vi "VR Controler 9.2.vi"() -> ()   [LabVIEW 2017]
uses:
  Sub VIs/Record enum.ctl
  Sub VIs/Socket enum.ctl
  Sub VIs/Main program enum2.ctl
  <vilib>/vision/Image Controls.llb/IMAQ Image.ctl
  e2139745-3a2d-4eca-8046-712b838de117.vi
  c1239b79-c935-4849-aa75-a73d195e7430.vi
  674a1914-568f-4f25-b0a8-01d8120e0c5f.vi
  5779e0b0-41b7-4506-a67f-138f79383ca8.vi
  75927e18-e53a-4ccd-922e-dca7ab16e00a.vi
  6c211394-beff-4d45-9cac-85fa7b8fa806.vi
  b426bb1a-86ec-4bb9-bfac-d02472307ceb.vi
  58126b9d-de85-4f5f-a9a7-01a9de38026e.vi
  6235507b-2202-4f21-86ca-b7b41428e472.vi
  835dcb76-40d0-41c5-8fe3-3989c1fd9891.vi
  7e58093c-c06d-4417-bc89-98900abbef57.vi
  280f3af5-b849-4305-b59e-3cd99654dfd1.vi
  378bb8a1-48c3-4ad7-89e2-98d14b258fa1.vi
  4796a129-a1f4-4c2b-9c8a-39875efc01cf.vi
  <vilib>/DAQmx/write.llb/DAQmx Write (Digital Bool 1Line 1Point).vi
  bf4008ee-ae26-4c0a-87de-22156137ce73.vi
  cfabecd4-7210-4e1d-87ea-acbfc879dca4.vi
  ec3ac053-eb45-4274-a63b-aef392164dd0.vi
  c7e8f878-57a8-404b-b967-73b810e59910.vi
  b14711bf-09ac-44ea-973e-d3b9cd6138c5.vi
  839eb35e-605d-4d61-b8d1-8b601b76a39a.vi
  1da1cb31-40b1-4a67-a7e6-56ad72bdf787.vi
  eb595f88-4225-414f-83f1-01d5d940fc66.vi
  fb6b5c9d-106e-453b-a883-cc93056fac18.vi
  4b664865-0372-4337-9de9-faa9f3913aab.vi
  63df5311-9246-4ffc-851f-b70ac2e65be5.vi
  <vilib>/DAQmx/read.llb/DAQmx Read (Analog 2D DBL NChan NSamp).vi
  <vilib>/DAQmx/read.llb/DAQmx Read (Digital 2D U8 NChan NSamp).vi
  <vilib>/DAQmx/read.llb/DAQmx Read (Counter 1D DBL 1Chan NSamp).vi
  <vilib>/DAQmx/create/channels.llb/DAQmx Create Channel (DO-Digital Output).vi
  <vilib>/Utility/file.llb/Read Delimited Spreadsheet (string).vi
  <vilib>/DAQmx/create/channels.llb/DAQmx Create Channel (AI-Voltage-Basic).vi
  <vilib>/DAQmx/create/channels.llb/DAQmx Create Channel (DI-Digital Input).vi
  <vilib>/DAQmx/configure/timing.llb/DAQmx Timing (Sample Clock).vi
  <vilib>/DAQmx/miscellaneous.llb/DAQmx Fill In Error Info.vi
  <vilib>/Utility/file.llb/Write Delimited Spreadsheet (string).vi
  <vilib>/DAQmx/create/channels.llb/DAQmx Create Channel (CO-Pulse Generation-Frequency).vi
  <vilib>/DAQmx/configure/timing.llb/DAQmx Timing (Implicit).vi
  6f1d6b9c-7e66-4bfa-a54a-0bf9111e914d.vi
  <resource>/objmgr/daqmx.rc
  f0a6b648-ccd6-4e98-b62c-d3930b5e7adb.vi
  <vilib>/vision/driver/NI_Vision_Acquisition_Software.lvlib
  fa866b4b-dc6c-4481-bc67-f1512cbbaaf9.vi
  <vilib>/DAQmx/configure/task.llb/DAQmx Configure Logging (TDMS).vi
panel:
  out "Write loop stopped":bool
  out "Read loop stopped":bool
  in  "VR Controller":T1(tab)
  in  "Timed reward (s)":u32
  in  "Various GUI elements":T2(tab)
  out "Saved 2P signals":string[][](table)
  in  "Record 2P":bool
  out "Frame signal 1 rec.":bool
  out "Frame signal 2 rec.":bool
  in  "Start trigger":bool
  in  "Stop triggers":bool
  out "Boolean 2":bool
  out "Boolean 3":bool
  out "Opt stim command":dbl[](graph)
  out "stim loop rate":dbl
  in  "start with ramp":bool
  out "Next trial stim. protocol":string
  out "Current stim. protocol":string
  in  "Stimulus cut off (s)":u32=15
  out "Laser ON":bool
  in  "Enable stim.":bool
  out "Saved optogen. signals":string[][](table)
  out "Pupille image saved":bool
  in  "Record Button 2":bool
  in  "Black Level":dbl(slide)=0.9896907216494839 min=-32.0 max=31.75 step=1.0 scale=-32.0..32.0
  in  "Gain":dbl(slide)=8.879999999999999 min=0.0 max=24.0 step=1.0 scale=0.0..24.0
  in  "Exposure Time (ms)":dbl(slide)=15144.329896907217 min=1.0 max=15.0 scale=0.0..15.0
  in  "Target frame rate":dbl=60.0 min=1.0 max=144.0 step=1.0
  out "Pupille image":T3(plugin-control)
  out "Frame rate":dbl
  in  "Image Format Control::Offset X":i64(slide) min=0 max=450 step=2 scale=0.0..450.0
  in  "Image Format Control::Offset Y":i64(slide) min=0 max=350 step=2 scale=0.0..350.0
  out "Lost Image Count":u32
  out "Total Images Transferred":u32
  out "Saved pupil imaging signals":string[][](table)
  out "EyeCam frame signal rec.":bool
  out "Security cam image":T3(plugin-control)
  in  "Cam ON /OFF":bool
  out "Random start pos":bool=TRUE
  in  "VR start pos":T4(ring)
  out "Behavior and VR signals saved":string[][](table)
  out "Stim. count":i32
  in  "Random reward":bool
  in  "Hybrid licking":bool
  in  "Boolean":bool
  in  "Comment":string
  out "Photodiode":bool
  out "Trial type ettings":enum32{"Page 1", "Page 2"}(tab)
  in  "Auto stop recording":bool
  in  "Shuffle stim trials":bool
  out "Session length":u16 max=100
  in  "Block num. 5":u16
  in  "Block 5":u16(ring) items=["Context J", "Context K (rew same as J)", "Context L", "Context M", "Context N (rew same as J)", "Context O"]
  in  "Block num. 4":u16
  in  "Block 4":u16(ring) items=["Context J", "Context K (rew same as J)", "Context L", "Context M", "Context N (rew same as J)", "Context O"]
  in  "Block num. 3":u16
  in  "Block 3":u16(ring) items=["Context J", "Context K (rew same as J)", "Context L", "Context M", "Context N (rew same as J)", "Context O"]
  in  "Block num. 2":u16
  in  "Block 2":u16(ring) items=["Context J", "Context K (rew same as J)", "Context L", "Context M", "Context N (rew same as J)", "Context O"]
  in  "Block num. 1":u16=1 min=1
  in  "Block 1":u16(ring) items=["Context J", "Context K (rew same as J)", "Context L", "Context M", "Context N (rew same as J)", "Context O"]
  in  "stim. num. 5":u16
  in  "Stim. prot 5":u16(ring) items=["none", "none", "continuous from 0 to 150 int. 100 % duty cycle 0 %", "20 Hz sinus from 0 to 150 int. 100 % duty cycle 0 %", "20 Hz sinus from 10 to 20 int. 100 % duty cycle 0 %", "20 Hz sinus from 10 to 70 int. 100 % duty cycle 0 %", "20 Hz sinus from 10 to 0 int. 100 % duty cycle 0 %", "20 Hz sinus from 0 to 70 int. 100 % duty cycle 0 %", "20 Hz sinus from 0 to 70 int. 50 % duty cycle 0 %", "continuous from 10 to 70 int. 100 % duty cycle 0 %"]
  in  "stim. num. 4":u16
  in  "Stim. prot 4":u16(ring) items=["none", "none", "continuous from 0 to 150 int. 100 % duty cycle 0 %", "20 Hz sinus from 0 to 150 int. 100 % duty cycle 0 %", "20 Hz sinus from 10 to 20 int. 100 % duty cycle 0 %", "20 Hz sinus from 10 to 70 int. 100 % duty cycle 0 %", "20 Hz sinus from 10 to 0 int. 100 % duty cycle 0 %", "20 Hz sinus from 0 to 70 int. 100 % duty cycle 0 %", "20 Hz sinus from 0 to 70 int. 50 % duty cycle 0 %", "continuous from 10 to 70 int. 100 % duty cycle 0 %"]
  in  "stim. num. 3":u16
  in  "Stim. prot 3":u16(ring) items=["none", "none", "continuous from 0 to 150 int. 100 % duty cycle 0 %", "20 Hz sinus from 0 to 150 int. 100 % duty cycle 0 %", "20 Hz sinus from 10 to 20 int. 100 % duty cycle 0 %", "20 Hz sinus from 10 to 70 int. 100 % duty cycle 0 %", "20 Hz sinus from 10 to 0 int. 100 % duty cycle 0 %", "20 Hz sinus from 0 to 70 int. 100 % duty cycle 0 %", "20 Hz sinus from 0 to 70 int. 50 % duty cycle 0 %", "continuous from 10 to 70 int. 100 % duty cycle 0 %"]
  in  "stim. num. 2":u16
  in  "Stim. prot 2":u16(ring) items=["none", "none", "continuous from 0 to 150 int. 100 % duty cycle 0 %", "20 Hz sinus from 0 to 150 int. 100 % duty cycle 0 %", "20 Hz sinus from 10 to 20 int. 100 % duty cycle 0 %", "20 Hz sinus from 10 to 70 int. 100 % duty cycle 0 %", "20 Hz sinus from 10 to 0 int. 100 % duty cycle 0 %", "20 Hz sinus from 0 to 70 int. 100 % duty cycle 0 %", "20 Hz sinus from 0 to 70 int. 50 % duty cycle 0 %", "continuous from 10 to 70 int. 100 % duty cycle 0 %"]
  in  "stim. num. 1":u16 min=1
  in  "Stim. prot 1":u16(ring) items=["none", "none", "continuous from 0 to 150 int. 100 % duty cycle 0 %", "20 Hz sinus from 0 to 150 int. 100 % duty cycle 0 %", "20 Hz sinus from 10 to 20 int. 100 % duty cycle 0 %", "20 Hz sinus from 10 to 70 int. 100 % duty cycle 0 %", "20 Hz sinus from 10 to 0 int. 100 % duty cycle 0 %", "20 Hz sinus from 0 to 70 int. 100 % duty cycle 0 %", "20 Hz sinus from 0 to 70 int. 50 % duty cycle 0 %", "continuous from 10 to 70 int. 100 % duty cycle 0 %"]
  out "Stim array length":u16 max=500
  in  "Masking light":T5(ring)
  out "GUI version":enum32{"Page 1", "Page 2"}(tab)
  in  "plot selector 1":u16(ring) items=["Context J", "Context K (rew same as J)", "Context L", "Context M", "Context N (rew same as J)", "Context O"]
  out "?":dbl(slide) scale=0.0..250.0
  in  "Reset top plot":bool=TRUE caption="Reset"
  in  "Reset bottom plot":bool=TRUE caption="Reset"
  out "P stim. Hit":dbl(slide) scale=0.0..1.0
  out "P ctrl. Hit":dbl(slide) scale=0.0..1.0
  out "Control hit trials %":dbl
  out "Stim. hit trials %":dbl
  out "Top Graph":cluster{"Y":dbl[], "Y":dbl[]}[](graph) caption="XY Graph"
  out "Bottom Graph":cluster{"Y":dbl[], "Y":dbl[]}[](graph) caption="XY Graph"
  in  "plot selector bool 1":bool
  in  "plot selector 2":u16(ring) items=["Context J", "Context K (rew same as J)", "Context L", "Context M", "Context N (rew same as J)", "Context O"]
  in  "plot selector bool 2":bool
  out "Hit trials %":dbl format="%#.1g"
  out "Hit trials":i32
  out "Wheel position graph":cluster{"Y":dbl[], "Y":dbl[]}[](graph) caption="XY Graph"
  in  "Reset wheel pos. graph":bool=TRUE caption="Reset"
  out "P hit trials":dbl(slide) scale=0.0..1.0
  out "%":dbl format="%#_3g"
  in  "Weight":dbl
  in  "Lab book notes":string
  in  "Open valve":bool
  in  "Reward freq. (cm)":u32
  in  "Reward zone":bool
  out "Distance (m)":dbl format="%#.2g"
  in  "Record Button":bool
  in  "Reset water count":bool
  out "Water received (ul)":dbl
  out "All trials":i32
  out "Ctrl. count":i32
  out "Unique ID":i8 format="%2d"
  in  "Stop recording":bool
  in  "Start recording":bool
  out "Laps":i32
  in  "Exit program":bool
  in  "counter reset (F)":bool caption="stop (F)"
  out "Position on the wheel":dbl(knob) scale=0.0..157.0
  in  "Give reward":bool
  in  "Repetition":i32
  out "Date":string
  out "Run experiment":bool
  out "Velocity chart":dbl(graph)
  out "Lick and reward chart":cluster{dbl, i16}(graph)
  out "Record":bool
  out "Time (min)":dbl format="%#.2g"
  in  "Active licking":bool
  in  "Mouse name":u16(ring) items=["-", "m8134-MN7", "m8135-NL1", "m8136-NL3", "m8137-MN8", "m8138-NL7", "m8139-X2", "m8140-MN6", "m8141-NL8", "m8142-NL6", "m8143-X", "m8144-NL4", "-", "-", "-", "-", "-", "test-xx", "train-NLX", "-"]
  out "Tab Control hidden Variables":enum32{"Test charts", "Variables"}(tab)
  in  "Ring 4":u16(ring) items=["Encoder signal", "Photo-diode", "Distance (cm)", "Position in Unity", "Valve open", "Lick signal", "Analog lick signal", "VR context", "VR gain", "Frame signal", "Frame signal 2", "EyeCam frame signal", "Analog input 3", "Photo stimulus signal", "Masking light signal", "Stimulus protocol", "Analog input 5"]
  out "Waveform Chart 4":dbl[](graph)
  in  "Ring 3":u16(ring) items=["Encoder signal", "Photo-diode", "Distance (cm)", "Position in Unity", "Valve open", "Lick signal", "Analog lick signal", "VR context", "VR gain", "Frame signal", "Frame signal 2", "EyeCam frame signal", "Analog input 3", "Photo stimulus signal", "Masking light signal", "Stimulus protocol", "Analog input 5"]
  out "Waveform Chart 3":dbl[](graph)
  in  "Ring 2":u16(ring) items=["Encoder signal", "Photo-diode", "Distance (cm)", "Position in Unity", "Valve open", "Lick signal", "Analog lick signal", "VR context", "VR gain", "Frame signal", "Frame signal 2", "EyeCam frame signal", "Analog input 3", "Photo stimulus signal", "Masking light signal", "Stimulus protocol", "Analog input 5"]
  out "Waveform Chart 2":dbl[](graph)
  in  "Ring":u16(ring) items=["Encoder signal", "Photo-diode", "Distance (cm)", "Position in Unity", "Valve open", "Lick signal", "Analog lick signal", "VR context", "VR gain", "Frame signal", "Frame signal 2", "EyeCam frame signal", "Analog input 3", "Photo stimulus signal", "Masking light signal", "Stimulus protocol", "Analog input 5"]
  out "Waveform Chart":dbl[](graph)
  in  "VR Gain":dbl
  out "Frame signal 2":i8[](array[numeric])
  out "corridor lengths":i32[](array[numeric])
  out "zeward zones":i16[][](array[numeric])
  out "teleports":i16[](array[numeric])
  out "Stim prot command":u16
  out "Context command":u16
  out "ML signal":sgl[](array[numeric])
  out "Pupil Exp day folder":path
  out "settings folder":path
  out "Eyecam states":T6(ring)
  in  "Eable security cam":bool
  out "Eye cam frame signal":i8[](array[numeric])
  out "prev. max stim. V":dbl
  out "prev. stim. type":string
  out "protocol array":string[][](array[string])
  out "analog lick":sgl[](array[numeric])
  out "Encoder signal":sgl[](array[numeric])
  out "Photo stimulus signal":sgl[](array[numeric])
  out "SciScan start":refnum<k21>
  out "Valve signal":i8[](array[numeric])
  out "Trials in session array":u16[][](array[numeric])
  out "Photodiode signal":sgl[](array[numeric])
  out "Frame signal":i8[](array[numeric])
  out "Filename":string
  out "Lab book file":path
  out "Lick indicator":dbl
  out "Encoder count":dbl
  out "Last saved reward size":dbl
  out "Stim types":u16[](array[numeric])
  out "shuffled array":i16[](array[numeric])
  out "Record loop state":T7
  in  "Record enum":T7
  out "Wheel circumference":dbl
  in  "Recording folder":path
  in  "command line":string
  in  "working directory":path=path ""
  out "Start time":u32
  out "Experiment time (ms)":u32
  out "delta time (s)":dbl format="%#.8g"
  out "reward zone end":dbl
  out "Sample rate":dbl
  out "Loop rate":dbl
  out "No. of smpl. per ch.":i32
  out "Original weight":dbl
  out "Laser stimulus calibration":string
  out "Stimulus protocol":string
  out "prev. diode position":dbl
  out "encoder ticks per rev":dbl
  out "Prev. rew. pos.":dbl
  out "Distance (cm)":dbl
  out "miss trial":bool
  out "Session start:":string
  out "hit trial":bool
  out "2P imaging":string
  out "Security camera":string
  out "velocity (cm/s)":dbl
  out "Masking light prot":string
  out "offset tag":string
  out "random rew":dbl
  out "Track position":sgl
  out "start of stim":bool
  in  "Eable eye cam":bool
  out "stim started":bool
  out "Context types":u16[](array[numeric])
  out "Reward given":u32
  out "current VR context":u16
  out "RZ available":bool
  out "User profile":string
  out "Stop Unity":bool
  out "Exit":bool
  out "Stim trial":bool
  out "Trial counted":bool
  in  "select trial":bool
  in  "VR Mode":bool
  out "delta distance cm":dbl[](array[numeric])
  in  "index":i32
  out "lick signal":i8[](array[numeric])
  out "msg tag":string
  out "Header":string
  out "Unity connected":bool
  out "Masking light":bool
  out "Lick":bool
  out "Valve open":bool
  in  "sound cue presented":bool
  out "read":bool
  out "Write":bool
  out "My tdms file":refnum<k34>
  out "Water cnt. reset":i32
  out "Store prev encoder count":dbl
  out "Start mask stim":bool
  out "Start light stim":bool
  out "Stop light stim":bool
  out "Light ON":bool
  out "Stop mask stim":bool
  out "Hit trials stim.":i32
  out "Hit trials ctrl.":i32
  in  "Software version":string
  out "total distance cm":sgl[](array[numeric])
  out "Experiment time (s)":dbl
  out "Analog 3":sgl[](array[numeric])
  out "Analog 5":sgl[](array[numeric])
  out "Signals to delete":i32[](array[numeric])
  out "channel names":string[](array[string])
  in  "working directory 2":path=path ""
  out "Mouse name 2":string
  out "Task config":string
  out "Saved signals":string
  out "Default vars text":string
  in  "Duty cycle (%)":u8=50 max=100 step=1
  out "Last calibration":string
  in  "Edit mouse list":bool
  out "Socket read loop rate (ms)":u32(graph)
  out "Recording loop rate  (ms)":u32(graph)
  in  "Sound duration (ms)":u32=25
  in  "Valve open dur. (ms)":u32=25
  in  "Reward size (ul)":dbl min=0.0 step=inf format="%#.2g"
  out "Reward read loop rate (ms)":u32(graph)
  in  "Current mice":string[][](array[string])
  out "Water count":i32
  in  "Stim protocols":u16(ring) items=["none", "none", "continuous from 0 to 150 int. 100 % duty cycle 0 %", "20 Hz sinus from 0 to 150 int. 100 % duty cycle 0 %", "20 Hz sinus from 10 to 20 int. 100 % duty cycle 0 %", "20 Hz sinus from 10 to 70 int. 100 % duty cycle 0 %", "20 Hz sinus from 10 to 0 int. 100 % duty cycle 0 %", "20 Hz sinus from 0 to 70 int. 100 % duty cycle 0 %", "20 Hz sinus from 0 to 70 int. 50 % duty cycle 0 %", "continuous from 10 to 70 int. 100 % duty cycle 0 %"]
  in  "Stim type":u16(ring) items=["none", "10 Hz sinus", "20 Hz sinus", "40 Hz sinus", "continuous", "10 Hz square", "20 Hz square", "40 Hz square"]
  in  "Intensity (%)":u8=100 max=100 step=1
  in  "stop (cm)":i32
  in  "start (cm)":i32
  in  "Select user profile":string(combo)
  in  "Default var. edit":string[][](array[string])
  in  "Path 2":path
  in  "Path":path
  out "Default variables":string[](array[string])
  out "Imaging ralated signals":string[](array[string])=["Encoder signal", "Photo-diode", "Distance (cm)", "Photo stimulus signal", "Position in Unity", "Valve open", "Lick signal", "Frame signal", "Stimulus protocol", "VR context", "Analog lick signal", "EyeCam frame signal", "Masking light signal", "Frame signal 2"]
  out "Behavior and task related signals":string[](array[string])=["Encoder signal", "Photo-diode", "Distance (cm)", "Photo stimulus signal", "Position in Unity", "Valve open", "Lick signal", "Frame signal", "Stimulus protocol", "VR context", "Analog lick signal", "EyeCam frame signal", "Masking light signal", "Frame signal 2"]
  out "Optogenetics related signals":string[](array[string])=["Encoder signal", "Photo-diode", "Distance (cm)", "Photo stimulus signal", "Position in Unity", "Valve open", "Lick signal", "Frame signal", "Stimulus protocol", "VR context", "Analog lick signal", "EyeCam frame signal", "Masking light signal", "Frame signal 2"]
  in  "Save":bool[](array[boolean])
  in  "Save 2":bool[](array[boolean])
  in  "Save 3":bool[](array[boolean])
  in  "Task configuration":string[][](array[string])
  in  "Save and exit":bool
  # "All"
  # "This session"
  # "Reward conditions"
  # "recording"
  # "recording"
  # "(Default)"
  # "To use 2P recording at least 1 frame \nsignal have to be saved. To edit signals \nto be saved please use the signal \nconfigurations VI."
  # "recording"
  # "ScanImage stops more reliably with extra stop triggers"
  # "Requirements to use optogenetics:  \n1) The stimulus signal have to be saved. \nTo edit  signals to be saved please use the signal configurations VI.\n\n2) \"Laser stimulus calibration.txt\" file in the user profile folder. Please use the Calibrate photo-stimulation VI to calibrate command voltage."
  # "To record pupil image the frame signal have to be \nsaved. To edit  signals to \nbe saved please use the \nsignal configurations VI."
  # "To edit signals to be saved please \nuse the signal configurations VI."
  # "Trial type settings"
  # "Hit trials:"
  # "%"
  # "Hit trials:"
  # "%"
  # "%"
  # "Edit stimulus protocols for photo stimulation. Chose a protocol from the list and define parameters."
  # "Mouse name               Headbar           Original weight"
  # "Reward settings"
  # "Test charts are not available in recording mode."
  # "Note: \nThese variables are used during the startup of the program. To save and activate any changes the program needs to be restarted. Press the Save and Exit button!"
  # "P0.5"
  # "Dev1/ctr0"
  # "P0.3"
  # "AI 4"
  # "AI 1"
  # "Calculated in LV"
  # "AI 3"
  # "Feedback from Unity"
  # "P0.6"
  # "P0.4"
  # "AI 0"
  # "AI 6"
  # "AI 2"
  # "LV command"
  # "LV command"
  # "LV command"
  # "AI 5"
  # "Context name"
  # "Corridor length"
  # "Teleport point"
  # "Rew. zone 1 start"
  # "Rew. zone 1 end"
  # "Rew. zone 2 start"
  # "Rew. zone 2 end"
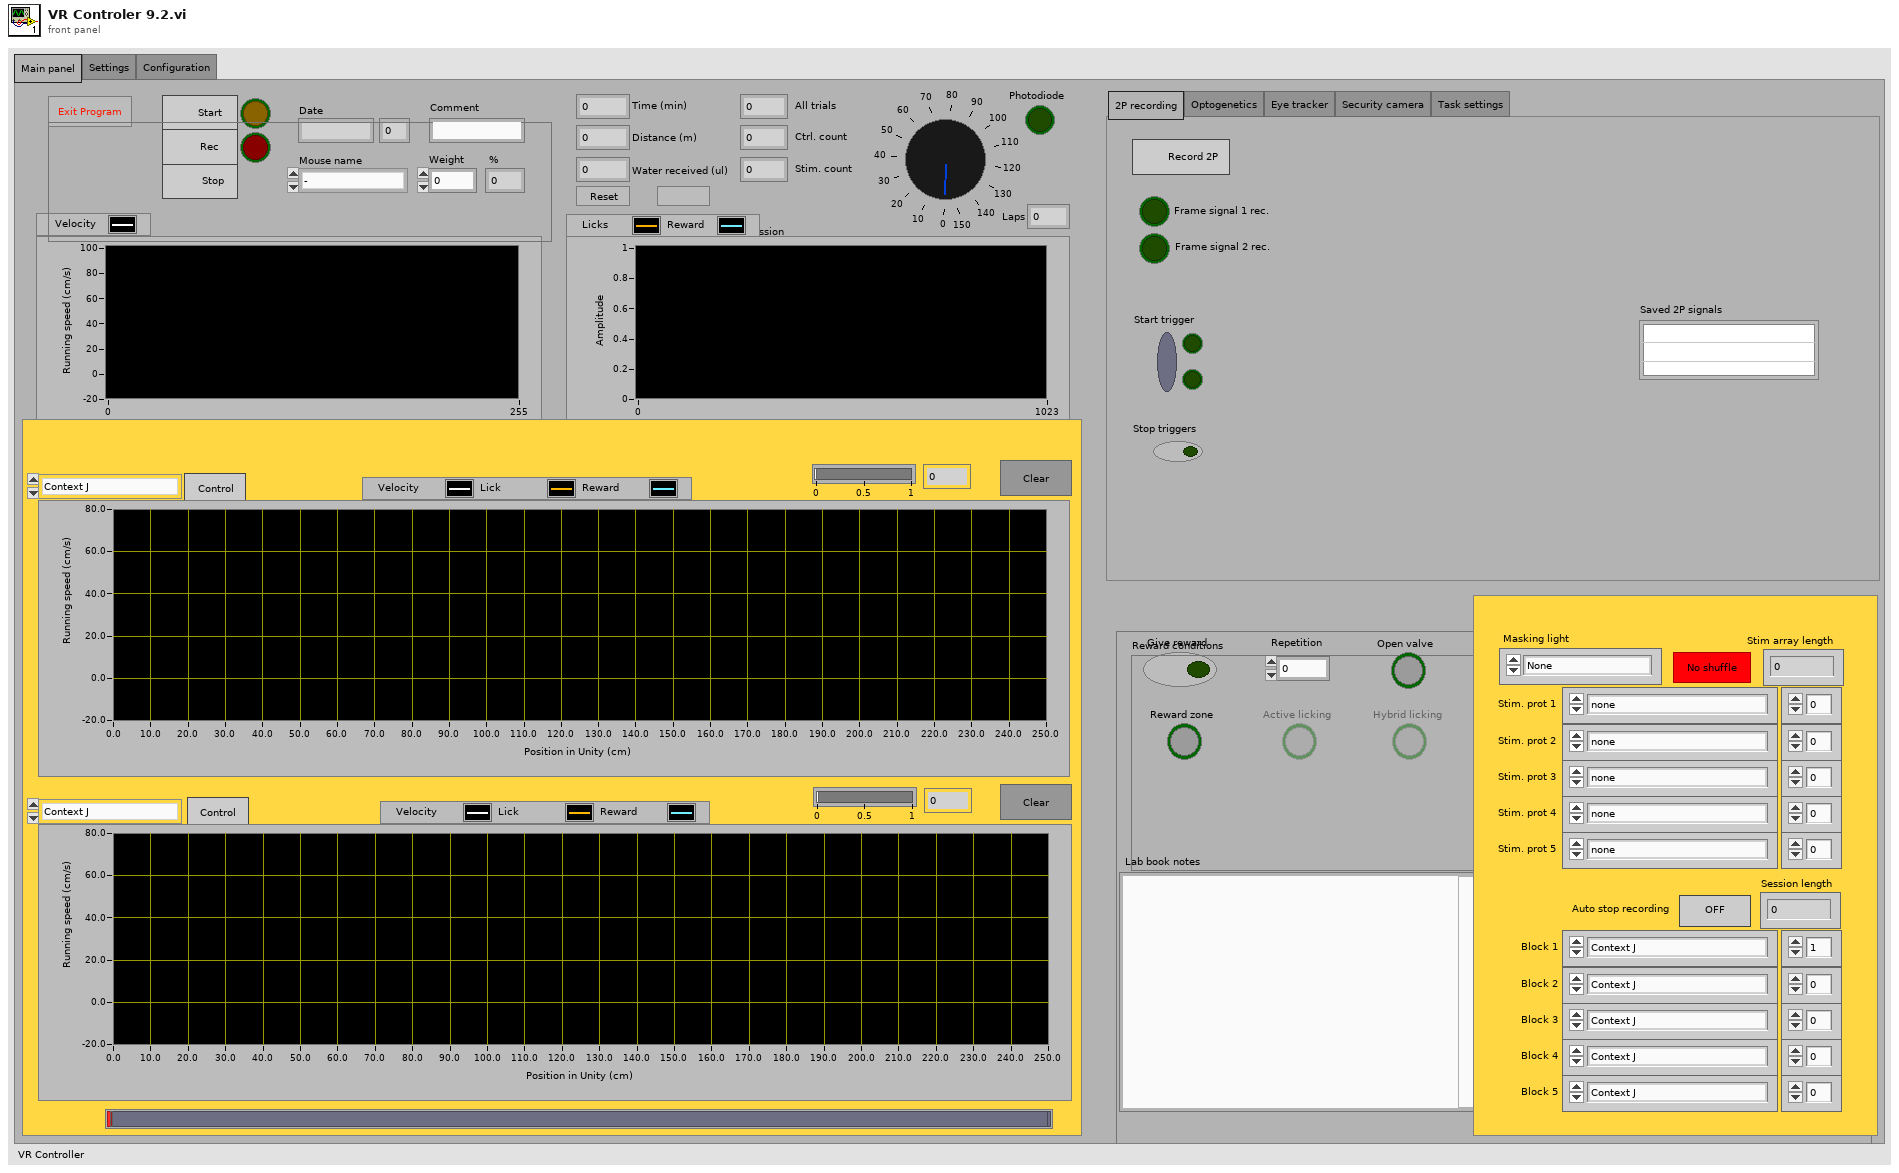
[diagram p1: front panel]
types:
  T1 = enum32{"Main panel", "Settings", "Configuration"}
  T2 = enum32{"2P recording", "Optogenetics", "Eye tracker", "Security camera", "Task settings"}
  T3 = typedef "IMAQ Image.ctl" = refnum<image>
  T4 = enum16{"Random of 4", "Random of 2", "Non-random"}
  T5 = enum16{"None", "20 Hz until reward ", "Continuous specified light off trials", "Continuous specified all trials", "20 Hz specified light off trials", "20 Hz specified all trials", "20 Hz full trial", "Continuous full trial"}
  T6 = enum16{"Idle", "Set params", "Start recording", "Record pupille", "Stop recording"}
  T7 = typedef "Record enum.ctl" = enum16{"Idle", "Init recording", "Init data acquisition", "Record VR", "Record", "Stop data acquision"}
  T8 = enum8{"Enabled", "Disabled", "Disabled and Grayed Out"}
  T9 = enum16{"open", "replace", "create", "open or create", "replace or create", "replace or create with confirmation"}
  T10 = typedef "Main program enum2.ctl" = enum16{"Init program", "Idle", "Init recording ", "Record", "Record VR", "Stop Recording", "Exit program"}
  T11 = typedef "Socket enum.ctl" = enum16{"Socket not connected", "Init socket", "Socket connected", "Close socket"}
  T12 = cluster{"Type":u32, "Version":u32, "Flags":u32, "SerialNumberHigh":u32, "SerialNumberLow":u32, "BusType":u32, "InterfaceName":string, "VendorName":string, "ModelName":string, "CameraFileName":string, "CameraAttributeURL":string}[]
  T13 = enum16{"Init program", "Idle", "Init recording ", "Record", "Record VR", "Stop Recording", "Exit program"}
  T14 = enum16{"None", "20 Hz until reward ", "Continuous specified light off trials", "Continuous specified all trials", "20 Hz specified light off trials", "20 Hz specified all trials"}
  T15 = enum16{"None", "Full trial 40 Hz sinus ", "Full trial 20 Hz sinus", "Continuous light ON", "Until reward 40 Hz sinus"}
  T16 = typedef "LVStringsAndValuesArrayTypeDef_U16.ctl" = cluster{"String":string, "Value":u16}[]
  T17 = enum16{"open", "open or create", "create or replace", "create", "open (read-only)"}
  T18 = enum16{"Standard", "Buffered", "CRLF", "Immediate"}
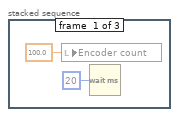
[diagram p2: hidden frame]
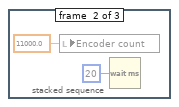
[diagram p3: hidden frame]
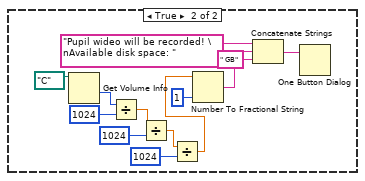
[diagram p7: hidden frame]
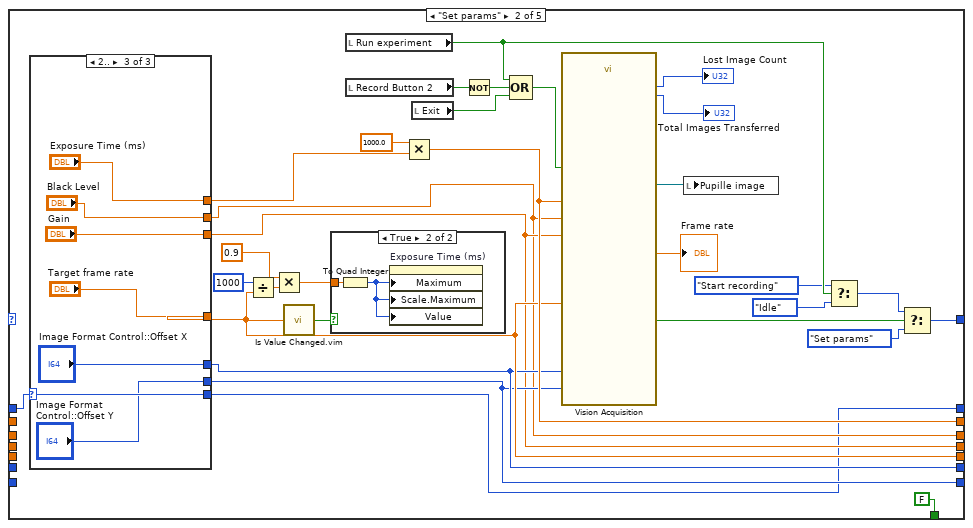
[diagram p8: hidden frame]
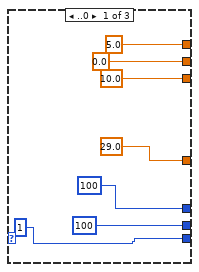
[diagram p9: hidden frame]
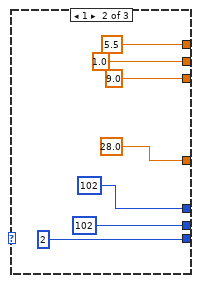
[diagram p10: hidden frame]
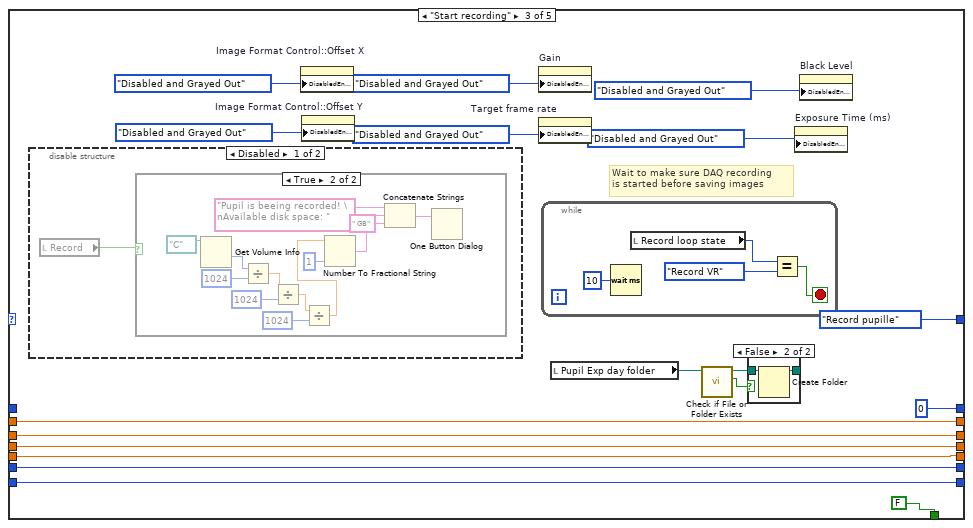
[diagram p12: hidden frame]
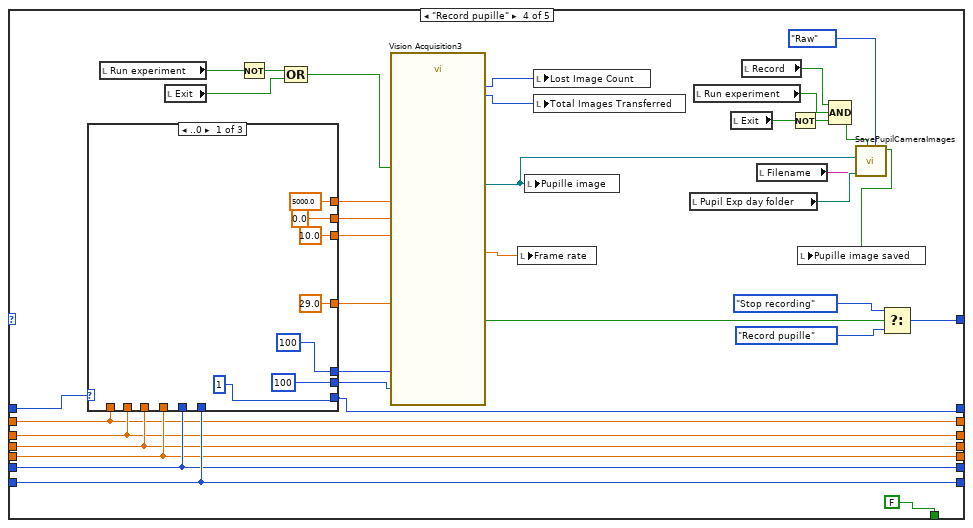
[diagram p16: hidden frame]
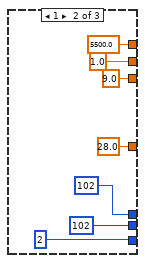
[diagram p17: hidden frame]
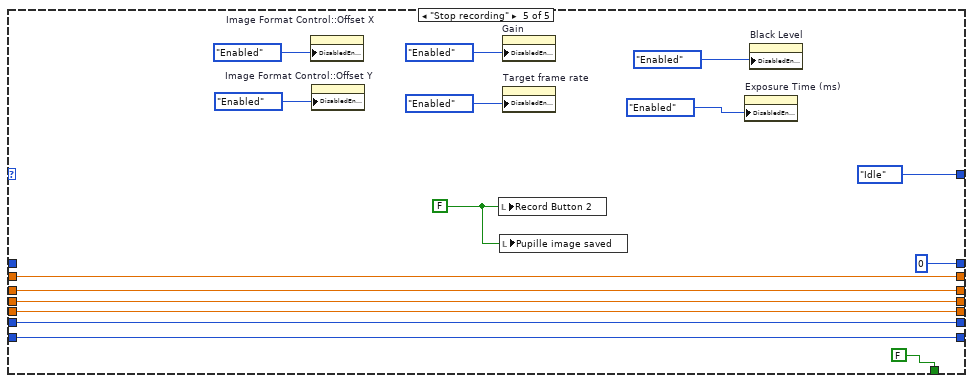
[diagram p19: hidden frame]
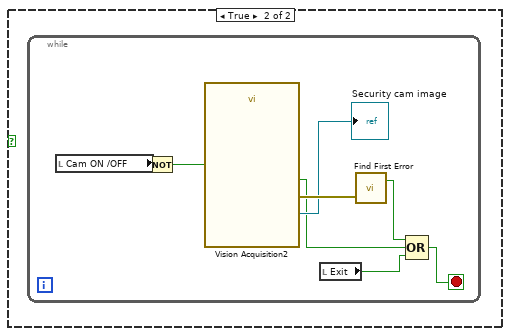
[diagram p20: hidden frame]
diagram:
  (unwired) string[] ["Photodiode signal", "Track position", "Valve signal", "Lick signal (digital)", "Lick signal (analog)", "VR gain", "Frame signal ", "Frame signal 2", "Pupilcam frame signal", "Analog input 3", "Photo stimulus signal", "ML signal", "Analog input 5"] ("Strings []")
  w7 = 0
  w10 = 0
  w19 = T8."Enabled" ("Disabled")
  w29 = FALSE ("Eable eye cam")
  w30 = FALSE ("Record Button 2")
  w31 = 60 ("y")
  (unwired) string[] ["Photo-diode", "Time (s)", "Delta Time (ms)", "Distance (cm)", "Valve open", "Frame signal", "Lick signal", "Photo stimulus signal", "Laser ON", "Position in Unity", "Corridor indicator"] ("channel name(s) in (Untitled)")
  w44 = FALSE ("Reset")
  # "Defaults"
  # "Keep order of default variables:\nUser:\tMate\nLoop rate:\t100\nSampling rate:\t3000\nEncoder tisks:\t4000\nRecording folder:\tC:\\Users\\vrsetup\\Desktop\nEnable VR more(Y/N):\tY\n..."
  # "File versions:\n-8.5 User profile selector\n\n-8.3 Camera control added> Pupil imaging and security camera\nTimed reward\n\n-8.2 with 8.4 unity version: \nNew task without cue\nImportant bugfixes in photo-stimulation, start stimulus with ramp option is added\nSafety switch shuts off stimulus after 10s \n\n-8.0 - 8.2\nNew task wersionm new optogenetic prorocol solutions\n\n-7.5 - 2019.07.10\nRandom reward option\n\n-7.5\nNew Unity version: coupling error is corrected! (interpolation factor discarded), randomizeable starting point.\nTiki-taka task for Nora\nNew masking light functions : 20Hz specified in light off or all trials\n\n\n-7.3\nMasking light options are added\nMasking light protocol is saved now in labbook\n\n-7.2\nmade GitHub compatible: folder path and some default variables are red from txt file and txt data files are now in separate folder\ndate is formated with different method\n\n-7.1\nsaves Encoder signal and imaging/security camera YES NO indication is added to lab book\nsaves Analog lick signal\n\n-7.0 \nMasking light\n\n-6.9\nData typed are changed back to DBL\n\n-6.8\nDifferent data saving settings to reduce file size by specifying data types\nCorrect trial % corrected after 2018.12.05\nHybrid licking\nPhoto stimulus trials and counting of \"Hit trials \"for Nora\n\n-6.7 \nfor Mate Loop rate from 200 -> 100 Hz  (should not affect VR that is 60 Hz) \nrecorded sampling rate increased 200 -> 3000 Hz\nswitch to show water consumption in current session is added\n\n\n\n..."
  n1 = flat-sequence {
    tunnel: [w86] -> w25
    tunnel: w25 -> [w144]
    tunnel: [w144] -> w1
    tunnel: [Socket_enum."Socket not connected" ("Enum")] -> w76
    tunnel: [Main_program_enum2."Init program" ("main program")] -> w75
    tunnel: [Record_enum."Idle" ("Record enum")] -> w72
    tunnel: [TRUE ("VR Mode")] -> _
    frame #0 {
      # "Select user profile"
      n2 = call <vilib>:"Recursive File List.vi"("Folder Path"=path "C:/VR Controller/data" ("path")) -> ("All Folders"=w100:path[])  [unwired: 6 in, 4 out]
      n3 = Array Size(array=w100) -> (size(s)=w104:i32)
      n4 = for {
        N: w104 -> [_]
        tunnel: w100 -> [w143] mode=indexing
        shift-right: [w140] -> w101
        shift-left: string[] [] -> [w139]
        i -> [w141]
        n5 = Strip Path(path=w143) -> (name=w142:string)  [unwired: 1 out]
        n6 = Insert Into Array(array=w139, index=w141, new element=w142) -> (w140:string[])
      }
      n7 = Array Size(array=w101) -> (size(s)=w95:i32)
      n8 = Greater?(x=w95, y=1) -> (0:w93:bool)
      n9 = Array Subset(array=w101, index=1, length=w95) -> (w81:string[])
      n10 = case shown="True" w93 {
        tunnel: w81 -> [_ w138]
        tunnel: w100 -> [_ w137]
        tunnel: [path "" ("path") w134] -> w80
        frame False {
        }
        frame True {
          n11 = call "Get User Input.vi"("Strings []"=w138) -> ("user"=w136:u16)  [unwired: 1 in, 9 out]
          n12 = Increment(x=w136) -> (x+1=w135:u16)
          n13 = Index Array(array=w137, index=w135) -> (element=w134:path)
        }
      }
      n14 = property on="Select user profile" class="CmbBox"("Strings[]"=w81) -> ()  [unwired: 2 in, 2 out]
      n15 = Strip Path(path=w80) -> (name=w79:string)  [unwired: 1 out]
      n16 = property on="Select user profile" class="CmbBox"("Value"=w79) -> ()  [unwired: 2 in, 2 out]
      n17 = Equal?(x=w80, y=path "" ("path")) -> (x = y?=w98:bool)
      n18 = Select(t=path "C:/VR Controller/data", s=w98, f=w80) -> (s? t:f=w86:path)
      "settings folder" <- w86
      n19 = Build Path(base path=w86, name or relative path="Data saving config.txt") -> (appended path=w88:path)
      n20 = call <vilib>:"Check if File or Folder Exists.vi"("path"=w88) -> ("file or folder exists?"=w87:bool)  [unwired: 8 in, 2 out]
      n21 = case shown="True" w87 {
        tunnel: [w119 w129] -> w83
        tunnel: w88 -> [_ w124]
        frame False {
          n22 = for {
            N: 17 -> [_]
            shift-right: [w121] -> w119
            shift-left: i32[] [] -> [w122]
            n23 = Build Array (concatenate)(w122, 1 ("index")) -> (w121:i32[])
          }
          n24 = local write "Saved signals"("Signal saving has not been concigured. All available signals are saved." ("Saved signals")) -> ()
          n25 = One Button Dialog(message="Data signal saving have not yet been configured for this user profile (Optional). Please find the options on the \"Configuration\" tab to avoid saving unused data channels!") -> ()  [unwired: 1 in, 1 out]
        }
        frame True {
          n26 = call-poly <vilib>:"Read Delimited Spreadsheet.vi"("file path (dialog if empty)"=w124) -> ("all rows"=w132:string[][])  [unwired: 9 in, 5 out]
          n27 = Open/Create/Replace File(file path (use dialog)=w124, operation (0:open)=T9."open", access (0:read/write)=enum16{"read/write", "read-only", "write-only"}."read-only") -> (refnum out=w128:refnum<file>)  [unwired: 3 in, 2 out]
          n28 = Read from Text File(file (use dialog)=w128) -> (refnum out=w127:refnum<file>, text=→"Saved signals":string)  [unwired: 3 in, 2 out]
          n29 = Index Array(array=w132, index (col)=1 ("disabled index (col)")) -> (element=w130:string[])  [unwired: 1 in]
          n30 = Close File(refnum=w127) -> ()  [unwired: 1 in, 2 out]
          n31 = Decimal String To Number(string=w130) -> (number=w129:i32[])  [unwired: 2 in, 1 out]
        }
      }
      n32 = for {
        tunnel: w83 -> [w110] mode=indexing
        shift-right: [w106] -> w85
        shift-left: i32[] [] -> [w105]
        i -> [w107]
        n33 = Equal?(x=w110, y=0) -> (x = y?=w108:bool)
        n34 = case shown="True" w108 {
          tunnel: w107 -> [_ w114]
          tunnel: [w111 w113] -> w106
          tunnel: w105 -> [w111 w112]
          frame False {
          }
          frame True {
            n35 = Build Array (concatenate)(w112, w114) -> (w113:i32[])
          }
        }
      }
      n36 = Path To String(path=w86) -> (string=w92:string)
      n37 = Reverse 1D Array(array=w85) -> (reversed array=→"Signals to delete":i32[])
      n38 = Match Pattern(string=w92, regular expression="data\\") -> (after substring=→"User profile":string)  [unwired: 1 in, 3 out]
    }
    frame #1 {
      w164 = 1 ("length")
      w169 = 1 ("length")
      w182 = 1 ("length")
      w185 = 1 ("length")
      w188 = 1 ("length")
      w191 = 1 ("length")
      # "VI version"
      # "Enable VR mode"
      n39 = Build Path(base path=w144, name or relative path="Default variables.txt") -> (appended path=w146:path)
      n40 = call-poly <vilib>:"Read Delimited Spreadsheet.vi"("file path (dialog if empty)"=w146) -> ("all rows"=w160:string[][])  [unwired: 9 in, 5 out]
      n41 = Array Subset(array=w160, index (row)=0 ("index"), length (row)=w191, index (col)=w191, length (col)=w191) -> (w190:string[][])
      n42 = Array Subset(array=w160, index (row)=1 ("index"), length (row)=w188, index (col)=w188, length (col)=w188) -> (w189:string[][])
      n43 = Array Subset(array=w160, index (row)=2 ("index"), length (row)=w169, index (col)=w169, length (col)=w169) -> (w166:string[][])
      n44 = Array Subset(array=w160, index (row)=3 ("index"), length (row)=w185, index (col)=w185, length (col)=w185) -> (w184:string[][])
      n45 = Array Subset(array=w160, index (row)=4 ("index"), length (row)=w182, index (col)=w182, length (col)=w182) -> (w183:string[][])
      n46 = Array Subset(array=w160, index (row)=5 ("index"), length (row)=w164, index (col)=w164, length (col)=w164) -> (w163:string[][])
      n47 = Concatenate Strings(w190) -> (w176:string)
      n48 = Concatenate Strings(w189) -> (w178:string)
      n49 = Concatenate Strings(w166) -> (w170:string)
      n50 = Concatenate Strings(w184) -> (w179:string)
      n51 = Concatenate Strings(w183) -> (w180:string)
      n52 = Concatenate Strings(w163) -> (w162:string)
      n53 = String To Path(string=w180) -> (path=w155:path)
      n54 = Fract/Exp String To Number(string=w170) -> (number=w167:dbl)  [unwired: 3 in, 1 out]
      n55 = Fract/Exp String To Number(string=w179) -> (number=w174:dbl)  [unwired: 3 in, 1 out]
      n56 = Fract/Exp String To Number(string=w178) -> (number=w175:dbl)  [unwired: 3 in, 1 out]
      n57 = Equal?(x=w176, y=" ") -> (x = y?=w153:bool)
      n58 = Equal?(x=w162, y="Y") -> (x = y?=w152:bool)
      n59 = case shown="True" w152 {
        tunnel: w160 -> [_ w200]
        tunnel: [path "" w203] -> w154
        frame False {
          (unwired) FALSE ("T button?")
        }
        frame True {
          w201 = 1 ("length")
          w207 = 1 ("length")
          # "Default context"
          n60 = Array Subset(array=w200, index (row)=6 ("index"), length (row)=w207, index (col)=w207, length (col)=w207) -> (w205:string[][])
          n61 = Array Subset(array=w200, index (row)=7 ("index"), length (row)=w201, index (col)=w201, length (col)=w201) -> (w199:string[][])
          n62 = Concatenate Strings(w205) -> (w204:string)
          n63 = Concatenate Strings(w199) -> (w198:string)
          n64 = local write "command line"(w204) -> ()
          n65 = String To Path(string=w204) -> (path=w203:path)
          n66 = Decimal String To Number(string=w198) -> (number=w197:i32)  [unwired: 2 in, 1 out]
          n67 = local write "Block 1"(w197) -> ()
          n68 = local write "plot selector 1"(w197) -> ()
        }
      }
      n69 = local write "Loop rate"(w175) -> ()
      n70 = local write "Sample rate"(w167) -> ()
      n71 = local write "encoder ticks per rev"(w174) -> ()
      n72 = local write "Recording folder"(w155) -> ()
      n73 = case shown="True" w153 {
        frame False {
          n74 = local write "Sound duration (ms)"(u32 0 ("Sound duration (ms)")) -> ()
        }
        frame True {
          n75 = local write "Sound duration (ms)"(u32 0 ("Sound duration (ms)")) -> ()
        }
      }
      n76 = Open/Create/Replace File(file path (use dialog)=w146, operation (0:open)=T9."open", access (0:read/write)=enum16{"read/write", "read-only", "write-only"}."read-only") -> (refnum out=w147:refnum<file>)  [unwired: 3 in, 2 out]
      n77 = Read from Text File(file (use dialog)=w147) -> (refnum out=w148:refnum<file>, text=→"Default vars text":string)  [unwired: 3 in, 2 out]
      n78 = Close File(refnum=w148) -> ()  [unwired: 1 in, 2 out]
      n79 = local write "VR Mode"(w152) -> ()
      n80 = Current VI's Path() -> (path=w158:path)
      n81 = case shown="True" TRUE {
        tunnel: [enum32{"Page 1", "Page 2"}."Page 2" ("GUI version") w230] -> w194
        tunnel: [enum32{"Page 1", "Page 2"}."Page 1" ("GUI version") w230] -> w193
        frame False {
          n82 = property on="Lick and reward chart" class="WFChart (strict)"("Visible"=FALSE, "DisabledEnum"=T8."Disabled" ("Disabled")) -> ()  [unwired: 2 in, 2 out]
          n83 = property on="Velocity chart" class="WFChart (strict)"("Visible"=FALSE, "DisabledEnum"=T8."Disabled" ("Disabled")) -> ()  [unwired: 2 in, 2 out]
          n84 = property on="Top Graph" class="XYGraph (strict)"("DisabledEnum"=T8."Disabled" ("Disabled")) -> ()  [unwired: 2 in, 2 out]
          n85 = property on="Bottom Graph" class="XYGraph (strict)"("DisabledEnum"=T8."Disabled" ("Disabled")) -> ()  [unwired: 2 in, 2 out]
          n86 = property on="Wheel position graph" class="XYGraph (strict)"("DisabledEnum"=T8."Enabled" ("Disabled")) -> ()  [unwired: 2 in, 2 out]
          n87 = property on="Reset top plot" class="Bool (strict)"("DisabledEnum"=T8."Disabled" ("Disabled")) -> ()  [unwired: 2 in, 2 out]
          n88 = property on="Reset wheel pos. graph" class="Bool (strict)"("DisabledEnum"=T8."Enabled" ("Disabled")) -> ()  [unwired: 2 in, 2 out]
          n89 = property on="Reset bottom plot" class="Bool (strict)"("DisabledEnum"=T8."Disabled" ("Disabled")) -> ()  [unwired: 2 in, 2 out]
        }
        frame True {
          w230 = enum32{"Page 1", "Page 2"}."Page 1" ("GUI version")
          n90 = property on="Top Graph" class="XYGraph (strict)"("DisabledEnum"=T8."Enabled" ("Disabled")) -> ()  [unwired: 2 in, 2 out]
          n91 = property on="Bottom Graph" class="XYGraph (strict)"("DisabledEnum"=T8."Enabled" ("Disabled")) -> ()  [unwired: 2 in, 2 out]
          n92 = property on="Lick and reward chart" class="WFChart (strict)"("Visible"=TRUE, "DisabledEnum"=T8."Enabled" ("Disabled")) -> ()  [unwired: 2 in, 2 out]
          n93 = property on="Wheel position graph" class="XYGraph (strict)"("DisabledEnum"=T8."Disabled" ("Disabled")) -> ()  [unwired: 2 in, 2 out]
          n94 = property on="Velocity chart" class="WFChart (strict)"("Visible"=TRUE, "DisabledEnum"=T8."Enabled" ("Disabled")) -> ()  [unwired: 2 in, 2 out]
          n95 = property on="Reset top plot" class="Bool (strict)"("DisabledEnum"=T8."Enabled" ("Disabled")) -> ()  [unwired: 2 in, 2 out]
          n96 = property on="Reset wheel pos. graph" class="Bool (strict)"("DisabledEnum"=T8."Disabled" ("Disabled")) -> ()  [unwired: 2 in, 2 out]
          n97 = property on="Reset bottom plot" class="Bool (strict)"("DisabledEnum"=T8."Enabled" ("Disabled")) -> ()  [unwired: 2 in, 2 out]
        }
      }
      "GUI version" <- w194
      "Trial type ettings" <- w193
      n98 = Strip Path(path=w154) -> (name=w156:string)  [unwired: 1 out]
      n99 = Strip Path(path=w158) -> (name=w157:string)  [unwired: 1 out]
      n100 = disable-structure shown="Disabled" {
        frame Disabled {
          n101 = local write "command line"("C:\\VR Controller\\corridor1\\LVcontrol_6.exe" ("command line")) -> ()
        }
        frame Enabled {
        }
      }
      n102 = case shown="True" w152 {
        tunnel: ["" ("string") w210] -> w172
        tunnel: w156 -> [_ w209]
        frame False {
        }
        frame True {
          n103 = Concatenate Strings(";    Unity VR version: " ("string"), w209) -> (w210:string)
        }
      }
      n104 = Concatenate Strings(w157, w172, "" ("string")) -> (w173:string)
      n105 = local write "Software version"(w173) -> ()
    }
    frame #2 {
      # "Has to be integer!"
      n106 = call <vilib>:"IMAQdx Enumerate Cameras.vi"() -> ("Camera Information Array"=w240:T12)  [unwired: 10 in, 1 out]
      n107 = local read "Sample rate"() -> (w239:dbl)
      n108 = for {
        tunnel: w240 -> [w252] mode=indexing
        # "Eye camera available"
        # "Security camera available"
        n109 = Unbundle By Name(w252) -> ("VendorName"=w249:string)
        n110 = Equal?(x="Microsoft® LifeCam Studio(TM)", y=w249) -> (x = y?=w247:bool)
        n111 = Equal?(x=w249, y="Basler") -> (x = y?=w248:bool)
        n112 = case shown="True" w247 {
          selector: w247 -> [_ w253]
          frame False {
          }
          frame True {
            n113 = local write "Eable security cam"(w253) -> ()
            n114 = property on="Cam ON /OFF" class="Bool (strict)"("DisabledEnum"=T8."Enabled" ("Disabled")) -> ()  [unwired: 2 in, 2 out]
          }
        }
        n115 = case shown="True" w248 {
          selector: w248 -> [_ w255]
          frame False {
          }
          frame True {
            n116 = local write "Eable eye cam"(w255) -> ()
            n117 = property on="Record Button 2" class="Bool (strict)"("DisabledEnum"=T8."Enabled" ("Disabled")) -> ()  [unwired: 2 in, 2 out]
          }
        }
      }
      n118 = local read "Loop rate"() -> (w243:dbl)
      n119 = Divide(x=w239, y=w243) -> (x/y=w244:dbl)
      n120 = Divide(x=1.0, y=w239) -> (x/y=w237:dbl)
      n121 = local write "No. of smpl. per ch."(w244) -> ()
      n122 = property on="Opt stim command" class="WFChart (strict)"("XScale.Multiplier"=w237) -> ()  [unwired: 2 in, 2 out]
    }
  }
  n123 = property on="Software version" class="Str"("Visible"=TRUE) -> ()  [unwired: 2 in, 2 out]
  n124 = disable-structure shown="Disabled" {
    frame Disabled {
      n125 = call-poly <vilib>:"DAQmx Configure Logging.vi"() -> ()  [unwired: 14 in, 2 out]
    }
    frame Enabled {
    }
  }
  n126 = disable-structure shown="Disabled" {
    frame Disabled {
      n127 = local read "Unity connected"() -> (w257:bool)
      n128 = case shown="False" w257 {
        frame False {
          n129 = case shown="True" {
            selector: _ -> [_ _]
            frame False {
            }
            frame True {
              n130 = call <vilib>:"System Exec.vi"("wait until completion? (T)"=FALSE, "working directory"="working directory", "command line"="command line") -> ()  [unwired: 5 in, 4 out]
              n131 = Wait (ms)(milliseconds to wait=u32 1000) -> ()  [unwired: 1 out]
            }
          }
        }
        frame True {
        }
      }
    }
    frame Enabled {
    }
  }
  n132 = local write "Eable security cam"(w29) -> ()
  n133 = local write "Eable eye cam"(w29) -> ()
  n134 = property on="Cam ON /OFF" class="Bool (strict)"("DisabledEnum"=T8."Disabled and Grayed Out" ("Disabled")) -> ()  [unwired: 2 in, 2 out]
  n135 = property on="Record Button 2" class="Bool (strict)"("DisabledEnum"=T8."Disabled and Grayed Out" ("Disabled")) -> ()  [unwired: 2 in, 2 out]
  n136 = local write "msg tag"("str," ("msg tag")) -> ()
  n137 = local write "Stop recording"(FALSE ("Stop recording")) -> ()
  n138 = local write "Security camera"("Security camera: NO" ("Security camera")) -> ()
  n139 = Multiply(x=50.0, y=3.141592653589793) -> (x*y=→"Wheel circumference":dbl)
  n140 = Divide(x=1000, y=w31) -> (x/y=w33:dbl)
  n141 = property on="Header" class="Str"("Visible"=TRUE) -> ()  [unwired: 2 in, 2 out]
  n142 = disable-structure shown="Disabled" {
    frame Disabled {
      n143 = Add Array Elements() -> (numeric array=w264:dbl[], sum=w263:dbl)
      n144 = Array Size(array=w264) -> (size(s)=w262:i32)
      n145 = Divide(x=w263, y=w262) -> ()  [unwired: 1 out]
    }
    frame Enabled {
    }
  }
  n146 = local write "Target frame rate"(w31) -> ()
  n147 = local write "Write loop stopped"(TRUE ("Read loop stopped")) -> ()
  n148 = local write "Read loop stopped"(TRUE ("Read loop stopped")) -> ()
  n149 = property on="Read loop stopped" class="Bool (strict)"("Visible"=FALSE) -> ()  [unwired: 2 in, 2 out]
  n150 = property on="Write loop stopped" class="Bool (strict)"("Visible"=FALSE) -> ()  [unwired: 2 in, 2 out]
  n151 = local write "Encoder count"(0.0 ("Encoder count")) -> ()
  n152 = Multiply(x=0.9, y=w33) -> (x*y=w35:dbl)
  n153 = local write "Recording folder"("Recording folder") -> ()
  n154 = To Quad Integer(1:w35) -> (0:w36:i64)
  n155 = Get Date/Time String(date format (0)=enum16{"short", "long", "abbreviated"}."short") -> ()  [unwired: 2 in, 2 out]
  n156 = property on="Lab book file" class="Path"("Visible"=TRUE) -> ()  [unwired: 2 in, 2 out]
  n157 = local write "Record Button 2"(w30) -> ()
  n158 = local write "Pupille image saved"(w30) -> ()
  n159 = property on="index" class="DigNum (strict)"("Visible"=TRUE) -> ()  [unwired: 2 in, 2 out]
  n160 = property on="Exposure Time (ms)" class="Slide (strict)"("Maximum"=w36, "Scale.Maximum"=w36, "Value"=w36) -> ()  [unwired: 2 in, 2 out]
  n161 = property on="lick signal" class="Arr (strict)"("Visible"=TRUE) -> ()  [unwired: 2 in, 2 out]
  n162 = property on="delta distance cm" class="DigNum (strict)"("Visible"=TRUE) -> ()  [unwired: 2 in, 2 out]
  n163 = while {
    shift-right: [w265] -> _
    shift-left: w75 -> [w267]
    stop <- w268 stop-if-true
    n164 = case shown="\"Record VR\"" w267 {
      tunnel: [T13."Idle" ("main program") w625 w1008 T13."Idle" ("main program") T13."Idle" ("main program") w1123 w1231] -> w265
      frame "Init program", Default {
        w320 = 11 ("index")
        w338 = 9 ("index")
        w339 = 0 ("index")
        w343 = 13 ("length")
        w293 = string[] ["Encoder signal", "Photo-diode", "Distance (cm)", "Position in Unity", "Valve open", "Lick signal", "Analog lick signal", "VR context", "VR gain", "Frame signal", "Frame signal 2", "EyeCam frame signal", "Analog input 3", "Photo stimulus signal", "Masking light signal", "Stimulus protocol", "Analog input 5"] ("channel name(s) in (Untitled)")
        w350 = 1 ("y")
        (unwired) path "C:/Users/Mate Neubrandt/Desktop/test/Task config" ("path")
        w285 = "Last calibration.txt" ("name or relative path")
        w276 = "List of mice.txt" ("name or relative path")
        w388 = u16 0 items=["none"] ("Stim. prot 1")
        w389 = u16 0 ("stim. num. 2")
        # "9"
        # "13"
        # "16"
        n165 = local read "settings folder"() -> (w277:path)
        n166 = local read "settings folder"() -> (w287:path)
        n167 = local write "Stim array length"(u16 10 ("Denominator")) -> ()
        n168 = local write "stim. num. 2"(w389) -> ()
        n169 = local write "stim. num. 3"(w389) -> ()
        n170 = local write "stim. num. 4"(w389) -> ()
        n171 = local write "stim. num. 5"(w389) -> ()
        n172 = local write "Record 2P"(FALSE ("SciScan")) -> ()
        n173 = local write "Block num. 2"(w389) -> ()
        n174 = local write "Block num. 3"(w389) -> ()
        n175 = local write "Block num. 4"(w389) -> ()
        n176 = local write "Block num. 5"(w389) -> ()
        n177 = local write "Unique ID"(i8 0 ("Unique ID")) -> ()
        n178 = local write "Stim. prot 2"(w388) -> ()
        n179 = local write "Stim. prot 3"(w388) -> ()
        n180 = local write "Stim. prot 4"(w388) -> ()
        n181 = local write "Stim. prot 5"(w388) -> ()
        n182 = local write "Run experiment"(FALSE ("Record")) -> ()
        n183 = local write "Edit mouse list"(FALSE ("Edit mouse list")) -> ()
        n184 = local write "Block 2"(w388) -> ()
        n185 = local write "Block 3"(w388) -> ()
        n186 = local write "Block 4"(w388) -> ()
        n187 = local write "Block 5"(w388) -> ()
        n188 = Build Path(base path=w287, name or relative path=w285) -> (appended path=w286:path)
        n189 = Strip Path(path=w277) -> (stripped path=w282:path)  [unwired: 1 out]
        n190 = Build Path(base path=w277, name or relative path=w276) -> (appended path=w281:path)
        n191 = Strip Path(path=w287) -> (stripped path=w290:path)  [unwired: 1 out]
        n192 = call-poly <vilib>:"DAQmx Create Virtual Channel.vi"("lines"=tag "Dev1/port0/line0") -> ("task out"=→"SciScan start":refnum<k21>)  [unwired: 13 in, 1 out]
        n193 = Build Path(base path=w290, name or relative path=w285) -> (appended path=w284:path)
        n194 = call <vilib>:"Check if File or Folder Exists.vi"("path"=w286) -> ("file or folder exists?"=w289:bool, "dup path"=w288:path)  [unwired: 8 in, 1 out]
        n195 = Build Path(base path=w282, name or relative path=w276) -> (appended path=w275:path)
        n196 = call <vilib>:"Check if File or Folder Exists.vi"("path"=w281) -> ("file or folder exists?"=w278:bool, "dup path"=w279:path)  [unwired: 8 in, 1 out]
        n197 = Select(t=w279, s=w278, f=w275) -> (s? t:f=w280:path)
        n198 = Select(t=w288, s=w289, f=w284) -> (s? t:f=w283:path)
        n199 = property on="Stop recording" class="Bool (strict)"("DisabledEnum"=T8."Disabled" ("Disabled")) -> ()  [unwired: 2 in, 2 out]
        n200 = call-poly <vilib>:"Read Delimited Spreadsheet.vi"("file path (dialog if empty)"=w280) -> ("all rows"=w291:string[][])  [unwired: 9 in, 5 out]
        n201 = Open/Create/Replace File(file path (use dialog)=w283, operation (0:open)=T9."open", access (0:read/write)=enum16{"read/write", "read-only", "write-only"}."read-only") -> (refnum out=w399:refnum<file>)  [unwired: 3 in, 2 out]
        n202 = local write "Current mice"(w291) -> ()
        n203 = for {
          tunnel: w291 -> [w414] mode=indexing
          tunnel: [w410] -> w292 mode=indexing
          n204 = Index Array(array=w414, index=0) -> (element=w413:string)
          n205 = Index Array(array=w414, index=1 ("length")) -> (element=w411:string)
          n206 = Concatenate Strings(w413, "-" ("string"), w411) -> (w410:string)
        }
        n207 = Read from Text File(file (use dialog)=w399) -> (refnum out=w400:refnum<file>, text=w401:string)  [unwired: 3 in, 2 out]
        n208 = flat-sequence {
          frame #0 {
            n209 = property on="Stim protocols" class="Ring (strict)"("Strings []"=string[] []) -> ()  [unwired: 2 in, 2 out]
          }
          frame #1 {
            n210 = local read "settings folder"() -> (w492:path)
            n211 = Build Path(base path=w492, name or relative path="Stimprotocols.txt") -> (appended path=w490:path)
            n212 = call-poly <vilib>:"Read Delimited Spreadsheet.vi"("file path (dialog if empty)"=w490) -> ("all rows"=w495:string[][])  [unwired: 9 in, 5 out]
            "protocol array" <- w495
            n213 = Array Size(array=w495) -> (size(s)=w498:i32[])
            n214 = Index Array(array=w498, index=0) -> (element=w496:i32)
            n215 = for {
              N: w496 -> [_]
              tunnel: w495 -> [w509] mode=indexing
              shift-right: [w507] -> w493
              shift-left: string[] [] -> [w506]
              i -> [w508]
              n216 = Concatenate Strings(w509) -> (w503:string)
              n217 = Match Pattern(string=w503, regular expression="none") -> (before substring=w501:string, match substring=w500:string)  [unwired: 1 in, 2 out]
              n218 = Not Equal?(x=w500, y="none") -> (x != y?=w502:bool)
              n219 = Select(t=w501, s=w502, f=w500) -> (s? t:f=w499:string)
              n220 = Insert Into Array(array=w506, index=w508, new element=w499) -> (w507:string[])
            }
            n221 = property on="Stim protocols" class="Ring (strict)"("Strings []"=w493) -> ()  [unwired: 2 in, 2 out]
          }
        }
        n222 = local write "Last calibration"(w401) -> ()
        n223 = Close File(refnum=w400) -> ()  [unwired: 1 in, 2 out]
        n224 = Match Pattern(string=w401, regular expression=" ul") -> (before substring=w403:string)  [unwired: 1 in, 3 out]
        n225 = Match Pattern(string=w401, regular expression="ul / ") -> (after substring=w402:string)  [unwired: 1 in, 3 out]
        n226 = local read "Signals to delete"() -> (w315:i32[])
        n227 = property on="Ring" class="Ring (strict)"("Strings []"=w293) -> ()  [unwired: 2 in, 2 out]
        n228 = property on="Ring 2" class="Ring (strict)"("Strings []"=w293) -> ()  [unwired: 2 in, 2 out]
        n229 = property on="Ring 3" class="Ring (strict)"("Strings []"=w293) -> ()  [unwired: 2 in, 2 out]
        n230 = property on="Ring 4" class="Ring (strict)"("Strings []"=w293) -> ()  [unwired: 2 in, 2 out]
        n231 = Fract/Exp String To Number(string=w403) -> (number=w404:dbl)  [unwired: 3 in, 1 out]
        "Last saved reward size" <- w404
        n232 = Match Pattern(string=w402, regular expression=" ms ") -> (before substring=w405:string)  [unwired: 1 in, 3 out]
        n233 = property on="Mouse name" class="Ring (strict)"("Strings []"=w292) -> ()  [unwired: 2 in, 2 out]
        n234 = local write "Reward size (ul)"(w404) -> ()
        n235 = Decimal String To Number(string=w405) -> (number=w406:i32)  [unwired: 2 in, 1 out]
        n236 = local write "Valve open dur. (ms)"(w406) -> ()
        n237 = for {
          tunnel: w315 -> [w488] mode=indexing
          shift-right: [w485] -> w344
          shift-left: w293 -> [w487]
          n238 = Delete From Array(array=w487, length=1, index=w488) -> (array with subset deleted=w485:string[])  [unwired: 1 out]
        }
        "channel names" <- w344
        n239 = Delete From Array(array=w293, length=4, index=13) -> (array with subset deleted=w340:string[])  [unwired: 1 out]
        n240 = Index Array(array=w293, index=w320) -> (element=w319:string)
        n241 = Search 1D Array(1D array=w315, element=9 ("index")) -> (index of element=w329:i32)  [unwired: 1 in]
        n242 = Search 1D Array(1D array=w315, element=10 ("index")) -> (index of element=w327:i32)  [unwired: 1 in]
        n243 = Delete From Array(array=w293, length=w343, index=w339) -> (array with subset deleted=w301:string[])  [unwired: 1 out]
        n244 = Delete From Array(array=w340, length=9, index=0) -> (array with subset deleted=w321:string[])  [unwired: 1 out]
        n245 = local read "settings folder"() -> (w300:path)
        n246 = local read "settings folder"() -> (w355:path)
        n247 = Build Array(w301) -> (w303:string[][])
        n248 = Build Array(w319) -> (w305:string[])
        n249 = Greater Or Equal?(x=w329, y=0) -> (x >= y?=w326:bool)
        n250 = Greater Or Equal?(x=w327, y=0) -> (x >= y?=w325:bool)
        n251 = Delete From Array(array=w321, length=1, index=2) -> (array with subset deleted=w308:string[])  [unwired: 1 out]
        n252 = Search 1D Array(1D array=w315, element=11 ("index")) -> (index of element=w318:i32)  [unwired: 1 in]
        n253 = Transpose 2D Array(2D array=w303) -> (transposed array=→"Saved optogen. signals":string[][])
        n254 = And(x=w326, y=w325) -> (x .and. y?=w324:bool)
        n255 = Build Array(w305) -> (w306:string[][])
        n256 = Build Array(w308) -> (w309:string[][])
        n257 = Greater Or Equal?(x=w318, y=0) -> (x >= y?=w314:bool)
        n258 = Build Path(base path=w300, name or relative path="Laser stimulus calibration.txt") -> (appended path=w299:path)
        n259 = Transpose 2D Array(2D array=w306) -> (transposed array=→"Saved pupil imaging signals":string[][])
        n260 = Transpose 2D Array(2D array=w309) -> (transposed array=→"Saved 2P signals":string[][])
        n261 = Build Path(base path=w355, name or relative path="Task configuration.txt") -> (appended path=w273:path)
        n262 = Open/Create/Replace File(file path (use dialog)=w273, operation (0:open)=T9."open", access (0:read/write)=enum16{"read/write", "read-only", "write-only"}."read-only") -> (refnum out=w274:refnum<file>)  [unwired: 3 in, 2 out]
        n263 = call <vilib>:"Check if File or Folder Exists.vi"("path"=w299) -> ("file or folder exists?"=w294:bool)  [unwired: 8 in, 2 out]
        n264 = Delete From Array(array=w293, length=8, index=w338) -> (array with subset deleted=w310:string[])  [unwired: 1 out]
        n265 = Search 1D Array(1D array=w315, element=13 ("index")) -> (index of element=w346:i32)  [unwired: 1 in]
        n266 = Read from Text File(file (use dialog)=w274) -> (refnum out=w270:refnum<file>, text=→"Task config":string)  [unwired: 3 in, 2 out]
        n267 = call-poly <vilib>:"Read Delimited Spreadsheet.vi"("file path (dialog if empty)"=w273) -> ("all rows"=w386:string[][])  [unwired: 9 in, 5 out]
        n268 = Greater Or Equal?(x=w346, y=0) -> (x >= y?=w296:bool)
        n269 = for {
          shift-right: [w457] -> _
          shift-left: w308 -> [w450]
          tunnel: w315 -> [w449] mode=indexing
          n270 = Equal?(x=w449, y=9) -> (x = y?=w455:bool)
          n271 = Equal?(x=w449, y=10) -> (x = y?=w454:bool)
          n272 = Equal?(x=w449, y=12) -> (x = y?=w447:bool)
          n273 = Subtract(x=w449, y=9) -> (x-y=w444:i32)
          n274 = Compound Arithmetic op=OR(w455, w454, w447) -> (w456:bool)
          n275 = Decrement(x=w444) -> (x-1=w445:i32)
          n276 = Select(t=w445, s=w447, f=w444) -> (s? t:f=w446:i32)
          n277 = case shown="True" w456 {
            tunnel: w450 -> [w458 w464]
            tunnel: [w458 w463] -> w457
            tunnel: w446 -> [_ w461]
            frame False {
            }
            frame True {
              n278 = Delete From Array(array=w464, length=1, index=w461) -> (array with subset deleted=w463:string[])  [unwired: 1 out]
              n279 = Bundle(w461, 0) -> (w462:cluster{i32, i32})  [unwired: 1 in]
              n280 = property on="Saved 2P signals" class="Tbl (strict)"("Active Cell"=w462, "Cell BG Color"=u32 13816530) -> ()  [unwired: 2 in, 2 out]
            }
          }
        }
        n281 = for {
          tunnel: w315 -> [w421] mode=indexing
          tunnel: w320 -> [w420]
          shift-right: [w417] -> _
          shift-left: w305 -> [w418]
          n282 = Equal?(x=w421, y=w420) -> (x = y?=w419:bool)
          n283 = case shown="True" w419 {
            tunnel: w418 -> [w422 _]
            tunnel: [w422 string[] []] -> w417
            frame False {
            }
            frame True {
              w425 = 0
              n284 = Bundle(w425, w425) -> (w424:cluster{i32, i32})  [unwired: 1 in]
              n285 = property on="Saved pupil imaging signals" class="Tbl (strict)"("Active Cell"=w424, "Cell BG Color"=u32 13816530) -> ()  [unwired: 2 in, 2 out]
            }
          }
        }
        n286 = for {
          tunnel: w343 -> [w472]
          tunnel: w315 -> [w471] mode=indexing
          shift-right: [w468] -> _
          shift-left: w301 -> [w469]
          tunnel: w339 -> [w466]
          n287 = Subtract(x=w471, y=w472) -> (x-y=w467:i32)
          n288 = Greater Or Equal?(x=w467, y=w466) -> (x >= y?=w470:bool)
          n289 = case shown="True" w470 {
            tunnel: w469 -> [w473 w479]
            tunnel: [w473 w478] -> w468
            tunnel: w467 -> [_ w474]
            frame False {
            }
            frame True {
              n290 = Delete From Array(array=w479, length=1, index=w474) -> (array with subset deleted=w478:string[])  [unwired: 1 out]
              n291 = Bundle(w474, 0) -> (w476:cluster{i32, i32})  [unwired: 1 in]
              n292 = property on="Saved optogen. signals" class="Tbl (strict)"("Active Cell"=w476, "Cell BG Color"=u32 13816530) -> ()  [unwired: 2 in, 2 out]
            }
          }
        }
        n293 = Close File(refnum=w270) -> ()  [unwired: 1 in, 2 out]
        n294 = Not(x=w296) -> (.not. x?=w295:bool)
        n295 = for {
          tunnel: w315 -> [w432] mode=indexing
          shift-right: [w433] -> _
          shift-left: w310 -> [w434]
          tunnel: w338 -> [w431]
          n296 = Less?(x=w432, y=w431) -> (x < y?=w435:bool)
          n297 = case shown="True" w435 {
            tunnel: w434 -> [w436 w442]
            tunnel: [w436 w441] -> w433
            tunnel: w432 -> [_ w440]
            frame False {
            }
            frame True {
              n298 = Delete From Array(array=w442, length=1, index=w440) -> (array with subset deleted=w441:string[])  [unwired: 1 out]
              n299 = Bundle("String"=w440, 0) -> (w438:cluster{"String":i32, i32})  [unwired: 1 in]
              n300 = property on="Behavior and VR signals saved" class="Tbl (strict)"("Active Cell"=w438, "Cell BG Color"=u32 13816530) -> ()  [unwired: 2 in, 2 out]
            }
          }
        }
        n301 = Build Array(w310) -> (w312:string[][])
        n302 = Delete From Array(array=w386, length=1, index (col)=0 ("disabled index (col)")) -> (deleted portion=w383:string[][], array with subset deleted=w372:string[][])  [unwired: 1 in]
        n303 = And(x=w295, y=w294) -> (x .and. y?=w297:bool)
        n304 = Transpose 2D Array(2D array=w312) -> (transposed array=→"Behavior and VR signals saved":string[][])
        n305 = case shown="False" w297 {
          frame False {
            n306 = local write "Enable stim."(FALSE ("Enable stim.")) -> ()
            n307 = property on="Enable stim." class="Bool (strict)"("DisabledEnum"=T8."Disabled and Grayed Out" ("Disabled")) -> ()  [unwired: 2 in, 2 out]
          }
          frame True {
            n308 = local write "Enable stim."(TRUE ("Enable stim.")) -> ()
            n309 = property on="Enable stim." class="Bool (strict)"("DisabledEnum"=T8."Enabled" ("Disabled")) -> ()  [unwired: 2 in, 2 out]
          }
        }
        n310 = Array Size(array=w383) -> (size(s)=w382:i32[])
        n311 = Index Array(array=w382, index=0) -> (element=w380:i32)
        n312 = Reshape Array(w383, w380) -> (w354:string[])
        n313 = Decimal String To Number(string=w372) -> (number=w369:i32[][])  [unwired: 2 in, 1 out]
        n314 = property on="Block 1" class="Ring (strict)"("Strings []"=w354) -> ()  [unwired: 2 in, 2 out]
        n315 = property on="Block 2" class="Ring (strict)"("Strings []"=w354) -> ()  [unwired: 2 in, 2 out]
        n316 = property on="Block 3" class="Ring (strict)"("Strings []"=w354) -> ()  [unwired: 2 in, 2 out]
        n317 = property on="Block 4" class="Ring (strict)"("Strings []"=w354) -> ()  [unwired: 2 in, 2 out]
        n318 = property on="Block 5" class="Ring (strict)"("Strings []"=w354) -> ()  [unwired: 2 in, 2 out]
        n319 = Delete From Array(array=w369, length=1, index (col)=0 ("disabled index (col)")) -> (deleted portion=w364:i32[][], array with subset deleted=w368:i32[][])  [unwired: 1 in]
        n320 = property on="plot selector 1" class="Ring (strict)"("Strings []"=w354) -> ()  [unwired: 2 in, 2 out]
        n321 = property on="plot selector 2" class="Ring (strict)"("Strings []"=w354) -> ()  [unwired: 2 in, 2 out]
        n322 = Delete From Array(array=w368, length=1, index (col)=0 ("disabled index (col)")) -> (deleted portion=w358:i32[][], array with subset deleted=→"zeward zones":i32[][])  [unwired: 1 in]
        n323 = local read "Eable eye cam"() -> (w334:bool)
        n324 = Not(x=w314) -> (.not. x?=w313:bool)
        n325 = local read "command line"() -> (w379:string)
        n326 = And(x=w313, y=w334) -> (x .and. y?=w333:bool)
        n327 = case shown="True" w324 {
          frame False {
            n328 = property on="Record 2P" class="Bool (strict)"("DisabledEnum"=T8."Enabled" ("Disabled")) -> ()  [unwired: 2 in, 2 out]
          }
          frame True {
            n329 = property on="Record 2P" class="Bool (strict)"("DisabledEnum"=T8."Disabled and Grayed Out" ("Disabled")) -> ()  [unwired: 2 in, 2 out]
          }
        }
        n330 = Array Size(array=w364) -> (size(s)=w365:i32[])
        n331 = Array Size(array=w358) -> (size(s)=w360:i32[])
        n332 = Array Size(array=w354) -> (size(s)=w353:i32)
        n333 = case shown="False" w333 {
          selector: w333 -> [_ w429]
          frame True {
          }
          frame False {
            n334 = local write "Eable eye cam"(w429) -> ()
            n335 = property on="Record Button 2" class="Bool (strict)"("DisabledEnum"=T8."Disabled and Grayed Out" ("Disabled")) -> ()  [unwired: 2 in, 2 out]
          }
        }
        n336 = Index Array(array=w365, index=0) -> (element=w363:i32)
        n337 = Index Array(array=w360, index=0) -> (element=w361:i32)
        n338 = Greater?(x=w353, y=w350) -> (0:w351:bool)
        n339 = Reshape Array(w364, w363) -> (→"corridor lengths":i32[])
        n340 = Reshape Array(w358, w361) -> (→"teleports":i32[])
        n341 = Match Pattern(string=w379, regular expression=".exe") -> (before substring=w377:string)  [unwired: 1 in, 3 out]
        n342 = Select(t=w350, s=w351, f=2) -> (s? t:f=w352:i32)
        n343 = property on="plot selector 2" class="Ring (strict)"("Value"=w352) -> ()  [unwired: 2 in, 2 out]
        n344 = Concatenate Strings(w377, "_config" ("string")) -> (w375:string)
        n345 = Build Path(name or relative path=w375) -> ()  [unwired: 1 in, 1 out]
      }
      frame "Idle" {
        w554 = string[] []
        w577 = u16[] []
        w578 = u16[] []
        w614 = 1 ("length")
        # "Save reward calibration data"
        # "Select mouse from the current list of mice"
        n346 = local read "stim. num. 1"() -> (w511:u16)
        n347 = local read "stim. num. 2"() -> (w582:u16)
        n348 = local read "stim. num. 3"() -> (w581:u16)
        n349 = local read "stim. num. 4"() -> (w580:u16)
        n350 = local read "stim. num. 5"() -> (w579:u16)
        n351 = stacked-sequence {
          seq-local: ["Stim protocols" _] -> [_ w751]
          seq-local: [w698 _] -> [_ w773]
          tunnel: [_ w749] -> w592
          frame #0 {
            n352 = call "Is Value Changed.vim"("value"="Stim protocols") -> ("changed or first call?"=w700:bool)
            n353 = local read "protocol array"() -> (w698:string[][])
            n354 = case shown="True" w700 {
              tunnel: w698 -> [_ w706]
              tunnel: "Stim protocols" -> [_ w704]
              frame False {
              }
              frame True {
                n355 = Index Array(array=w706, index (row)=w704, index (col)=2 ("disabled index (col)")) -> (element=w712:string)
                n356 = Index Array(array=w706, index (row)=w704, index (col)=0 ("disabled index (col)")) -> (element=w717:string)
                n357 = property on="Stim type" class="Ring (strict)"() -> ("StringsAndValues[]"=w715:T16)  [unwired: 2 in, 2 out]
                n358 = Index Array(array=w706, index (row)=w704, index (col)=1 ("disabled index (col)")) -> (element=w714:string)
                n359 = Index Array(array=w706, index (row)=w704, index (col)=4 ("disabled index (col)")) -> (element=w705:string)
                n360 = Index Array(array=w706, index (row)=w704, index (col)=3 ("disabled index (col)")) -> (element=w721:string)
                n361 = Match Pattern(string=w712, regular expression="to ") -> (after substring=w713:string)  [unwired: 1 in, 3 out]
                n362 = Match Pattern(string=w714, regular expression="from ") -> (after substring=w726:string)  [unwired: 1 in, 3 out]
                n363 = Not Equal?(x=w713, y="rew") -> ()  [unwired: 1 out]
                n364 = Match Pattern(string=w721, regular expression=" int. ") -> (after substring=w720:string)  [unwired: 1 in, 3 out]
                n365 = Not Equal?(x=w726, y="rew") -> ()  [unwired: 1 out]
                n366 = Match Pattern(string=w705, regular expression=" duty cycle. ") -> (after substring=w710:string)  [unwired: 1 in, 3 out]
                n367 = Match Pattern(string=w720, regular expression=" %  ") -> (before substring=w719:string)  [unwired: 1 in, 3 out]
                n368 = Match Pattern(string=w710, regular expression=" %  ") -> (before substring=w711:string)  [unwired: 1 in, 3 out]
                n369 = Decimal String To Number(string=w726) -> (number=w702:i32)  [unwired: 2 in, 1 out]
                n370 = Decimal String To Number(string=w713) -> (number=w701:i32)  [unwired: 2 in, 1 out]
                n371 = Array Size(array=w715) -> (size(s)=w718:i32)
                n372 = for {
                  N: w718 -> [_]
                  tunnel: w717 -> [w735]
                  tunnel: w715 -> [w734] mode=indexing
                  n373 = Unbundle(w734) -> ("String"=w733:string, "Value"=w737:u16)
                  n374 = Equal?(x=w735, y=w733) -> (x = y?=w736:bool)
                  n375 = case shown="True" w736 {
                    tunnel: w737 -> [_ w738]
                    frame False {
                    }
                    frame True {
                      n376 = local write "Stim type"(w738) -> ()
                    }
                  }
                }
                n377 = Decimal String To Number(string=w711) -> (number=w703:i32)  [unwired: 2 in, 1 out]
                n378 = Decimal String To Number(string=w719) -> (number=w716:i32)  [unwired: 2 in, 1 out]
                n379 = local write "Intensity (%)"(w716) -> ()
                n380 = local write "Duty cycle (%)"(w703) -> ()
                n381 = local write "start (cm)"(w702) -> ()
                n382 = local write "stop (cm)"(w701) -> ()
              }
            }
          }
          frame #1 {
            w746 = "" ("new element/subarray")
            w748 = 0 ("index (row)")
            n383 = Number To Decimal String(number="stop (cm)") -> (decimal integer string=w744:string)  [unwired: 1 in]
            n384 = Number To Decimal String(number="Duty cycle (%)") -> (decimal integer string=w757:string)  [unwired: 1 in]
            n385 = Number To Decimal String(number="Intensity (%)") -> (decimal integer string=w778:string)  [unwired: 1 in]
            n386 = Concatenate Strings(" to " ("string"), w744) -> (w787:string)
            n387 = property on="Stim type" class="Ring (strict)"() -> ("RingText.Text"=w760:string)  [unwired: 2 in, 2 out]
            n388 = Number To Decimal String(number="start (cm)") -> (decimal integer string=w740:string)  [unwired: 1 in]
            n389 = property on="stop (cm)" class="DigNum (strict)"("DisabledEnum"=T8."Enabled" ("Disabled")) -> ()  [unwired: 2 in, 2 out]
            n390 = property on="start (cm)" class="DigNum (strict)"("DisabledEnum"=T8."Enabled" ("Disabled")) -> ()  [unwired: 2 in, 2 out]
            n391 = Concatenate Strings(" from " ("string"), w740) -> (w786:string)
            n392 = Concatenate Strings(" int. " ("string"), w778, " %" ("string")) -> (w788:string)
            n393 = Concatenate Strings(" duty cycle " ("string"), w757, " %" ("string")) -> (w753:string)
            n394 = Not Equal?(x=w760, y="none") -> (x != y?=w761:bool)
            n395 = case shown="True" w761 {
              tunnel: w788 -> [w794 _]
              tunnel: w787 -> [w793 _]
              tunnel: w786 -> [w792 _]
              tunnel: [w791 w797] -> w782
              tunnel: w760 -> [w790 w796]
              tunnel: w753 -> [w789 _]
              frame True {
                n396 = Build Array(w790, w792, w793, w794, w789) -> (w791:string[])
              }
              frame False {
                w795 = "" ("element")
                n397 = Build Array(w796, w795, w795, w795, w795) -> (w797:string[])
              }
            }
            n398 = Replace Array Subset(array=w773, new element=w760, index (row)=w751, index (col)=0 ("disabled index (col)")) -> (w783:string[][])
            n399 = Replace Array Subset(array=w783, new element=w786, index (row)=w751, index (col)=1 ("disabled index (col)")) -> (w784:string[][])
            n400 = Replace Array Subset(array=w784, new element=w787, index (row)=w751, index (col)=2 ("disabled index (col)")) -> (w785:string[][])
            n401 = Replace Array Subset(array=w785, new element=w788, index (row)=w751, index (col)=3 ("disabled index (col)")) -> (w752:string[][])
            n402 = Replace Array Subset(array=w752, new element=w753, index (row)=w751, index (col)=4 ("disabled index (col)")) -> (w754:string[][])
            n403 = Replace Array Subset(array=w754, new element="none" ("new element/subarray"), index (row)=w748, index (col)=0 ("disabled index (col)")) -> (w767:string[][])
            n404 = Replace Array Subset(array=w767, new element=w746, index (row)=w748, index (col)=1 ("disabled index (col)")) -> (w766:string[][])
            n405 = Replace Array Subset(array=w766, new element=w746, index (row)=w748, index (col)=2 ("disabled index (col)")) -> (w765:string[][])
            n406 = Replace Array Subset(array=w765, new element=w746, index (row)=w748, index (col)=3 ("disabled index (col)")) -> (w750:string[][])
            n407 = Replace Array Subset(array=w750, new element=w746, index (row)=w748, index (col)=4 ("disabled index (col)")) -> (w749:string[][])
            n408 = local write "protocol array"(w749) -> ()
            n409 = Concatenate Strings(w782) -> (w781:string)
            n410 = property on="Stim protocols" class="Ring (strict)"("RingText.Text"=w781) -> ()  [unwired: 2 in, 2 out]
          }
        }
        n411 = Compound Arithmetic op=ADD(w511, w582, w581, w580, w579) -> (w510:u16)
        "Stim array length" <- w510
        n412 = Build Array("Stim. prot 1", "Stim. prot 2", "Stim. prot 3", "Stim. prot 4", "Stim. prot 5") -> (w555:u16[])
        n413 = for {
          N: "stim. num. 2" -> [_]
          tunnel: "Stim. prot 2" -> [w883]
          shift-right: [w882] -> w590
          shift-left: w578 -> [w881]
          i -> [w884]
          n414 = Insert Into Array(array=w881, index=w884, new element=w883) -> (w882:u16[])
        }
        n415 = for {
          N: "stim. num. 3" -> [_]
          tunnel: "Stim. prot 3" -> [w879]
          shift-right: [w878] -> w591
          shift-left: w578 -> [w877]
          i -> [w880]
          n416 = Insert Into Array(array=w877, index=w880, new element=w879) -> (w878:u16[])
        }
        n417 = for {
          N: "stim. num. 4" -> [_]
          tunnel: "Stim. prot 4" -> [w875]
          shift-right: [w874] -> w588
          shift-left: w578 -> [w873]
          i -> [w876]
          n418 = Insert Into Array(array=w873, index=w876, new element=w875) -> (w874:u16[])
        }
        n419 = for {
          N: "stim. num. 1" -> [_]
          tunnel: "Stim. prot 1" -> [w887]
          shift-right: [w886] -> w589
          shift-left: w578 -> [w885]
          i -> [w888]
          n420 = Insert Into Array(array=w885, index=w888, new element=w887) -> (w886:u16[])
        }
        n421 = for {
          N: "stim. num. 5" -> [_]
          tunnel: "Stim. prot 5" -> [w871]
          shift-right: [w870] -> w587
          shift-left: w578 -> [w869]
          i -> [w872]
          n422 = Insert Into Array(array=w869, index=w872, new element=w871) -> (w870:u16[])
        }
        n423 = for {
          N: w510 -> [_]
          shift-right: [w894] -> w594
          shift-left: i32[] [] -> [w893]
          i -> [w895]
          n424 = Insert Into Array(array=w893, index=w895, new element=w895) -> (w894:i32[])
        }
        n425 = Build Array (concatenate)(w589, w590, w591, w588, w587) -> (→"Stim types":u16[])
        n426 = local write "shuffled array"(w594) -> ()
        n427 = Build Array("Block 1", "Block 2", "Block 3", "Block 4", "Block 5") -> (w542:u16[])
        n428 = local read "Block num. 1"() -> (w527:u16)
        n429 = local read "Block num. 2"() -> (w528:u16)
        n430 = local read "Block num. 3"() -> (w529:u16)
        n431 = local read "Block num. 4"() -> (w530:u16)
        n432 = local read "Block num. 5"() -> (w526:u16)
        n433 = for {
          N: "Block num. 1" -> [_]
          tunnel: "Block 1" -> [w867]
          shift-right: [w866] -> w572
          shift-left: w577 -> [w865]
          i -> [w868]
          n434 = Insert Into Array(array=w865, index=w868, new element=w867) -> (w866:u16[])
        }
        n435 = for {
          N: "Block num. 2" -> [_]
          tunnel: "Block 2" -> [w863]
          shift-right: [w862] -> w571
          shift-left: w577 -> [w861]
          i -> [w864]
          n436 = Insert Into Array(array=w861, index=w864, new element=w863) -> (w862:u16[])
        }
        n437 = for {
          N: "Block num. 3" -> [_]
          tunnel: "Block 3" -> [w859]
          shift-right: [w858] -> w570
          shift-left: w577 -> [w857]
          i -> [w860]
          n438 = Insert Into Array(array=w857, index=w860, new element=w859) -> (w858:u16[])
        }
        n439 = for {
          N: "Block num. 4" -> [_]
          tunnel: "Block 4" -> [w855]
          shift-right: [w854] -> w569
          shift-left: w577 -> [w853]
          i -> [w856]
          n440 = Insert Into Array(array=w853, index=w856, new element=w855) -> (w854:u16[])
        }
        n441 = for {
          N: "Block num. 5" -> [_]
          tunnel: "Block 5" -> [w851]
          shift-right: [w850] -> w568
          shift-left: w577 -> [w849]
          i -> [w852]
          n442 = Insert Into Array(array=w849, index=w852, new element=w851) -> (w850:u16[])
        }
        n443 = call "Is Value Changed.vim"("value"=w592) -> ("changed or first call?"=w593:bool)
        n444 = property on="Stim protocols" class="Ring (strict)"() -> ("Strings []"=w567:string[])  [unwired: 2 in, 2 out]
        n445 = local read "VR Controller"() -> (w515:T1)
        n446 = property on="Stim. prot 1" class="Ring (strict)"("Strings []"=w567) -> ()  [unwired: 2 in, 2 out]
        n447 = property on="Stim. prot 2" class="Ring (strict)"("Strings []"=w567) -> ()  [unwired: 2 in, 2 out]
        n448 = property on="Stim. prot 3" class="Ring (strict)"("Strings []"=w567) -> ()  [unwired: 2 in, 2 out]
        n449 = property on="Stim. prot 4" class="Ring (strict)"("Strings []"=w567) -> ()  [unwired: 2 in, 2 out]
        n450 = property on="Stim. prot 5" class="Ring (strict)"("Strings []"=w567) -> ()  [unwired: 2 in, 2 out]
        n451 = case shown="True" w593 {
          tunnel: w592 -> [_ w892]
          frame False {
          }
          frame True {
            n452 = local read "settings folder"() -> (w891:path)
            n453 = Build Path(base path=w891, name or relative path="Stimprotocols.txt") -> (appended path=w889:path)
            n454 = call-poly <vilib>:"Write Delimited Spreadsheet.vi"("file path (dialog if empty)"=w889, "2D data"=w892) -> ()  [unwired: 12 in, 2 out]
          }
        }
        n455 = Equal?(x=w515, y=T1."Configuration") -> (x = y?=w516:bool)
        n456 = Compound Arithmetic op=ADD(w527, w528, w529, w530, w526) -> (→"Session length":u16)
        n457 = Build Array (concatenate)(w572, w571, w570, w569, w568) -> (→"Context types":u16[])
        n458 = case shown="True" w516 {
          frame False {
          }
          frame True {
            n459 = Path To String(path="Path") -> (string=w632:string)
            n460 = Path To String(path="Path 2") -> (string=w631:string)
            n461 = Boolean To (0,1)(Boolean="Save") -> (0, 1=w670:i16[])
            n462 = Boolean To (0,1)(Boolean="Save 2") -> (0, 1=w669:i16[])
            n463 = Boolean To (0,1)(Boolean="Save 3") -> (0, 1=w667:i16[])
            n464 = Replace Array Subset(array="Default var. edit", new element=w632, index (row)=4, index (col)=1 ("disabled index (col)")) -> (w639:string[][])
            n465 = Replace Array Subset(array="Default var. edit", new element=w631, index (row)=6, index (col)=1 ("disabled index (col)")) -> (w636:string[][])
            n466 = Number To Decimal String(number=w670) -> (decimal integer string=w663:string[])  [unwired: 1 in]
            n467 = Number To Decimal String(number=w669) -> (decimal integer string=w665:string[])  [unwired: 1 in]
            n468 = Number To Decimal String(number=w667) -> (decimal integer string=w664:string[])  [unwired: 1 in]
            n469 = call "Is Value Changed.vim"("value"=w632) -> ("changed or first call?"=w640:bool)
            n470 = call "Is Value Changed.vim"("value"=w631) -> ("changed or first call?"=w637:bool)
            n471 = Select(t=w639, s=w640, f="Default var. edit") -> (s? t:f=w638:string[][])
            n472 = Build Array (concatenate)(w663, w665, w664) -> (w662:string[])
            n473 = Select(t=w636, s=w637, f="Default var. edit") -> (s? t:f=w635:string[][])
            n474 = local read "Exit program"() -> (w647:bool)
            n475 = local write "Default var. edit"(w635) -> ()
            n476 = local write "Default var. edit"(w638) -> ()
            n477 = local read "Default var. edit"() -> (w654:string[][])
            n478 = local read "settings folder"() -> (w649:path)
            n479 = Or(x="Save and exit", y=w647) -> (x .or. y?=w645:bool)
            n480 = Build Path(base path=w649, name or relative path="Default variables.txt") -> (appended path=w648:path)
            n481 = Build Path(base path=w649, name or relative path="Task configuration.txt") -> (appended path=w655:path)
            n482 = Build Path(base path=w649, name or relative path="Data saving config.txt") -> (appended path=w652:path)
            n483 = Build Path(base path=path "C:/VR Controller/data" ("t"), name or relative path="Select user profile") -> (appended path=w658:path)
            n484 = call "Is Value Changed.vim"("value"=w658) -> ("changed or first call?"=w660:bool)
            n485 = case shown="True" w660 {
              tunnel: w658 -> [_ w694]
              tunnel: [w681 w693] -> w659
              tunnel: w658 -> [_ w689]
              tunnel: w658 -> [_ w686]
              frame False {
                n486 = local read "Behavior and task related signals"() -> (w684:string[])
                n487 = local read "Imaging ralated signals"() -> (w683:string[])
                n488 = local read "Optogenetics related signals"() -> (w682:string[])
                n489 = Build Array (concatenate)(w684, w683, w682) -> (w681:string[])
              }
              frame True {
                n490 = call "Read signal settings.vi"("base path"=w694) -> ("channel name(s) in (Untitled)"=w692:string[], "Save"=w697:bool[], "channel name(s) in (Untitled) 2"=w691:string[], "Save 2"=w696:bool[], "channel name(s) in (Untitled) 3"=w690:string[], "Save 3"=w695:bool[])  [unwired: 13 in]
                "Imaging ralated signals" <- w691
                "Behavior and task related signals" <- w692
                "Optogenetics related signals" <- w690
                n491 = call "Read def. var..vi"("settings folder"=w689) -> ("Name column"=→"Default variables":string[], "Default var."=w687:string[][])  [unwired: 9 in]
                n492 = call "Read task config..vi"("settings folder"=w686) -> ("table"=w685:string[][])  [unwired: 10 in]
                n493 = local write "Task configuration"(w685) -> ()
                n494 = local write "Default var. edit"(w687) -> ()
                n495 = local write "Save"(w697) -> ()
                n496 = local write "Save 3"(w695) -> ()
                n497 = local write "Save 2"(w696) -> ()
                n498 = Build Array (concatenate)(w692, w691, w690) -> (w693:string[])
              }
            }
            n499 = Build Array(w659, w662) -> (w661:string[][])
            n500 = Transpose 2D Array(2D array=w661) -> (transposed array=w651:string[][])
            n501 = case shown="True" w645 {
              selector: w645 -> [_ w674]
              tunnel: "Task configuration" -> [_ w680]
              tunnel: w655 -> [_ w679]
              tunnel: w654 -> [_ w678]
              tunnel: w652 -> [_ w677]
              tunnel: w651 -> [_ w676]
              tunnel: w648 -> [_ w675]
              frame False {
              }
              frame True {
                n502 = local write "Exit program"(w674) -> ()
                n503 = call-poly <vilib>:"Write Delimited Spreadsheet.vi"("file path (dialog if empty)"=w675, "2D data"=w678) -> ()  [unwired: 12 in, 2 out]
                n504 = call-poly <vilib>:"Write Delimited Spreadsheet.vi"("file path (dialog if empty)"=w677, "2D data"=w676) -> ()  [unwired: 12 in, 2 out]
                n505 = call-poly <vilib>:"Write Delimited Spreadsheet.vi"("file path (dialog if empty)"=w679, "2D data"=w680) -> ()  [unwired: 12 in, 2 out]
              }
            }
            n506 = local write "settings folder"(w658) -> ()
          }
        }
        n507 = local read "stim. num. 1"() -> (w564:u16)
        n508 = local read "stim. num. 2"() -> (w563:u16)
        n509 = local read "stim. num. 3"() -> (w562:u16)
        n510 = local read "stim. num. 4"() -> (w561:u16)
        n511 = local read "stim. num. 5"() -> (w560:u16)
        n512 = local read "Block num. 1"() -> (w552:u16)
        n513 = local read "Block num. 2"() -> (w551:u16)
        n514 = local read "Block num. 3"() -> (w550:u16)
        n515 = local read "Block num. 4"() -> (w549:u16)
        n516 = local read "Block num. 5"() -> (w548:u16)
        n517 = local read "Last saved reward size"() -> (w603:dbl)
        n518 = Build Array(w564, w563, w562, w561, w560) -> (w553:u16[])
        n519 = Build Array(w552, w551, w550, w549, w548) -> (w547:u16[])
        n520 = Array Size(array=w553) -> (size(s)=w566:i32)
        n521 = for {
          N: w566 -> [_]
          tunnel: w542 -> [w812] mode=indexing
          shift-right: [w808] -> w539
          shift-left: w554 -> [w807]
          tunnel: w547 -> [w806] mode=indexing
          tunnel: w555 -> [w800] mode=indexing
          shift-right: [w804] -> w541
          shift-left: w554 -> [w799]
          tunnel: w553 -> [w805] mode=indexing
          i -> [w798]
          n522 = Greater?(x=w806, y=u16 0) -> (0:w811:bool)
          n523 = Greater?(x=w805, y=u16 0) -> (0:w801:bool)
          n524 = case shown="True" w811 {
            tunnel: w812 -> [_ w848]
            tunnel: w806 -> [_ w847]
            tunnel: ["" w836] -> w809
            frame False {
            }
            frame True {
              n525 = property on="Block 1" class="Ring (strict)"() -> ("StringsAndValues[]"=w831:T16)  [unwired: 2 in, 2 out]
              n526 = local read "Session length"() -> (w832:u16)
              n527 = Number To Decimal String(number=w847) -> (decimal integer string=w842:string)  [unwired: 1 in]
              n528 = Index Array(array=w831, index=w848) -> (element=w846:cluster{"String":string, "Value":u16})
              n529 = Number To Decimal String(number=w832) -> (decimal integer string=w840:string)  [unwired: 1 in]
              n530 = Concatenate Strings(w842, "/" ("string"), w840) -> (w839:string)
              n531 = Unbundle(w846) -> ("String"=w835:string, "Value"=w845:u16)
              n532 = Number To Decimal String(number=w845) -> (decimal integer string=w844:string)  [unwired: 1 in]
              n533 = Match Pattern(string=w835, regular expression="int. ") -> (before substring=w833:string)  [unwired: 1 in, 3 out]
              n534 = Concatenate Strings(w844, ": " ("string"), w839, " " ("string"), w833, "\n" ("string")) -> (w836:string)
            }
          }
          n535 = case shown="True" w801 {
            tunnel: w800 -> [_ w828]
            tunnel: w805 -> [_ w827]
            tunnel: ["" w814] -> w803
            frame False {
            }
            frame True {
              n536 = property on="Stim protocols" class="Ring (strict)"() -> ("StringsAndValues[]"=w829:T16)  [unwired: 2 in, 2 out]
              n537 = local read "Stim array length"() -> (w820:u16)
              n538 = Number To Decimal String(number=w827) -> (decimal integer string=w822:string)  [unwired: 1 in]
              n539 = Index Array(array=w829, index=w828) -> (element=w826:cluster{"String":string, "Value":u16})
              n540 = Number To Decimal String(number=w820) -> (decimal integer string=w819:string)  [unwired: 1 in]
              n541 = Unbundle(w826) -> ("String"=w816:string, "Value"=w825:u16)
              n542 = Concatenate Strings(w822, "/" ("string"), w819) -> (w818:string)
              n543 = Number To Decimal String(number=w825) -> (decimal integer string=w824:string)  [unwired: 1 in]
              n544 = Concatenate Strings(w824, ": " ("string"), w818, " " ("string"), w816, "\n" ("string")) -> (w814:string)
            }
          }
          n545 = Insert Into Array(array=w807, index=w798, new element=w809) -> (w808:string[])
          n546 = Insert Into Array(array=w799, index=w798, new element=w803) -> (w804:string[])
        }
        n547 = Not Equal?(x="Reward size (ul)", y=w603) -> (x != y?=w617:bool)
        n548 = case shown="True" w617 {
          tunnel: "Reward size (ul)" -> [_ w908]
          frame False {
          }
          frame True {
            w905 = "Last calibration.txt" ("name or relative path")
            n549 = local write "Last saved reward size"(w908) -> ()
            n550 = local read "settings folder"() -> (w907:path)
            n551 = local read "Valve open dur. (ms)"() -> (w916:u32)
            n552 = local read "Date"() -> (w911:string)
            n553 = Strip Path(path=w907) -> (stripped path=w906:path)  [unwired: 1 out]
            n554 = Build Path(base path=w907, name or relative path=w905) -> (appended path=w903:path)
            n555 = Number To Decimal String(number=w916) -> (decimal integer string=w917:string)  [unwired: 1 in]
            n556 = call <vilib>:"Check if File or Folder Exists.vi"("path"=w903) -> ("file or folder exists?"=w901:bool, "dup path"=w902:path)  [unwired: 8 in, 1 out]
            n557 = Build Path(base path=w906, name or relative path=w905) -> (appended path=w900:path)
            n558 = Number To Fractional String(number=w908, precision (6)=i16 2) -> (F-format string=w919:string)  [unwired: 2 in]
            n559 = Select(t=w902, s=w901, f=w900) -> (s? t:f=w904:path)
            n560 = Concatenate Strings(w919, " ul / " ("string"), w917, " ms " ("string"), " (" ("string"), w911, ")" ("string")) -> (w913:string)
            "Last calibration" <- w913
            n561 = Open/Create/Replace File(file path (use dialog)=w904, operation (0:open)=T9."open") -> (refnum out=w920:refnum<file>)  [unwired: 4 in, 2 out]
            n562 = Write to Text File(file (use dialog)=w920, text=w913) -> (refnum out=w921:refnum<file>)  [unwired: 2 in, 2 out]
            n563 = Close File(refnum=w921) -> ()  [unwired: 1 in, 2 out]
          }
        }
        n564 = local read "Current mice"() -> (w517:string[][])
        n565 = case shown="True" "Edit mouse list" {
          frame False {
            n566 = property on="Current mice" class="Arr (strict)"("DisabledEnum"=T8."Disabled and Grayed Out" ("Disabled")) -> ()  [unwired: 2 in, 2 out]
          }
          frame True {
            w927 = "List of mice.txt" ("name or relative path")
            n567 = local read "settings folder"() -> (w931:path)
            n568 = property on="Current mice" class="Arr (strict)"("DisabledEnum"=T8."Enabled" ("Disabled")) -> ()  [unwired: 2 in, 2 out]
            n569 = Strip Path(path=w931) -> (stripped path=w928:path)  [unwired: 1 out]
            n570 = Build Path(base path=w931, name or relative path=w927) -> (appended path=w932:path)
            n571 = for {
              tunnel: "Current mice" -> [w938] mode=indexing
              tunnel: [w934] -> w924 mode=indexing
              n572 = Index Array(array=w938, index=0) -> (element=w937:string)
              n573 = Index Array(array=w938, index=1 ("length")) -> (element=w935:string)
              n574 = Concatenate Strings(w937, "-" ("string"), w935) -> (w934:string)
            }
            n575 = call <vilib>:"Check if File or Folder Exists.vi"("path"=w932) -> ("file or folder exists?"=w930:bool, "dup path"=w929:path)  [unwired: 8 in, 1 out]
            n576 = Build Path(base path=w928, name or relative path=w927) -> (appended path=w926:path)
            n577 = Select(t=w929, s=w930, f=w926) -> (s? t:f=w925:path)
            n578 = property on="Mouse name" class="Ring (strict)"("Strings []"=w924) -> ()  [unwired: 2 in, 2 out]
            n579 = call-poly <vilib>:"Write Delimited Spreadsheet.vi"("file path (dialog if empty)"=w925, "2D data"="Current mice") -> ()  [unwired: 12 in, 2 out]
          }
        }
        n580 = local write "Valve open dur. (ms)"("Valve open dur. (ms)") -> ()
        n581 = Format Date/Time String(time format string (%c)="%Y.%m.%d") -> (date/time string=→"Date":string)  [unwired: 2 in]
        n582 = local read "Exit program"() -> (w628:bool)
        n583 = property on="Masking light" class="Enum (strict)"() -> ("RingText.Text"=w535:string)  [unwired: 2 in, 2 out]
        n584 = Concatenate Strings("\nOptical stimulation protocol:\n", w541, "\nVR context:\n", w539) -> (→"Stimulus protocol":string)
        n585 = Array Subset(array=w517, index (row)="Mouse name", length (row)=w614, index (col)=0 ("index 2"), length (col)=w614) -> (w622:string[][])
        n586 = Array Subset(array=w517, index (row)="Mouse name", length (row)=w614, index (col)=1 ("index 2"), length (col)=w614) -> (w619:string[][])
        n587 = Array Subset(array=w517, index (row)="Mouse name", length (row)=w614, index (col)=2 ("index"), length (col)=w614) -> (w613:string[][])
        n588 = Concatenate Strings(w613) -> (w611:string)
        n589 = local write "Run experiment"(FALSE ("Record")) -> ()
        n590 = case shown="True" w628 {
          frame False {
            n591 = flat-sequence {
              frame #0 {
                n592 = Wait (ms)(milliseconds to wait=u32 50) -> ()  [unwired: 1 out]
              }
              frame #1 {
                n593 = local write "Write"(TRUE ("Write")) -> ()
              }
            }
            n594 = local write "read"(FALSE ("read")) -> ()
            n595 = local write "msg tag"("str," ("msg tag")) -> ()
          }
          frame True {
            n596 = while {
              tunnel: [FALSE ("read")] -> w947
              tunnel: [TRUE ("Exit")] -> w946
              stop <- w956 stop-if-true
              n597 = local read "Read loop stopped"() -> (w956:bool)
              n598 = local read "Encoder count"() -> (w954:dbl)
              n599 = Add(x=w954, y=100.0) -> (x+y=w955:dbl)
              n600 = local write "Encoder count"(w955) -> ()
              n601 = Wait (ms)(milliseconds to wait=u32 20) -> ()  [unwired: 1 out]
            }
            n602 = local read "Write loop stopped"() -> (w948:bool)
            n603 = local write "msg tag"("c1" ("msg tag")) -> ()
            n604 = local write "Masking light"(T14."None" ("Masking light")) -> ()
            n605 = case shown="True" w948 {
              frame False {
              }
              frame True {
                n606 = local write "Exit program"(FALSE ("Exit program")) -> ()
                n607 = local write "Exit"(TRUE ("Exit")) -> ()
              }
            }
            n608 = local write "Stop Unity"(w946) -> ()
            n609 = local write "read"(w947) -> ()
          }
        }
        n610 = local read "Stim types"() -> (w524:u16[])
        n611 = Fract/Exp String To Number(string=w611) -> (number=w610:dbl)  [unwired: 3 in, 1 out]
        "Original weight" <- w610
        n612 = local write "Masking light"("Masking light") -> ()
        n613 = local write "Record"("Record Button") -> ()
        n614 = case shown="False" "Record Button" {
          frame False {
          }
          frame True {
            n615 = local read "Unique ID"() -> (w896:i8)
            n616 = Increment(x=w896) -> (x+1=w897:i8)
            n617 = local write "Unique ID"(w897) -> ()
          }
        }
        n618 = Or(x="Start recording", y="Record Button") -> (x .or. y?=w626:bool)
        n619 = Concatenate Strings("Primary masking light: ", w535) -> (→"Masking light prot":string)
        n620 = Concatenate Strings(w622, string[][] [["-"]] ("string"), w619) -> (w601:string)
        "Mouse name 2" <- w601
        n621 = Add Array Elements(numeric array=w524) -> (sum=w523:u16)
        n622 = Divide(x="Weight", y=w610) -> (x/y=w608:dbl)
        n623 = Multiply(x=100.0, y=w608) -> (x*y=→"%":dbl)
        n624 = local write "2P imaging"("2P imaging: NO" ("2P imaging")) -> ()
        n625 = Greater?(x=w523, y=u16 0) -> (0:w521:bool)
        n626 = local write "Comment"("Comment") -> ()
        n627 = call "Is Value Changed.vim"("value"=w601) -> ("changed or first call?"=w600:bool)
        n628 = case shown="True" w600 {
          frame False {
          }
          frame True {
            n629 = local write "Reset water count"(TRUE ("Reset water count")) -> ()
            n630 = local write "Unique ID"(i8 0 ("Unique ID")) -> ()
          }
        }
        n631 = Not(x="Start trigger") -> (.not. x?=→"Boolean 3":bool)
        n632 = property on="plot selector bool 2" class="Bool (strict)"("Value"=w521) -> ()  [unwired: 2 in, 2 out]
        n633 = Select(t=T13."Init recording " ("main program"), s=w626, f=T13."Idle" ("main program")) -> (s? t:f=w625:T13)
        "Boolean 2" <- "Start trigger"
      }
      frame "Init recording " {
        w991 = T8."Disabled" ("Disabled")
        w993 = 0 ("All trials")
        # "Reward zone available?"
        n634 = local read "teleports"() -> (w988:i16[])
        n635 = Index Array(array=w988, index=0) -> (element=w986:i16)
        n636 = local write "Edit mouse list"(FALSE ("Edit mouse list")) -> ()
        n637 = Decrement(x=w986) -> (x-1=w985:i16)
        n638 = local write "Write"(TRUE ("Write")) -> ()
        n639 = local write "read"(TRUE ("read")) -> ()
        n640 = local write "select trial"(FALSE ("Randomize")) -> ()
        n641 = local write "Run experiment"(TRUE ("record")) -> ()
        n642 = local write "Random reward"(FALSE ("Random reward")) -> ()
        n643 = local read "current VR context"() -> (w968:u16)
        n644 = local read "zeward zones"() -> (w969:i16[][])
        n645 = local write "Track position"(w985) -> ()
        n646 = Delete From Array(array=w969, index (row)=w968) -> (deleted portion=w970:i16[])  [unwired: 2 in, 1 out]
        n647 = Decimate 1D Array(w970) -> (w967:i16[], w966:i16[])
        n648 = disable-structure shown="Enabled" {
          disable-tunnel: [w1017 -1 ("All trials")] -> w989
          frame Disabled {
            n649 = local read "VR Mode"() -> (w1018:bool)
            n650 = Select(t=-1 ("All trials"), s=w1018, f=0 ("All trials")) -> (s? t:f=w1017:i32)
          }
          frame Enabled {
          }
        }
        n651 = Add Array Elements(numeric array=w967) -> (sum=w965:i16)
        n652 = Add Array Elements(numeric array=w966) -> (sum=w964:i16)
        n653 = Less?(x=w965, y=w964) -> (x < y?=w960:bool)
        n654 = local read "Context types"() -> (w983:u16[])
        n655 = Select(t=TRUE ("Hybrid licking"), s=w960, f=FALSE ("Active licking")) -> (s? t:f=w961:bool)
        n656 = local write "Stim prot command"(u16 0 ("Mask prot command")) -> ()
        n657 = local write "Trials in session array"(u16[][] [] ("Trials in session array")) -> ()
        n658 = local write "Prev. rew. pos."(0.0 ("Prev. rew. pos.")) -> ()
        n659 = local write "miss trial"(FALSE ("miss trial")) -> ()
        n660 = local write "Water count"(0 ("Water count")) -> ()
        n661 = local write "Active licking"(w961) -> ()
        n662 = local write "Start light stim"(FALSE ("Start light stim")) -> ()
        n663 = local write "Reward given"(u32 10 ("Reward given")) -> ()
        n664 = local write "Hybrid licking"(w961) -> ()
        n665 = local write "Reward zone"(TRUE ("Reward zone")) -> ()
        n666 = local write "Hit trials ctrl."(w993) -> ()
        n667 = local write "Hit trials"(w993) -> ()
        n668 = local write "Hit trials stim."(w993) -> ()
        n669 = local write "Ctrl. count"(w993) -> ()
        n670 = local write "Stim. count"(w993) -> ()
        n671 = Index Array(array=w983, index=0) -> (element=w977:u16)
        n672 = local write "All trials"(w989) -> ()
        n673 = local write "Context command"(w977) -> ()
        n674 = Increment(x=w977) -> (x+1=w982:u16)
        n675 = local read "corridor lengths"() -> (w975:i32[])
        n676 = Number To Decimal String(number=w982) -> (decimal integer string=w980:string)  [unwired: 1 in]
        n677 = local read "teleports"() -> (w976:i16[])
        n678 = Concatenate Strings("c" ("string"), w980) -> (w981:string)
        n679 = local write "Trial counted"(FALSE ("Trial counted")) -> ()
        n680 = local write "msg tag"(w981) -> ()
        n681 = disable-structure shown="Disabled" {
          frame Disabled {
            n682 = local read "Stim types"() -> (w1028:u16[])
            n683 = local read item#-1() -> ()  [unwired: 1 out]
            n684 = Index Array(array=w1028, index=1 ("index (row)")) -> (element=w1030:u16)
            n685 = Add Array Elements(numeric array=w1030) -> (sum=w1029:dbl)
            n686 = Greater?(x=w1029, y=i16 0) -> (0:w1022:bool)
            n687 = Equal?(y=T15."None" ("Stimulus protocol")) -> (x = y?=w1023:bool)  [unwired: 1 in]
            n688 = And(x=w1022, y=w1023) -> (x .and. y?=w1024:bool)
            n689 = case shown="True" w1024 {
              frame False {
              }
              frame True {
                n690 = One Button Dialog(message="No stimulus protocol has been selected!") -> ()  [unwired: 1 in, 1 out]
              }
            }
          }
          frame Enabled {
          }
        }
        n691 = Index Array(array=w976, index=w977) -> (element=w974:i16)
        n692 = Index Array(array=w975, index=w977) -> (element=w973:i32)
        n693 = Subtract(x=w974, y=w973) -> (x-y=w972:i32)
        n694 = local read "SciScan start"() -> (w1002:refnum<k21>)
        n695 = property on="Top Graph" class="XYGraph (strict)"("XScale.Maximum"=w974, "XScale.Minimum"=w972) -> ()  [unwired: 2 in, 2 out]
        n696 = property on="Bottom Graph" class="XYGraph (strict)"("XScale.Maximum"=w974, "XScale.Minimum"=w972) -> ()  [unwired: 2 in, 2 out]
        n697 = property on="Position bar" class="Slide (strict)"("Scale.Maximum"=w974, "Scale.Minimum"=w972) -> ()  [unwired: 2 in, 2 out]
        n698 = call <vilib>:"DAQmx Start Task.vi"("task/channels in"=w1002) -> ("task out"=w1003:refnum<k21>, "error out"=w1000:errorcluster)  [unwired: 13 in]
        n699 = local write "offset tag"("0," ("offset tag")) -> ()
        n700 = call-poly <vilib>:"DAQmx Write.vi"("task/channels in"=w1003, "data"=FALSE, "error in"=w1000) -> ("task out"=w999:refnum<k21>)  [unwired: 10 in, 2 out]
        n701 = disable-structure shown="Disabled" {
          frame Disabled {
            n702 = call <vilib>:"DAQmx Stop Task.vi"() -> ()  [unwired: 14 in, 2 out]
          }
          frame Enabled {
          }
        }
        n703 = property on="Record Button" class="Bool (strict)"("DisabledEnum"=w991) -> ()  [unwired: 2 in, 2 out]
        n704 = property on="Stop recording" class="Bool (strict)"("DisabledEnum"=T8."Enabled" ("Disabled")) -> ()  [unwired: 2 in, 2 out]
        n705 = local write "SciScan start"(w999) -> ()
        n706 = property on="Start recording" class="Bool (strict)"("DisabledEnum"=w991) -> ()  [unwired: 2 in, 2 out]
        n707 = disable-structure shown="Enabled" {
          disable-tunnel: [w1020 TRUE ("VR Mode")] -> w1006
          frame Disabled {
            n708 = local read "VR Mode"() -> (w1020:bool)
          }
          frame Enabled {
          }
        }
        n709 = Select(t=T13."Record VR" ("main program"), s=w1006, f=T13."Record" ("main program")) -> (s? t:f=w1008:T13)
      }
      frame "Stop Recording" {
        w1041 = T8."Enabled" ("Disabled")
        n710 = local read "VR Mode"() -> (w1046:bool)
        n711 = local write "read"(FALSE ("read")) -> ()
        n712 = local write "Run experiment"(FALSE ("Record")) -> ()
        n713 = local write "Start light stim"(FALSE ("Start light stim")) -> ()
        n714 = local write "Timed reward (s)"(u32 0 ("Timed reward (s)")) -> ()
        n715 = local write "Start recording"(FALSE ("Start recording")) -> ()
        n716 = local write "Record Button"(FALSE ("Record Button")) -> ()
        n717 = local write "Repetition"(1 ("Repetition")) -> ()
        n718 = case shown="True" w1046 {
          frame False {
          }
          frame True {
            # "Wait for writing stimulus protocol, etc. to in lab book file"
            n719 = flat-sequence {
              frame #0 {
                n720 = Wait (ms)(milliseconds to wait=u32 100) -> ()  [unwired: 1 out]
              }
              frame #1 {
                n721 = disable-structure shown="Disabled" {
                  frame Disabled {
                    n722 = local write "Masking light"(T14."None" ("Masking light")) -> ()
                  }
                  frame Enabled {
                  }
                }
              }
            }
          }
        }
        n723 = local read "Stop triggers"() -> (w1035:bool)
        n724 = local read "SciScan start"() -> (w1037:refnum<k21>)
        n725 = case shown="True" w1035 {
          tunnel: w1037 -> [w1053 w1060]
          tunnel: [w1052 w1055] -> w1038
          frame False {
            n726 = call-poly <vilib>:"DAQmx Write.vi"("task/channels in"=w1053, "data"=FALSE) -> ("task out"=w1052:refnum<k21>)  [unwired: 11 in, 2 out]
          }
          frame True {
            n727 = flat-sequence {
              tunnel: w1060 -> [w1062]
              tunnel: [w1061] -> w1059
              tunnel: w1059 -> [w1066]
              tunnel: [w1065] -> w1058
              tunnel: w1058 -> [w1070]
              tunnel: [w1069] -> w1057
              tunnel: w1057 -> [w1074]
              tunnel: [w1073] -> w1056
              tunnel: w1056 -> [w1079]
              tunnel: [w1078] -> w1055
              frame #0 {
                n728 = call-poly <vilib>:"DAQmx Write.vi"("task/channels in"=w1062, "data"=FALSE) -> ("task out"=w1061:refnum<k21>)  [unwired: 11 in, 2 out]
                n729 = Wait (ms)(milliseconds to wait=u32 20) -> ()  [unwired: 1 out]
              }
              frame #1 {
                n730 = call-poly <vilib>:"DAQmx Write.vi"("task/channels in"=w1066, "data"=TRUE) -> ("task out"=w1065:refnum<k21>)  [unwired: 11 in, 2 out]
                n731 = Wait (ms)(milliseconds to wait=u32 20) -> ()  [unwired: 1 out]
              }
              frame #2 {
                n732 = call-poly <vilib>:"DAQmx Write.vi"("task/channels in"=w1070, "data"=FALSE) -> ("task out"=w1069:refnum<k21>)  [unwired: 11 in, 2 out]
                n733 = Wait (ms)(milliseconds to wait=u32 50) -> ()  [unwired: 1 out]
              }
              frame #3 {
                n734 = call-poly <vilib>:"DAQmx Write.vi"("task/channels in"=w1074, "data"=TRUE) -> ("task out"=w1073:refnum<k21>)  [unwired: 11 in, 2 out]
                n735 = Wait (ms)(milliseconds to wait=u32 50) -> ()  [unwired: 1 out]
              }
              frame #4 {
                n736 = call-poly <vilib>:"DAQmx Write.vi"("task/channels in"=w1079, "data"=FALSE) -> ("task out"=w1078:refnum<k21>)  [unwired: 11 in, 2 out]
                n737 = Wait (ms)(milliseconds to wait=u32 10) -> ()  [unwired: 1 out]
              }
            }
          }
        }
        n738 = local write "Frame signal 1 rec."(FALSE ("Frame signal")) -> ()
        n739 = local write "Frame signal 2 rec."(FALSE ("Frame signal")) -> ()
        n740 = local write "EyeCam frame signal rec."(FALSE ("Frame signal")) -> ()
        n741 = local write "Record 2P"(FALSE ("SciScan")) -> ()
        n742 = Wait (ms)(milliseconds to wait=u32 100) -> ()  [unwired: 1 out]
        n743 = call <vilib>:"DAQmx Stop Task.vi"("task/channels in"=w1038) -> ("task out"=w1036:refnum<k21>)  [unwired: 13 in, 1 out]
        n744 = local write "SciScan start"(w1036) -> ()
        n745 = property on="Stop recording" class="Bool (strict)"("DisabledEnum"=T8."Disabled" ("Disabled")) -> ()  [unwired: 2 in, 2 out]
        n746 = property on="Record Button" class="Bool (strict)"("DisabledEnum"=w1041) -> ()  [unwired: 2 in, 2 out]
        n747 = property on="Start recording" class="Bool (strict)"("DisabledEnum"=w1041) -> ()  [unwired: 2 in, 2 out]
      }
      frame "Exit program" {
      }
      frame "Record" {
        # "only true if prev. diode pos. <15 cm and reward given changes"
        # "These events happen only once in a trial at the beginning: 10 cm after the diode signal \nand  min ~ 5cm after revard given"
        # "Calculate \"Hit trials\""
        # "These events happen only once in a trial at the second half: 100 cm after diode signal"
        n748 = local read "Reward given"() -> (w1085:u32)
        n749 = local read "VR Mode"() -> (w1098:bool)
        n750 = local read "prev. diode position"() -> (w1090:dbl)
        n751 = case shown="False" w1098 {
          tunnel: [w1128 w1129] -> w1097
          frame True {
            n752 = local read "Prev. rew. pos."() -> (w1128:dbl)
          }
          frame False {
            n753 = local read "prev. diode position"() -> (w1129:dbl)
          }
        }
        n754 = local read "prev. diode position"() -> (w1105:dbl)
        n755 = Not Equal?(x=w1085, y=u32 0) -> (x != y?=w1084:bool)
        n756 = local read "total distance cm"() -> (w1108:sgl[])
        n757 = local read "Trial counted"() -> (w1096:bool)
        n758 = First Call?() -> (First Call?: T/F=w1091:bool)
        n759 = local read "hit trial"() -> (w1095:bool)
        n760 = Not(x=w1091) -> (.not. x?=w1088:bool)
        n761 = Greater?(x=w1090, y=0.0) -> (0:w1087:bool)
        n762 = Not(x=w1096) -> (.not. x?=w1093:bool)
        n763 = Array Max & Min(array=w1108) -> (max value=w1109:sgl)  [unwired: 3 out]
        n764 = call "Is Value Changed.vim"("value"=w1097) -> ("changed or first call?"=w1092:bool)
        n765 = call "Is Value Changed.vim"("value"=w1084) -> ("changed or first call?"=w1103:bool)
        n766 = Subtract(x=w1109, y=w1105) -> (x-y=w1106:dbl)
        n767 = Compound Arithmetic op=AND(w1092, w1093, w1088, w1087) -> (w1094:bool)
        n768 = Less?(x=w1106, y=15.0) -> (x < y?=w1104:bool)
        n769 = case shown="True" w1094 {
          frame False {
          }
          frame True {
            n770 = stacked-sequence {
              frame #0 {
                n771 = local read "Reward given"() -> (w1132:u32)
                n772 = Not Equal?(x=w1132, y=u32 0) -> (x != y?=w1130:bool)
                n773 = local read "Stim trial"() -> (w1133:bool)
                n774 = local read "Stim trial"() -> (w1135:bool)
                n775 = local read "Stim trial"() -> (w1138:bool)
                n776 = local read "hit trial"() -> (w1140:bool)
                n777 = local read "hit trial"() -> (w1136:bool)
                n778 = case shown="True" w1133 {
                  frame False {
                    n779 = local read "Ctrl. count"() -> (w1143:i32)
                    n780 = Increment(x=w1143) -> (x+1=w1144:i32)
                    n781 = local write "Ctrl. count"(w1144) -> ()
                  }
                  frame True {
                    n782 = local read "Stim. count"() -> (w1146:i32)
                    n783 = Increment(x=w1146) -> (x+1=w1145:i32)
                    n784 = local write "Stim. count"(w1145) -> ()
                  }
                }
                n785 = local read "All trials"() -> (w1142:i32)
                n786 = Not(x=w1135) -> (.not. x?=w1134:bool)
                n787 = Compound Arithmetic op=AND(w1130, w1140, w1134) -> (w1139:bool)
                n788 = Compound Arithmetic op=AND(w1130, w1136, w1138) -> (w1137:bool)
                n789 = Increment(x=w1142) -> (x+1=w1141:i32)
                n790 = case shown="True" w1139 {
                  frame False {
                  }
                  frame True {
                    n791 = local read "Hit trials ctrl."() -> (w1149:i32)
                    n792 = Increment(x=w1149) -> (x+1=w1150:i32)
                    n793 = local write "Hit trials ctrl."(w1150) -> ()
                  }
                }
                n794 = case shown="True" w1137 {
                  frame False {
                  }
                  frame True {
                    n795 = local read "Hit trials stim."() -> (w1147:i32)
                    n796 = Increment(x=w1147) -> (x+1=w1148:i32)
                    n797 = local write "Hit trials stim."(w1148) -> ()
                  }
                }
                n798 = local write "All trials"(w1141) -> ()
              }
              frame #1 {
                w1181 = TRUE ("Trial counted")
                # "Build trial type array counting trials \nat the beginning"
                n799 = local read "Stim array length"() -> (w1151:u16)
                n800 = local read "Stim array length"() -> (w1163:u16)
                n801 = local read "All trials"() -> (w1155:i32)
                n802 = local read "shuffled array"() -> (w1158:i16[])
                n803 = local read "Stim types"() -> (w1171:u16[])
                n804 = local read "All trials"() -> (w1152:i32)
                n805 = local write "Trial counted"(w1181) -> ()
                n806 = local write "select trial"(w1181) -> ()
                n807 = Quotient & Remainder(x=w1155, y=w1163) -> (x-y*floor(x/y)=w1160:i32)  [unwired: 1 out]
                n808 = Decrement(x=w1163) -> (x-1=w1159:u16)
                n809 = Increment(x=w1152) -> (x+1=w1156:i32)
                n810 = Quotient & Remainder(x=w1152, y=w1151) -> (x-y*floor(x/y)=w1154:i32)  [unwired: 1 out]
                n811 = Quotient & Remainder(x=w1156, y=w1151) -> (x-y*floor(x/y)=w1153:i32)  [unwired: 1 out]
                n812 = Equal?(x=w1160, y=w1159) -> (x = y?=w1161:bool)
                n813 = Index Array(array=w1158, index=w1154) -> (element=w1166:i16)
                n814 = call "Shuffle 1D Array.vim"("array"=w1158) -> ("shuffled array"=w1162:i16[])  [unwired: 4 in]
                n815 = Select(t=w1162, s=w1161, f=w1158) -> (s? t:f=w1157:i16[])
                n816 = Index Array(array=w1157, index=w1153) -> (element=w1165:i16)
                n817 = Index Array(array=w1171, index=w1166) -> (element=w1164:u16)
                n818 = Index Array(array=w1171, index=w1165) -> (element=w1170:u16)
                n819 = local write "shuffled array"(w1157) -> ()
                n820 = local write "Stim prot command"(w1164) -> ()
                n821 = Build Array(w1164, w1164) -> (w1178:u16[])
                n822 = property on="Stim protocols" class="Ring (strict)"() -> ("Strings []"=w1177:string[])  [unwired: 2 in, 2 out]
                n823 = local read "Trials in session array"() -> (w1179:u16[][])
                n824 = Greater?(x=w1164, y=i8 0) -> (0:w1174:bool)
                n825 = Select(t=TRUE, s=w1174, f=FALSE) -> (s? t:f=w1173:bool)
                n826 = local read "All trials"() -> (w1172:i32)
                n827 = Index Array(array=w1177, index=w1164) -> (element=w1176:string)
                n828 = Index Array(array=w1177, index=w1170) -> (element=w1175:string)
                n829 = local write "Stim trial"(w1173) -> ()
                n830 = local write "Current stim. protocol"(w1176) -> ()
                n831 = local write "Next trial stim. protocol"(w1175) -> ()
                n832 = Insert Into Array(array=w1179, index (row)=w1172, new element=w1178) -> (w1180:u16[][])  [unwired: 1 in]
                n833 = local write "Trials in session array"(w1180) -> ()
              }
            }
          }
        }
        n834 = Compound Arithmetic op=AND(w1103, w1095, w1104) -> (w1102:bool)
        n835 = case shown="True" w1102 {
          frame False {
          }
          frame True {
            n836 = local read "Hit trials"() -> (w1189:i32)
            n837 = Increment(x=w1189) -> (x+1=w1188:i32)
            n838 = local write "Hit trials"(w1188) -> ()
          }
        }
        n839 = local read "VR Mode"() -> (w1101:bool)
        n840 = local read "total distance cm"() -> (w1111:sgl[])
        n841 = case shown="False" w1101 {
          tunnel: [140.0 ("y") w1185] -> w1100
          tunnel: [w1182 w1184] -> w1099
          frame False {
            n842 = local read "prev. diode position"() -> (w1182:dbl)
          }
          frame True {
            n843 = local read "Prev. rew. pos."() -> (w1184:dbl)
            n844 = local read "Reward freq. (cm)"() -> (w1187:u32)
            n845 = Subtract(x=w1187, y=15.0) -> (x-y=w1185:dbl)
          }
        }
        n846 = local read "Trial counted"() -> (w1119:bool)
        n847 = Array Max & Min(array=w1111) -> (max value=w1110:sgl)  [unwired: 3 out]
        n848 = Subtract(x=w1110, y=w1099) -> (x-y=w1120:dbl)
        n849 = Greater?(x=w1120, y=w1100) -> (0:w1118:bool)
        n850 = And(x=w1118, y=w1119) -> (x .and. y?=w1117:bool)
        n851 = case shown="True" w1117 {
          frame False {
          }
          frame True {
            n852 = local write "Trial counted"(FALSE ("Trial counted")) -> ()
          }
        }
        n853 = local read "Record 2P"() -> (w1121:bool)
        n854 = local read "Stop recording"() -> (w1124:bool)
        n855 = case shown="True" w1121 {
          frame False {
          }
          frame True {
            n856 = local read "SciScan start"() -> (w1192:refnum<k21>)
            n857 = local write "2P imaging"("2P imaging: YES" ("2P imaging")) -> ()
            n858 = call-poly <vilib>:"DAQmx Write.vi"("task/channels in"=w1192, "data"=TRUE) -> ()  [unwired: 11 in, 3 out]
          }
        }
        n859 = local read "Exit program"() -> (w1125:bool)
        n860 = local read "Hit trials"() -> (w1116:i32)
        n861 = local read "All trials"() -> (w1115:i32)
        n862 = Divide(x=w1116, y=w1115) -> (x/y=w1113:dbl)
        "P hit trials" <- w1113
        n863 = Or(x=w1124, y=w1125) -> (x .or. y?=w1122:bool)
        n864 = Multiply(x=w1113, y=100.0) -> (x*y=→"Hit trials %":dbl)
        n865 = Select(t=T13."Stop Recording" ("main program"), s=w1122, f=T13."Record" ("main program")) -> (s? t:f=w1123:T13)
      }
      frame "Record VR" {
        (unwired) 0 ("index")
        # "These computations run only once in a trial at the very beginning"
        n866 = disable-structure shown="Disabled" {
          frame Disabled {
            n867 = local read "Stim array length"() -> (w1289:u16)
            n868 = local read "All trials"() -> (w1291:i32)
            n869 = local read item#-1() -> (w1296)
            n870 = Quotient & Remainder(x=w1291, y=w1289) -> (x-y*floor(x/y)=w1292:i32)  [unwired: 1 out]
            n871 = Decrement(x=w1289) -> (x-1=w1290:u16)
            n872 = Equal?(x=w1292, y=w1290) -> (x = y?=w1293:bool)
            n873 = Equal?(x=w1292, y=0.0) -> (x = y?=w1295:bool)
            n874 = Compound Arithmetic op=AND(w1295, w1296) -> (w1294:bool)
            n875 = case shown="True" w1293 {
              frame False {
              }
              frame True {
              }
            }
            n876 = case shown="True" w1294 {
              frame False {
              }
              frame True {
                n877 = local read "shuffled array"() -> (w1299:i16[])
                n878 = call "Shuffle 1D Array.vim"("array"=w1299) -> ("shuffled array"=w1298:i16[])  [unwired: 4 in]
                n879 = local write "shuffled array"(w1298) -> ()
                n880 = local write item#-1(FALSE ("Shuffle")) -> ()
              }
            }
          }
          frame Enabled {
          }
        }
        n881 = local read "Context command"() -> (w1221:u16)
        n882 = local read "All trials"() -> (w1207:i32)
        n883 = local read "corridor lengths"() -> (w1223:i32[])
        n884 = local read "teleports"() -> (w1224:i16[])
        n885 = Greater Or Equal To 0?(x=w1207) -> ()  [unwired: 1 out]
        n886 = Index Array(array=w1224, index=w1221) -> (element=w1222:i16)
        n887 = Index Array(array=w1223, index=w1221) -> (element=w1220:i32)
        n888 = Divide(x=w1220, y=2) -> (x/y=w1218:dbl)
        n889 = Subtract(x=w1222, y=w1218) -> (x-y=w1217:dbl)
        n890 = disable-structure shown="Enabled" {
          disable-tunnel: [w1237 w1241] -> w1225
          disable-tunnel: w1217 -> [w1233 _]
          frame Disabled {
            n891 = local read "Track position"() -> (w1232:sgl)
            n892 = local read "Trial counted"() -> (w1238:bool)
            n893 = Equal?(x=w1238, y=FALSE) -> (x = y?=w1235:bool)
            n894 = Less?(x=w1232, y=w1233) -> (x < y?=w1236:bool)
            n895 = Compound Arithmetic op=AND(w1235, w1236) -> (w1237:bool)
          }
          frame Enabled {
            n896 = local read "Track position"() -> (w1240:sgl)
            n897 = call "Is New Trial - trial counting.vi"("Position data"=w1240, "Minimum value drop"=-20.0) -> ("Boolean"=w1241:bool)
          }
        }
        n898 = case shown="True" w1225 {
          frame False {
          }
          frame True {
            n899 = stacked-sequence {
              frame #0 {
                # "Build Trials in session array counting trials \nat the beginning"
                n900 = local read "Stim array length"() -> (w1307:u16)
                n901 = local read "Stim array length"() -> (w1310:u16)
                n902 = local read "All trials"() -> (w1319:i32)
                n903 = local read "shuffled array"() -> (w1304:i16[])
                n904 = local read "Stim types"() -> (w1330:u16[])
                n905 = local read "Context types"() -> (w1317:u16[])
                n906 = local read "Session length"() -> (w1316:u16)
                n907 = local read "Shuffle stim trials"() -> (w1302:bool)
                n908 = Increment(x=w1319) -> (x+1=w1306:i32)
                n909 = Quotient & Remainder(x=w1306, y=w1307) -> (x-y*floor(x/y)=w1309:i32)  [unwired: 1 out]
                n910 = local write "All trials"(w1306) -> ()
                n911 = Decrement(x=w1307) -> (x-1=w1308:u16)
                n912 = Increment(x=w1306) -> (x+1=w1311:i32)
                n913 = Quotient & Remainder(x=w1306, y=w1310) -> (x-y*floor(x/y)=w1332:i32)  [unwired: 1 out]
                n914 = Increment(x=w1306) -> (x+1=w1318:i32)
                n915 = Quotient & Remainder(x=w1311, y=w1310) -> (x-y*floor(x/y)=w1312:i32)  [unwired: 1 out]
                n916 = Equal?(x=w1309, y=w1308) -> (x = y?=w1303:bool)
                n917 = Quotient & Remainder(x=w1318, y=w1316) -> (x-y*floor(x/y)=w1325:i32)  [unwired: 1 out]
                n918 = Quotient & Remainder(x=w1306, y=w1316) -> (x-y*floor(x/y)=w1315:i32)  [unwired: 1 out]
                n919 = And(x=w1303, y=w1302) -> (x .and. y?=w1301:bool)
                n920 = Index Array(array=w1304, index=w1332) -> (element=w1329:i16)
                n921 = case shown="True" w1301 {
                  tunnel: [w1342 w1344] -> w1305
                  tunnel: w1304 -> [w1342 w1343]
                  frame False {
                  }
                  frame True {
                    n922 = call "Shuffle 1D Array.vim"("array"=w1343) -> ("shuffled array"=w1344:i16[])  [unwired: 4 in]
                  }
                }
                n923 = Index Array(array=w1305, index=w1312) -> (element=w1328:i16)
                n924 = Index Array(array=w1330, index=w1329) -> (element=w1326:u16)
                n925 = Index Array(array=w1330, index=w1328) -> (element=w1331:u16)
                n926 = Index Array(array=w1317, index=w1325) -> (element=w1314:u16)
                n927 = Index Array(array=w1317, index=w1315) -> (element=w1313:u16)
                n928 = local read "Trials in session array"() -> (w1341:u16[][])
                n929 = Build Array(w1326, w1313) -> (w1327:u16[])
                n930 = local write "current VR context"(w1313) -> ()
                n931 = local write "shuffled array"(w1305) -> ()
                n932 = property on="Stim protocols" class="Ring (strict)"() -> ("Strings []"=w1340:string[])  [unwired: 2 in, 2 out]
                n933 = Increment(x=w1314) -> (x+1=w1321:u16)
                n934 = Greater?(x=w1326, y=u16 0) -> (0:w1337:bool)
                n935 = local write "Context command"(w1314) -> ()
                n936 = Number To Decimal String(number=w1321) -> (decimal integer string=w1324:string)  [unwired: 1 in]
                n937 = Index Array(array=w1340, index=w1326) -> (element=w1339:string)
                n938 = Index Array(array=w1340, index=w1331) -> (element=w1338:string)
                n939 = Select(t=TRUE, s=w1337, f=FALSE) -> (s? t:f=w1336:bool)
                n940 = local write "Stim prot command"(w1326) -> ()
                n941 = local write "Current stim. protocol"(w1339) -> ()
                n942 = local write "Next trial stim. protocol"(w1338) -> ()
                n943 = local write "Stim trial"(w1336) -> ()
                n944 = Concatenate Strings("c" ("string"), w1324) -> (w1323:string)
                n945 = Insert Into Array(array=w1341, index (row)=w1306, new element=w1327) -> (w1320:u16[][])  [unwired: 1 in]
                n946 = local write "msg tag"(w1323) -> ()
                n947 = local write "Trials in session array"(w1320) -> ()
              }
              frame #1 {
                w1348 = TRUE ("Trial counted")
                n948 = local read "Reward given"() -> (w1347:u32)
                n949 = local write "Trial counted"(w1348) -> ()
                n950 = local write "select trial"(w1348) -> ()
                n951 = Not Equal?(x=w1347, y=u32 0) -> (x != y?=w1345:bool)
                n952 = local read "Stim trial"() -> (w1349:bool)
                n953 = local read "Stim trial"() -> (w1351:bool)
                n954 = local read "Stim trial"() -> (w1354:bool)
                n955 = local read "hit trial"() -> (w1356:bool)
                n956 = local read "hit trial"() -> (w1352:bool)
                n957 = case shown="True" w1349 {
                  frame False {
                    n958 = local read "Ctrl. count"() -> (w1357:i32)
                    n959 = Increment(x=w1357) -> (x+1=w1358:i32)
                    n960 = local write "Ctrl. count"(w1358) -> ()
                  }
                  frame True {
                    n961 = local read "Stim. count"() -> (w1360:i32)
                    n962 = Increment(x=w1360) -> (x+1=w1359:i32)
                    n963 = local write "Stim. count"(w1359) -> ()
                  }
                }
                n964 = Not(x=w1351) -> (.not. x?=w1350:bool)
                n965 = Compound Arithmetic op=AND(w1345, w1356, w1350) -> (w1355:bool)
                n966 = Compound Arithmetic op=AND(w1345, w1352, w1354) -> (w1353:bool)
                n967 = case shown="True" w1355 {
                  frame False {
                  }
                  frame True {
                    n968 = local read "Hit trials ctrl."() -> (w1363:i32)
                    n969 = Increment(x=w1363) -> (x+1=w1364:i32)
                    n970 = local write "Hit trials ctrl."(w1364) -> ()
                  }
                }
                n971 = case shown="True" w1353 {
                  frame False {
                  }
                  frame True {
                    n972 = local read "Hit trials stim."() -> (w1361:i32)
                    n973 = Increment(x=w1361) -> (x+1=w1362:i32)
                    n974 = local write "Hit trials stim."(w1362) -> ()
                  }
                }
              }
            }
          }
        }
        n975 = local read "Record loop state"() -> (w1215:T7)
        n976 = local read "Record 2P"() -> (w1213:bool)
        n977 = Equal?(x=w1215, y=Record_enum."Record VR" ("Record loop state")) -> (x = y?=w1214:bool)
        n978 = disable-structure shown="Disabled" {
          disable-tunnel: w1217 -> [w1243 _]
          frame Disabled {
            # "These computations run only once in a trial when the mouse enters to the RZ"
            n979 = local read "Track position"() -> (w1242:sgl)
            n980 = local read "select trial"() -> (w1244:bool)
            n981 = Greater?(x=w1242, y=w1243) -> (0:w1245:bool)
            n982 = Compound Arithmetic op=AND(w1245, w1244) -> (w1246:bool)
            n983 = case shown="True" w1246 {
              frame True {
                w1247 = FALSE ("Randomize")
                n984 = disable-structure shown="Disabled" {
                  frame Disabled {
                    n985 = local read "Stim array length"() -> (w1277:u16)
                    n986 = local read "shuffled array"() -> (w1283:i16[])
                    n987 = local read "Stim types"() -> (w1279:u16[])
                    n988 = local read "All trials"() -> (w1284:i32)
                    n989 = Quotient & Remainder(x=w1284, y=w1277) -> (x-y*floor(x/y)=w1282:i32)  [unwired: 1 out]
                    n990 = Index Array(array=w1283, index=w1282) -> (element=w1278:i16)
                    n991 = Index Array(array=w1279, index (row)=1, index (col)=w1278) -> (element=w1276:u16)
                    n992 = Index Array(array=w1279, index (row)=0, index (col)=w1278) -> (element=w1274:u16)
                    n993 = Greater?(x=w1274, y=u16 0) -> (0:w1275:bool)
                    n994 = local write "Stim prot command"(w1274) -> ()
                    n995 = Select(t=TRUE ("Beaconed"), s=w1275, f=FALSE) -> (s? t:f=w1270:bool)
                    n996 = local write item#-1(w1276) -> ()
                    n997 = local write "Stim trial"(w1270) -> ()
                  }
                  frame Enabled {
                  }
                }
                n998 = disable-structure shown="Disabled" {
                  frame Disabled {
                    n999 = local read "VR start pos"() -> (w1248:T4)
                    n1000 = case shown="\"Random of 2\"" w1248 {
                      tunnel: [w1251 "0," w1262] -> w1249
                      frame "Random of 4", Default {
                        n1001 = local write "Random start pos"(TRUE ("Random start pos")) -> ()
                        n1002 = Build Array("0,", "2,", "4,", "6,") -> (w1257:string[])
                        n1003 = call "Shuffle 1D Array.vim"("array"=w1257) -> ("shuffled array"=w1258:string[])  [unwired: 4 in]
                        n1004 = Index Array(array=w1258, index=0) -> (element=w1251:string)
                      }
                      frame "Non-random" {
                        n1005 = local write "Random start pos"(TRUE ("Random start pos")) -> ()
                      }
                      frame "Random of 2" {
                        n1006 = local write "Random start pos"(TRUE ("Random start pos")) -> ()
                        n1007 = Build Array("0,", "6,", "0,", "6,") -> (w1265:string[])
                        n1008 = call "Shuffle 1D Array.vim"("array"=w1265) -> ("shuffled array"=w1263:string[])  [unwired: 4 in]
                        n1009 = Index Array(array=w1263, index=0) -> (element=w1262:string)
                      }
                    }
                    n1010 = local write "offset tag"(w1249) -> ()
                  }
                  frame Enabled {
                  }
                }
                n1011 = local write "Trial counted"(w1247) -> ()
                n1012 = local write "select trial"(w1247) -> ()
              }
              frame False {
              }
            }
          }
          frame Enabled {
          }
        }
        n1013 = And(x=w1213, y=w1214) -> (x .and. y?=w1195:bool)
        n1014 = call "Is Value Changed.vim"("value"=w1195) -> ("changed or first call?"=w1194:bool)
        n1015 = And(x=w1195, y=w1194) -> (x .and. y?=w1196:bool)
        n1016 = local read "corridor lengths"() -> (w1204:i32[])
        n1017 = case shown="True" w1196 {
          frame False {
          }
          frame True {
            n1018 = local read "SciScan start"() -> (w1368:refnum<k21>)
            n1019 = local read "Start trigger"() -> (w1365:bool)
            n1020 = local write "2P imaging"("2P imaging: YES" ("2P imaging")) -> ()
            n1021 = call-poly <vilib>:"DAQmx Write.vi"("task/channels in"=w1368, "data"=TRUE) -> ("task out"=w1366:refnum<k21>)  [unwired: 11 in, 2 out]
            n1022 = case shown="True" w1365 {
              tunnel: w1366 -> [_ w1371]
              frame False {
              }
              frame True {
                n1023 = flat-sequence {
                  tunnel: w1371 -> [w1373]
                  tunnel: [w1373] -> w1370
                  tunnel: w1370 -> [w1374]
                  frame #0 {
                    n1024 = Wait (ms)(milliseconds to wait=u32 50) -> ()  [unwired: 1 out]
                  }
                  frame #1 {
                    n1025 = call-poly <vilib>:"DAQmx Write.vi"("task/channels in"=w1374, "data"=FALSE) -> ()  [unwired: 11 in, 3 out]
                  }
                }
              }
            }
          }
        }
        n1026 = disable-structure shown="Disabled" {
          frame Disabled {
            # "Wait to make sure DAQ recording \nis started before saving images"
            n1027 = while {
              stop <- w1286 stop-if-true
              n1028 = Wait (ms)(milliseconds to wait=u32 10) -> ()  [unwired: 1 out]
              n1029 = local read "Record loop state"() -> (w1288:T7)
              n1030 = Equal?(x=w1288, y=Record_enum."Record VR" ("Record loop state")) -> (x = y?=w1286:bool)
            }
          }
          frame Enabled {
          }
        }
        n1031 = local read "teleports"() -> (w1206:i16[])
        n1032 = Index Array(array=w1206, index=0) -> (element=w1203:i16)
        n1033 = Index Array(array=w1204) -> (element=w1202:i32)  [unwired: 1 in]
        n1034 = local read "Track position"() -> (w1199:sgl)
        n1035 = Subtract(x=w1203, y=w1202) -> (x-y=w1201:i32)
        n1036 = local read "Session length"() -> (w1211:u16)
        n1037 = local read "Auto stop recording"() -> (w1210:bool)
        n1038 = local read "All trials"() -> (w1212:i32)
        n1039 = Add(x=50, y=w1201) -> (x+y=w1198:i32)
        n1040 = Greater?(x=w1199, y=w1198) -> (0:w1197:bool)
        n1041 = Equal?(x=w1212, y=w1211) -> (x = y?=w1209:bool)
        n1042 = local read "Stop recording"() -> (w1226:bool)
        n1043 = local read "Exit program"() -> (w1227:bool)
        n1044 = Compound Arithmetic op=AND(w1197, w1210, w1209) -> (w1208:bool)
        n1045 = Compound Arithmetic op=OR(w1208, w1226, w1227) -> (w1230:bool)
        n1046 = Select(t=T13."Stop Recording" ("main program"), s=w1230, f=T13."Record VR" ("main program")) -> (s? t:f=w1231:T13)
      }
    }
    n1047 = Wait (ms)(milliseconds to wait=u32 3) -> ()  [unwired: 1 out]
    n1048 = local read "Exit"() -> (w268:bool)
  }
  n1049 = while {
    shift-right: [w1403] -> _
    shift-left: w72 -> [w1402]
    shift-right: [w1399] -> _
    shift-left: _ -> [w1396]
    shift-right: [w1390] -> _
    shift-left: _ -> [w1395]
    shift-right: [w1398] -> _
    shift-left: _ -> [w1392]
    shift-right: [w1397] -> _
    shift-left: _ -> [w1391]
    shift-right: [w1394] -> _
    shift-left: _ -> [w1393]
    shift-right: [w1389] -> _
    shift-left: _ -> [w1388]
    shift-right: [w1385] -> _
    shift-left: _ -> [w1387]
    shift-right: [w1384] -> _
    shift-left: _ -> [w1386]
    shift-right: [w1383] -> _
    shift-left: 0.0 -> [w1382]
    shift-right: [w1381] -> _
    shift-left: _ -> [w1379]
    shift-right: [w1380] -> _
    shift-left: _ -> [w1378]
    shift-right: [w1377] -> _
    shift-left: _ -> [w1376]
    stop <- w1400 stop-if-true
    n1050 = case shown="\"Init data acquisition\"" w1402 {
      selector: w1402 -> [w1496 _ w1579 w1610 w1869 w1995]
      tunnel: [w1492 w1542 w1580 Record_enum."Idle" ("Record enum") w1870 w1996] -> w1403
      tunnel: [FALSE ("Exit") FALSE ("Exit") w1578 FALSE ("Exit") FALSE ("Exit") FALSE ("Exit")] -> w1400
      tunnel: [w1443 w1551 w1577 refnum<k21> refnum ("task out") w1851 w1992] -> w1399
      tunnel: [w1441 w1550 w1576 w1599 w1850 w1991] -> w1390
      tunnel: [w1437 w1549 w1573 refnum<k21> refnum ("task out") w1844 w1988] -> w1398
      tunnel: [w1439 w1548 w1572 w1598 w1843 w1987] -> w1397
      tunnel: w1396 -> [w1444 _ w1577 w1602 w1858 w1992]
      tunnel: w1395 -> [w1442 _ w1576 w1603 w1857 w1991]
      tunnel: [w1490 dbl[] [] w1575 w1608 w1782 w1990] -> w1394
      tunnel: w1393 -> [w1490 _ w1575 w1608 w1793 w1990]
      tunnel: w1392 -> [w1438 _ w1573 w1605 w1853 w1988]
      tunnel: w1391 -> [w1440 _ w1572 w1604 w1852 w1987]
      tunnel: [w1489 w1547 w1574 w1607 w1804 w1989] -> w1389
      tunnel: w1388 -> [w1489 _ w1574 w1607 w1840 w1989]
      tunnel: w1387 -> [_ _ _ _ w1829 _]
      tunnel: w1386 -> [_ _ _ _ w1825 _]
      tunnel: [0.0 0.0 0.0 0.0 w1831 0.0] -> w1385
      tunnel: [0.0 0.0 0.0 0.0 w1830 0.0] -> w1384
      tunnel: [w1486 w1537 w1568 w1594 w1808 w1984] -> w1383
      tunnel: w1382 -> [w1486 w1537 w1568 w1594 _ w1984]
      tunnel: [w1435 w1527 w1567 refnum<k21> refnum ("task out") w1800 w1983] -> w1381
      tunnel: [w1433 w1526 w1566 w1589 w1805 w1982] -> w1380
      tunnel: w1379 -> [w1436 _ w1567 w1592 w1803 w1983]
      tunnel: w1378 -> [w1434 _ w1566 w1591 w1806 w1982]
      tunnel: [w1461 dbl[] [] ("data") w1565 w1584 w1758 w1981] -> w1377
      tunnel: w1376 -> [w1461 _ w1565 w1584 _ w1981]
      frame "Init recording" {
        w1420 = " Hz" ("string")
        w1423 = "\n" ("string")
        w1406 = "   " ("string")
        w1455 = "-" ("string")
        # "Create a \"header\" for the lab book file from those variables that do not change during the recording"
        n1051 = local write "Record loop state"(w1496) -> ()
        n1052 = local read "Weight"() -> (w1474:dbl)
        n1053 = local read "%"() -> (w1472:dbl)
        n1054 = local read "Original weight"() -> (w1476:dbl)
        n1055 = Number To Fractional String(number=w1472, precision (6)=i16 2) -> (F-format string=w1473:string)  [unwired: 2 in]
        n1056 = Number To Fractional String(number=w1474, precision (6)=i16 1) -> (F-format string=w1475:string)  [unwired: 2 in]
        n1057 = local read "Last calibration"() -> (w1479:string)
        n1058 = Number To Fractional String(number=w1476, precision (6)=i16 1) -> (F-format string=w1477:string)  [unwired: 2 in]
        n1059 = Concatenate Strings("Weight: " ("string"), w1473, " %   ( " ("string"), w1475, " g ; weight before water restriction: " ("string"), w1477, " g)" ("string")) -> (w1464:string)
        n1060 = local read "Sample rate"() -> (w1429:dbl)
        n1061 = case shown="True" FALSE {
          tunnel: ["" w1501] -> w1456
          frame False {
          }
          frame True {
            n1062 = disable-structure shown="Disabled" {
              disable-tunnel: [w1505 _] -> w1501
              frame Disabled {
                n1063 = local read "VR Mode"() -> ()  [unwired: 1 out]
                n1064 = local read "zeward zones"() -> ()  [unwired: 1 out]
                n1065 = Number To Decimal String() -> (decimal integer string=w1504:string)  [unwired: 2 in]
                n1066 = Concatenate Strings("-" ("string"), w1504, "cm" ("string")) -> (w1505:string)
              }
              frame Enabled {
              }
            }
          }
        }
        n1067 = local read "Loop rate"() -> (w1428:dbl)
        n1068 = Concatenate Strings("Last calibration of water valve: " ("string"), w1479) -> (w1462:string)
        n1069 = Number To Decimal String(number=w1429) -> (decimal integer string=w1426:string)  [unwired: 1 in]
        n1070 = Number To Decimal String(number=w1428) -> (decimal integer string=w1422:string)  [unwired: 1 in]
        n1071 = local read "Software version"() -> (w1463:string)
        n1072 = local read "Mouse name 2"() -> (w1405:string)
        n1073 = local read "User profile"() -> (w1404:string)
        n1074 = call <vilib>:"DAQmx Stop Task.vi"("task/channels in"=w1444, "error in"=w1442) -> ("task out"=w1450:refnum<k21>, "error out"=w1449:errorcluster)  [unwired: 12 in]
        n1075 = Concatenate Strings("Sampling rate: " ("string"), w1426, w1420, " Loop rate: " ("string"), w1422, w1420) -> (w1425:string)
        n1076 = Format Date/Time String(time format string (%c)="%Y%m%d") -> (date/time string=w1418:string)  [unwired: 2 in]
        n1077 = Format Date/Time String(time format string (%c)="%Y.%m.%d %H:%M:%S") -> (date/time string=w1407:string)  [unwired: 2 in]
        n1078 = call <vilib>:"DAQmx Start Task.vi"("task/channels in"=w1450, "error in"=w1449) -> ("task out"=w1443:refnum<k21>, "error out"=w1441:errorcluster)  [unwired: 12 in]
        n1079 = Concatenate Strings(w1407, w1406, w1405, w1406, w1404, w1423, w1423, w1464, w1423, w1462, w1423, w1463, w1423, w1425, w1423, "\n******************************" ("string"), w1423, w1423) -> (w1481:string)
        n1080 = local read "Mouse name 2"() -> (w1460:string)
        n1081 = local read "Recording folder"() -> (w1414:path)
        n1082 = local read "Unique ID"() -> (w1451:i8)
        n1083 = call <vilib>:"DAQmx Stop Task.vi"("task/channels in"=w1438, "error in"=w1440) -> ("task out"=w1447:refnum<k21>, "error out"=w1448:errorcluster)  [unwired: 12 in]
        n1084 = local write "Header"(w1481) -> ()
        n1085 = local write "Lab book notes"(w1481) -> ()
        n1086 = Format Date/Time String(time format string (%c)="%Y.%m.%d") -> (date/time string=w1410:string)  [unwired: 2 in]
        n1087 = Format Into String(format string="%02d", w1451) -> (resulting string=w1452:string)  [unwired: 2 in, 1 out]
        n1088 = call <vilib>:"DAQmx Start Task.vi"("task/channels in"=w1447, "error in"=w1448) -> ("task out"=w1437:refnum<k21>, "error out"=w1439:errorcluster)  [unwired: 12 in]
        n1089 = local read "Comment"() -> (w1454:string)
        n1090 = Match Pattern(string=w1460, regular expression="-") -> (before substring=w1458:string, after substring=w1457:string)  [unwired: 1 in, 2 out]
        n1091 = Strip Path(path=w1414) -> (stripped path=w1413:path)  [unwired: 1 out]
        n1092 = Build Path(base path=w1413, name or relative path="PupilData") -> (appended path=w1411:path)
        n1093 = call <vilib>:"DAQmx Stop Task.vi"("task/channels in"=w1436, "error in"=w1434) -> ("task out"=w1446:refnum<k21>, "error out"=w1445:errorcluster)  [unwired: 12 in]
        n1094 = Build Path(base path=w1414, name or relative path=w1410) -> (appended path=w1499:path)
        n1095 = Build Path(base path=w1411, name or relative path=w1410) -> (appended path=w1409:path)
        n1096 = Concatenate Strings(w1458, w1455, w1418, w1455, w1452, w1455, w1457, w1456, w1455, w1454) -> (w1416:string)
        n1097 = call <vilib>:"DAQmx Start Task.vi"("task/channels in"=w1446, "error in"=w1445) -> ("task out"=w1435:refnum<k21>, "error out"=w1433:errorcluster)  [unwired: 12 in]
        n1098 = call <vilib>:"Check if File or Folder Exists.vi"("path"=w1499) -> ("file or folder exists?"=w1498:bool, "dup path"=w1497:path)  [unwired: 8 in, 1 out]
        n1099 = Format Date/Time String(time format string (%c)="Session start: %H:%M:%S\n") -> (date/time string=→"Session start:":string)  [unwired: 2 in]
        n1100 = case shown="False" w1498 {
          tunnel: [w1514 w1516] -> w1415
          tunnel: w1497 -> [w1514 w1515]
          frame True {
          }
          frame False {
            n1101 = Create Folder(path (use dialog)=w1515) -> (created path=w1516:path)  [unwired: 2 in, 2 out]
          }
        }
        n1102 = local write "Pupil Exp day folder"(w1409) -> ()
        n1103 = Concatenate Strings(w1416, ".tdms") -> (w1480:string)
        n1104 = Concatenate Strings(w1416, ".txt" ("string")) -> (w1484:string)
        n1105 = Build Path(base path=w1415, name or relative path=w1484) -> (appended path=w1482:path)
        n1106 = Build Path(base path=w1415, name or relative path=w1480) -> (appended path=w1495:path)
        n1107 = local write "Filename"(w1416) -> ()
        n1108 = local write "Lab book file"(w1482) -> ()
        n1109 = call <vilib>:"Check if File or Folder Exists.vi"("path"=w1495) -> ("file or folder exists?"=w1493:bool, "dup path"=w1494:path)  [unwired: 8 in, 1 out]
        n1110 = Format Date/Time String() -> ()  [unwired: 3 in, 1 out]
        n1111 = case shown="False" w1493 {
          tunnel: w1494 -> [w1510 _]
          tunnel: [Record_enum."Record VR" ("Record enum") Record_enum."Init recording" ("Record enum")] -> w1492
          frame False {
            n1112 = TDMS Open(5:FALSE ("create index file? (T)"), 10:T17."create" ("operation (0:open)"), 11:w1510) -> (3:w1507:refnum<k34>)  [unwired: 4 in, 1 out]
            n1113 = local write "My tdms file"(w1507) -> ()
          }
          frame True {
            n1114 = local read "Unique ID"() -> (w1513:i8)
            n1115 = Increment(x=w1513) -> (x+1=w1512:i8)
            n1116 = local write "Unique ID"(w1512) -> ()
          }
        }
      }
      frame "Init data acquisition" {
        w1517 = 0 items=["one channel for each line", "one channel for all lines"] ("line grouping")
        w1523 = 10083 items=["Default"=-1, "RSE"=10083, "NRSE"=10078, "Differential"=10106, "Pseudodifferential"=12529] ("input terminal configuration")
        (unwired) tag "Dev1/ai2" ("physical channels")
        w1531 = 10123 items=["Finite Samples"=10178, "Continuous Samples"=10123, "Hardware Timed Single Point"=12522] ("sample mode")
        w1553 = 10123 items=["Finite Samples"=10178, "Continuous Samples"=10123, "Hardware Timed Single Point"=12522] ("sample mode")
        w1559 = 10123 items=["Finite Samples"=10178, "Continuous Samples"=10123, "Hardware Timed Single Point"=12522] ("sample mode")
        (unwired) tag "Dev1/port0/line6" ("lines")
        # "Photo stim\nPhotodiode\nAnalog lick\nEyecam frame\nML signal\nAnalog 3\nAnalog 5"
        # "Extra Analog Input"
        # "Frame signal 2"
        # "Valve open"
        # "Frame signal"
        # "Encoder"
        # "Lickport"
        n1117 = call "Encoder read task.vi"() -> ("error out"=w1558:errorcluster, "task out"=w1557:refnum<k21>)  [unwired: 10 in]
        n1118 = local read "Sample rate"() -> (w1554:dbl)
        n1119 = call <vilib>:"DAQmx Flatten Channel String.vi"("names in"=string[] ["Dev1/port0/line4", "Dev1/port0/line5", "Dev1/port0/line6", "Dev1/port0/line3"]) -> ("names out"=w1519:string)  [unwired: 13 in, 1 out]
        n1120 = call <vilib>:"DAQmx Flatten Channel String.vi"("names in"=string[] ["Dev1/ai0", "Dev1/ai4", "Dev1/ai6", "Dev1/ai1", "Dev1/ai2", "Dev1/ai3", "Dev1/ai5"]) -> ("names out"=w1529:string)  [unwired: 13 in, 1 out]
        n1121 = local read "Sample rate"() -> (w1561:dbl)
        n1122 = local read "Sample rate"() -> (w1533:dbl)
        n1123 = call-poly <vilib>:"DAQmx Create Virtual Channel.vi"("lines"=w1519, "line grouping"=w1517) -> ("task out"=w1560:refnum<k21>, "error out"=w1562:errorcluster)  [unwired: 12 in]
        n1124 = call-poly <vilib>:"DAQmx Create Virtual Channel.vi"("maximum value"=10.0, "minimum value"=-10.0, "input terminal configuration"=w1523, "physical channels"=w1529) -> ("task out"=w1532:refnum<k21>, "error out"=w1534:errorcluster)  [unwired: 10 in]
        n1125 = call-poly <vilib>:"DAQmx Timing.vi"("task/channels in"=w1557, "sample mode"=w1553, "rate"=w1554, "source"=tag "/Dev1/di/SampleClock", "error in"=w1558) -> ("task out"=w1555:refnum<k21>, "error out"=w1556:errorcluster)  [unwired: 9 in]
        n1126 = call-poly <vilib>:"DAQmx Timing.vi"("task/channels in"=w1560, "sample mode"=w1559, "rate"=w1561, "source"=tag "OnboardClock", "error in"=w1562) -> ("task out"=w1563:refnum<k21>, "error out"=w1564:errorcluster)  [unwired: 9 in]
        n1127 = call-poly <vilib>:"DAQmx Timing.vi"("task/channels in"=w1532, "sample mode"=w1531, "rate"=w1533, "source"=tag "/Dev1/di/SampleClock", "error in"=w1534) -> ("task out"=w1535:refnum<k21>, "error out"=w1536:errorcluster)  [unwired: 9 in]
        n1128 = call <vilib>:"DAQmx Start Task.vi"("task/channels in"=w1555, "error in"=w1556) -> ("task out"=w1551:refnum<k21>, "error out"=w1550:errorcluster)  [unwired: 12 in]
        n1129 = call <vilib>:"DAQmx Start Task.vi"("task/channels in"=w1563, "error in"=w1564) -> ("task out"=w1549:refnum<k21>, "error out"=w1548:errorcluster)  [unwired: 12 in]
        n1130 = call <vilib>:"DAQmx Start Task.vi"("task/channels in"=w1535, "error in"=w1536) -> ("task out"=w1527:refnum<k21>, "error out"=w1526:errorcluster)  [unwired: 12 in]
        n1131 = local write "prev. diode position"(-157.0 ("prev. diode position")) -> ()
        n1132 = local write "Store prev encoder count"(w1537) -> ()
        n1133 = local read "Record"() -> (w1545:bool)
        n1134 = Tick Count (ms)() -> (millisecond timer value=w1547:u32)
        "Start time" <- w1547
        n1135 = local write "index"(0 ("index")) -> ()
        n1136 = Select(t=Record_enum."Init recording" ("Record enum"), s=w1545, f=Record_enum."Record VR" ("Record enum")) -> (s? t:f=w1542:T7)
      }
      frame "Idle" {
        n1137 = local write "Record loop state"(w1579) -> ()
        n1138 = Wait (ms)(milliseconds to wait=u32 20) -> ()  [unwired: 1 out]
        n1139 = local read "Run experiment"() -> (w1583:bool)
        n1140 = Select(t=Record_enum."Init data acquisition" ("Record enum"), s=w1583, f=Record_enum."Idle" ("Record enum")) -> (s? t:f=w1580:T7)
        n1141 = local read "Exit"() -> (w1578:bool)
      }
      frame "Stop data acquision" {
        n1142 = local write "Record loop state"(w1610) -> ()
        n1143 = local read "Record"() -> (w1597:bool)
        n1144 = call <vilib>:"DAQmx Stop Task.vi"("task/channels in"=w1605, "error in"=w1604) -> ("task out"=w1600:refnum<k21>, "error out"=w1606:errorcluster)  [unwired: 12 in]
        n1145 = call <vilib>:"DAQmx Stop Task.vi"("task/channels in"=w1592, "error in"=w1591) -> ("task out"=w1590:refnum<k21>, "error out"=w1593:errorcluster)  [unwired: 12 in]
        n1146 = call <vilib>:"DAQmx Stop Task.vi"("task/channels in"=w1602, "error in"=w1603) -> ("task out"=w1601:refnum<k21>, "error out"=w1588:errorcluster)  [unwired: 12 in]
        n1147 = call <vilib>:"DAQmx Clear Task.vi"("task in"=w1600, "error in"=w1606) -> ("error out"=w1598:errorcluster)  [unwired: 13 in]
        n1148 = call <vilib>:"DAQmx Clear Task.vi"("task in"=w1590, "error in"=w1593) -> ("error out"=w1589:errorcluster)  [unwired: 13 in]
        n1149 = call <vilib>:"DAQmx Clear Task.vi"("task in"=w1601, "error in"=w1588) -> ("error out"=w1599:errorcluster)  [unwired: 13 in]
        n1150 = case shown="True" w1597 {
          frame False {
            n1151 = local write "Start recording"(FALSE ("Start recording")) -> ()
          }
          frame True {
            w1628 = "\n"
            w1616 = "\n******************************\n" ("string")
            # "Write labbook data"
            n1152 = local read "VR Mode"() -> (w1626:bool)
            n1153 = local write "VR Mode"(w1626) -> ()
            n1154 = local read "My tdms file"() -> (w1667:refnum<k34>)
            n1155 = case shown="True" TRUE {
              tunnel: [w1695 w1737] -> w1635
              frame True {
                w1672 = "\n" ("string")
                w1686 = "\n" ("string")
                w1698 = " (" ("string")
                # "VR Variables"
                n1156 = local read "Trials in session array"() -> (w1685:u16[][])
                n1157 = local read "Stim types"() -> (w1675:u16[])
                n1158 = Number To Decimal String(number=w1685) -> (decimal integer string=w1684:string[][])  [unwired: 1 in]
                n1159 = Add Array Elements(numeric array=w1675) -> (sum=w1677:u16)
                n1160 = Greater?(x=w1677, y=i16 0) -> (0:w1674:bool)
                n1161 = Index Array(array=w1684, index (col)=0 ("disabled index (col)")) -> (element=w1683:string[])  [unwired: 1 in]
                n1162 = Index Array(array=w1684, index (col)=1 ("disabled index (col)")) -> (element=w1682:string[])  [unwired: 1 in]
                n1163 = case shown="True" w1674 {
                  tunnel: ["" ("Laser stimulus calibration") w1711] -> w1671
                  frame False {
                  }
                  frame True {
                    n1164 = local read "Laser stimulus calibration"() -> (w1712:string)
                    n1165 = Concatenate Strings("\n" ("string"), w1712) -> (w1711:string)
                  }
                }
                n1166 = local read "Stimulus protocol"() -> (w1673:string)
                n1167 = Concatenate Strings("Trial types (stimulus protocols):\n", w1683, "\nTrial types (VR contexts):\n", w1682) -> (w1670:string)
                n1168 = local read "Masking light prot"() -> (w1694:string)
                n1169 = Concatenate Strings(w1673, w1672, w1670, w1672) -> (w1669:string)
                n1170 = Concatenate Strings(w1686, w1694, w1686, w1669, w1671) -> (w1693:string)
                n1171 = local read "Control hit trials %"() -> (w1688:dbl)
                n1172 = local read "Stim. hit trials %"() -> (w1687:dbl)
                n1173 = local read "Ctrl. count"() -> (w1704:i32)
                n1174 = local read "Stim. count"() -> (w1689:i32)
                n1175 = local read "All trials"() -> (w1707:i32)
                n1176 = Number To Decimal String(number=w1704) -> (decimal integer string=w1703:string)  [unwired: 1 in]
                n1177 = Number To Decimal String(number=w1707) -> (decimal integer string=w1706:string)  [unwired: 1 in]
                n1178 = Number To Fractional String(number=w1687, precision (6)=i16 2) -> (F-format string=w1697:string)  [unwired: 2 in]
                n1179 = Number To Decimal String(number=w1689) -> (decimal integer string=w1699:string)  [unwired: 1 in]
                n1180 = Number To Fractional String(number=w1688, precision (6)=i16 2) -> (F-format string=w1701:string)  [unwired: 2 in]
                n1181 = Concatenate Strings("\nReward zone distance: " ("string"), "" ("string"), " cm " ("string"), "\nAll trials: " ("string"), w1706, "\nControl trials: " ("string"), w1703, w1698, w1701, " % hit)\nStimulated trials: " ("string"), w1699, w1698, w1697, " % hit)\n" ("string"), w1693) -> (w1695:string)
              }
              frame False {
                w1713 = "\n" ("string")
                n1182 = local read "Stim types"() -> (w1717:u16[])
                n1183 = Add Array Elements(numeric array=w1717) -> (sum=w1720:u16)
                n1184 = Greater?(x=w1720, y=i16 0) -> (0:w1719:bool)
                n1185 = case shown="True" w1719 {
                  tunnel: ["" ("Laser stimulus calibration") w1740] -> w1714
                  frame False {
                  }
                  frame True {
                    w1739 = "\n" ("string")
                    n1186 = local read "Stimulus protocol"() -> (w1742:string)
                    n1187 = local read "Laser stimulus calibration"() -> (w1741:string)
                    n1188 = Concatenate Strings(w1742, w1739, w1741, w1739) -> (w1740:string)
                  }
                }
                n1189 = local read "Reward zone"() -> (w1721:bool)
                n1190 = local read "Masking light prot"() -> (w1718:string)
                n1191 = case shown="True" w1721 {
                  tunnel: [w1744 w1747] -> w1722
                  frame True {
                    n1192 = local read "VR Mode"() -> (w1743:bool)
                    n1193 = case shown="False" w1743 {
                      tunnel: ["Reward zone starts at photo diode (0-6 cm)." ""] -> w1744
                      frame False {
                      }
                      frame True {
                      }
                    }
                  }
                  frame False {
                    n1194 = local read "Reward freq. (cm)"() -> (w1750:u32)
                    n1195 = Number To Fractional String(number=w1750, precision (6)=i16 0) -> (F-format string=w1748:string)  [unwired: 2 in]
                    n1196 = Concatenate Strings("\nReward frequency (minimum): " ("string"), w1748) -> (w1747:string)
                  }
                }
                n1197 = Concatenate Strings(w1713, w1718, w1713, w1714) -> (w1715:string)
                n1198 = local read "Hit trials"() -> (w1732:i32)
                n1199 = local read "All trials"() -> (w1731:i32)
                n1200 = Divide(x=w1732, y=w1731) -> (x/y=w1730:dbl)
                n1201 = Number To Decimal String(number=w1731) -> (decimal integer string=w1735:string)  [unwired: 1 in]
                n1202 = Multiply(x=w1730, y=100.0) -> (x*y=w1727:dbl)
                n1203 = Number To Decimal String(number=w1732) -> (decimal integer string=w1733:string)  [unwired: 1 in]
                n1204 = Number To Fractional String(number=w1727, precision (6)=i16 2) -> (F-format string=w1725:string)  [unwired: 2 in]
                n1205 = Concatenate Strings(w1722, "\nAll trials: " ("string"), w1735, "\nHit trials: " ("string"), w1733, " (" ("string"), w1725, " % correct)" ("string")) -> (w1723:string)
                n1206 = Concatenate Strings(w1723, w1715) -> (w1737:string)
              }
            }
            n1207 = local write "Record Button"(FALSE ("Record Button")) -> ()
            n1208 = local read "Security camera"() -> (w1630:string)
            n1209 = local write "Record"(FALSE ("Logg data")) -> ()
            n1210 = local read "2P imaging"() -> (w1629:string)
            n1211 = local read "Reward size (ul)"() -> (w1656:dbl)
            n1212 = TDMS Close(11:w1667) -> ()  [unwired: 1 in, 2 out]
            n1213 = local read "Water count"() -> (w1655:i32)
            n1214 = Concatenate Strings(w1628, w1630, w1628, w1629, w1628) -> (w1627:string)
            n1215 = Multiply(x=w1656, y=w1655) -> (x*y=w1654:dbl)
            n1216 = Number To Fractional String(number=w1654, precision (6)=i16 2) -> (F-format string=w1651:string)  [unwired: 2 in]
            n1217 = Concatenate Strings("\nWater received: " ("string"), w1651, " ul" ("string")) -> (w1636:string)
            n1218 = Format Date/Time String(time format string (%c)="Session stop: %H:%M:%S\n") -> (date/time string=w1631:string)  [unwired: 2 in]
            n1219 = local read "Distance (m)"() -> (w1642:dbl)
            n1220 = local read "Session start:"() -> (w1632:string)
            n1221 = local read "Time (min)"() -> (w1646:dbl)
            n1222 = local read "Lab book notes"() -> (w1663:string)
            n1223 = Number To Fractional String(number=w1646, precision (6)=i16 2) -> (F-format string=w1647:string)  [unwired: 2 in]
            n1224 = local read "Laps"() -> (w1638:i32)
            n1225 = Number To Fractional String(number=w1642, precision (6)=i16 2) -> (F-format string=w1641:string)  [unwired: 2 in]
            n1226 = Number To Decimal String(number=w1638) -> (decimal integer string=w1637:string)  [unwired: 1 in]
            n1227 = Match Pattern(string=w1663, regular expression="**********\n") -> (after substring=w1614:string)  [unwired: 1 in, 3 out]
            n1228 = Concatenate Strings(w1632, w1631, "Time: " ("string"), w1647, " minutes\n" ("string"), "Distance: " ("string"), w1641, " m\n" ("string"), "Laps completed: " ("string"), w1637, w1636, w1635, w1627, w1616) -> (w1634:string)
            n1229 = local read "Default vars text"() -> (w1622:string)
            n1230 = local read "Task config"() -> (w1621:string)
            n1231 = local read "Saved signals"() -> (w1623:string)
            n1232 = local read "Lab book file"() -> (w1661:path)
            n1233 = local read "Header"() -> (w1664:string)
            n1234 = Concatenate Strings(w1616, "VR context configuration. (Name, Corridor length, Teleport point, Reward zone starts and ends.):\n\n" ("string"), w1621, w1616, "Default variables of user configuration: \n\n" ("string"), w1622, w1616, "Signals saved:\n\n" ("string"), w1623) -> (w1617:string)
            n1235 = Concatenate Strings(w1614, "\n" ("string")) -> (w1613:string)
            n1236 = Open/Create/Replace File(file path (use dialog)=w1661, operation (0:open)=T9."create") -> (refnum out=w1662:refnum<file>)  [unwired: 4 in, 2 out]
            n1237 = Concatenate Strings(w1664, w1634, "Notes:\n\n" ("string"), w1613, w1617) -> (w1665:string)
            n1238 = Write to Text File(file (use dialog)=w1662, text=w1665) -> (refnum out=w1660:refnum<file>)  [unwired: 2 in, 2 out]
            n1239 = Close File(refnum=w1660) -> ()  [unwired: 1 in, 2 out]
          }
        }
      }
      frame "Record VR" {
        # "Calculate Velocity (cm/s) with 50Hz sampling"
        n1240 = local read "VR Mode"() -> (w1776:bool)
        n1241 = local read "Record"() -> (w1842:bool)
        n1242 = case shown="False" w1842 {
          frame False {
            # "Stim prot"
            # "VR ctx"
            n1243 = local read "No. of smpl. per ch."() -> (w1898:i32)
            n1244 = local read "VR Gain"() -> (w1900:dbl)
            n1245 = local read "Photodiode signal"() -> (w1920:sgl[])
            n1246 = local read "total distance cm"() -> (w1919:sgl[])
            n1247 = local read "Track position"() -> (w1913:sgl)
            n1248 = local read "Valve signal"() -> (w1910:i8[])
            n1249 = local read "lick signal"() -> (w1908:i8[])
            n1250 = local read "analog lick"() -> (w1909:sgl[])
            n1251 = local read "Trials in session array"() -> (w1916:u16[][])
            n1252 = local read "All trials"() -> (w1912:i32)
            n1253 = local read "Eye cam frame signal"() -> (w1915:i8[])
            n1254 = local read "Analog 3"() -> (w1906:sgl[])
            n1255 = local read "Photo stimulus signal"() -> (w1905:sgl[])
            n1256 = local read "ML signal"() -> (w1904:sgl[])
            n1257 = local read "Frame signal"() -> (w1901:i8[])
            n1258 = local read "Frame signal 2"() -> (w1902:i8[])
            n1259 = local read "Encoder signal"() -> (w1918:sgl[])
            n1260 = local read "Analog 5"() -> (w1895:sgl[])
            n1261 = Index Array(array=w1916, index (row)=w1912, index (col)=0 ("disabled index (col)")) -> (element=w1914:u16)
            n1262 = Index Array(array=w1916, index (row)=w1912, index (col)=1 ("disabled index (col)")) -> (element=w1917:u16)
            n1263 = Initialize Array(w1900, w1898) -> (w1899:dbl[])
            n1264 = Initialize Array(w1914, w1898) -> (w1903:u16[])
            n1265 = Initialize Array(w1917, w1898) -> (w1907:u16[])
            n1266 = Initialize Array(w1913, w1898) -> (w1911:sgl[])
            n1267 = Build Array(w1918, w1920, w1919, w1911, w1910, w1908, w1909, w1907, w1899, w1901, w1902, w1915, w1906, w1905, w1904, w1903, w1895) -> (w1888:dbl[][])
            n1268 = Index Array(array=w1888, index (row)="Ring") -> (element=→"Waveform Chart":dbl[])  [unwired: 1 in]
            n1269 = Index Array(array=w1888, index (row)="Ring 2") -> (element=→"Waveform Chart 2":dbl[])  [unwired: 1 in]
            n1270 = Index Array(array=w1888, index (row)="Ring 3") -> (element=→"Waveform Chart 3":dbl[])  [unwired: 1 in]
            n1271 = Index Array(array=w1888, index (row)="Ring 4") -> (element=→"Waveform Chart 4":dbl[])  [unwired: 1 in]
          }
          frame True {
            n1272 = case shown="True" TRUE ("VR Mode") {
              frame True {
                # "Stim prot"
                # "VR ctx"
                n1273 = local read "No. of smpl. per ch."() -> (w1927:i32)
                n1274 = local read "VR Gain"() -> (w1929:dbl)
                n1275 = local read "Photodiode signal"() -> (w1951:sgl[])
                n1276 = local read "total distance cm"() -> (w1950:sgl[])
                n1277 = local read "Track position"() -> (w1943:sgl)
                n1278 = local read "Valve signal"() -> (w1940:i8[])
                n1279 = local read "lick signal"() -> (w1938:i8[])
                n1280 = local read "analog lick"() -> (w1939:sgl[])
                n1281 = local read "Trials in session array"() -> (w1947:u16[][])
                n1282 = local read "All trials"() -> (w1942:i32)
                n1283 = local read "Eye cam frame signal"() -> (w1945:i8[])
                n1284 = local read "Analog 3"() -> (w1936:sgl[])
                n1285 = local read "Photo stimulus signal"() -> (w1935:sgl[])
                n1286 = local read "ML signal"() -> (w1934:sgl[])
                n1287 = local read "Frame signal"() -> (w1931:i8[])
                n1288 = local read "Frame signal 2"() -> (w1932:i8[])
                n1289 = local read "Encoder signal"() -> (w1949:sgl[])
                n1290 = local read "Analog 5"() -> (w1930:sgl[])
                n1291 = Index Array(array=w1947, index (row)=w1942, index (col)=0 ("disabled index (col)")) -> (element=w1944:u16)
                n1292 = Index Array(array=w1947, index (row)=w1942, index (col)=1 ("disabled index (col)")) -> (element=w1948:u16)
                n1293 = Initialize Array(w1929, w1927) -> (w1928:dbl[])
                n1294 = Initialize Array(w1944, w1927) -> (w1933:u16[])
                n1295 = Initialize Array(w1948, w1927) -> (w1937:u16[])
                n1296 = Initialize Array(w1943, w1927) -> (w1941:sgl[])
                n1297 = Build Array(w1949, w1951, w1950, w1941, w1940, w1938, w1939, w1937, w1928, w1931, w1932, w1945, w1936, w1935, w1934, w1933, w1930) -> (w1925:dbl[][])
                n1298 = case shown="True" TRUE {
                  tunnel: w1925 -> [w1955 w1957]
                  tunnel: [w1955 w1956] -> w1924
                  frame False {
                  }
                  frame True {
                    n1299 = local read "Signals to delete"() -> (w1958:i32[])
                    n1300 = for {
                      tunnel: w1958 -> [w1962] mode=indexing
                      shift-right: [w1959] -> w1956
                      shift-left: w1957 -> [w1961]
                      n1301 = Delete From Array(array=w1961, length=1, index (row)=w1962) -> (array with subset deleted=w1959:dbl[][])  [unwired: 1 in, 1 out]
                    }
                  }
                }
                n1302 = local read "channel names"() -> (w1926:string[])
                n1303 = local read "My tdms file"() -> (w1953:refnum<k34>)
                n1304 = TDMS Write(0:w1953, 1:enum16{"decimated", "interleaved"}."decimated" ("data layout (0:decimated)"), 7:w1926, 9:w1924) -> ()  [unwired: 2 in, 4 out]
              }
              frame False {
                n1305 = local read "Trials in session array"() -> (w1978:u16[][])
                n1306 = local read "Encoder signal"() -> (w1965:sgl[])
                n1307 = local read "Photodiode signal"() -> (w1976:sgl[])
                n1308 = local read "total distance cm"() -> (w1974:sgl[])
                n1309 = local read "Photo stimulus signal"() -> (w1973:sgl[])
                n1310 = local read "Valve signal"() -> (w1970:i8[])
                n1311 = local read "lick signal"() -> (w1969:i8[])
                n1312 = local read "Frame signal"() -> (w1968:i8[])
                n1313 = local read "All trials"() -> (w1964:i32)
                n1314 = local read "No. of smpl. per ch."() -> (w1975:i32)
                n1315 = local read "Eye cam frame signal"() -> (w1963:i8[])
                n1316 = Index Array(array=w1978, index (row)=w1964, index (col)=0 ("disabled index (col)")) -> (element=w1966:u16)
                n1317 = Initialize Array(w1966, w1975) -> (w1967:u16[])
                n1318 = Build Array(w1965, w1976, w1974, w1973, w1970, w1969, w1968, w1967, w1963) -> (w1971:sgl[][])
                n1319 = local read "My tdms file"() -> (w1979:refnum<k34>)
                n1320 = TDMS Write(0:w1979, 1:enum16{"decimated", "interleaved"}."decimated" ("data layout (0:decimated)"), 7:string[] ["Encoder signal", "Photo-diode", "Distance (cm)", "Photo stimulus signal", "Valve open", "Lick signal", "Frame signal", "Stimulus protocol", "EyeCam frame signal"] ("channel name(s) in (Untitled)"), 9:w1971) -> ()  [unwired: 2 in, 4 out]
              }
            }
            n1321 = local read "VR Mode"() -> (w1921:bool)
            n1322 = local write "VR Mode"(w1921) -> ()
          }
        }
        n1323 = case shown="False" w1776 {
          frame True {
          }
          frame False {
            n1324 = local read "prev. diode position"() -> (w1875:dbl)
            n1325 = local read "Distance (cm)"() -> (w1876:dbl)
            n1326 = Subtract(x=w1876, y=w1875) -> (x-y=w1874:dbl)
            n1327 = local write "Track position"(w1874) -> ()
          }
        }
        n1328 = local read "index"() -> (w1832:i32)
        n1329 = Increment(x=w1832) -> (x+1=w1834:i32)
        n1330 = local read "delta distance cm"() -> (w1814:dbl[])
        n1331 = local read "No. of smpl. per ch."() -> (w1861:i32)
        n1332 = local write "index"(w1834) -> ()
        n1333 = local read "Loop rate"() -> (w1820:dbl)
        n1334 = local read "No. of smpl. per ch."() -> (w1807:i32)
        n1335 = local read "delta time (s)"() -> (w1824:dbl)
        n1336 = local read "No. of smpl. per ch."() -> (w1845:i32)
        n1337 = local read "encoder ticks per rev"() -> (w1783:dbl)
        n1338 = Add Array Elements(numeric array=w1814) -> (sum=w1817:dbl)
        n1339 = Array Size(array=w1814) -> (size(s)=w1816:i32)
        n1340 = local read "Store prev encoder count"() -> (w1810:dbl)
        n1341 = local read "Start time"() -> (w1841:u32)
        n1342 = call-poly <vilib>:"DAQmx Read.vi"("task/channels in"=w1858, "number of samples per channel"=w1861, "error in"=w1857) -> ("task out"=w1851:refnum<k21>, "data"=w1848:dbl[], "error out"=w1850:errorcluster)  [unwired: 10 in]
        n1343 = local read "Wheel circumference"() -> (w1865:dbl)
        n1344 = Divide(x=w1817, y=w1816) -> (x/y=w1815:dbl)
        n1345 = Divide(x=w1820, y=50.0) -> (x/y=w1818:dbl)
        n1346 = Add(x=w1829, y=w1815) -> (x+y=w1823:dbl)
        n1347 = Add(x=w1825, y=w1824) -> (x+y=w1822:dbl)
        n1348 = Subtract(x=w1848, y=40000.0) -> (x-y=w1779:dbl[])
        "Encoder signal" <- w1779
        n1349 = call-poly <vilib>:"DAQmx Read.vi"("task/channels in"=w1803, "number of samples per channel"=w1807, "error in"=w1806) -> ("task out"=w1800:refnum<k21>, "data"=w1752:dbl[][], "error out"=w1805:errorcluster)  [unwired: 10 in]
        n1350 = Index Array(array=w1752, index (row)=2 ("index")) -> (element=→"analog lick":dbl[])  [unwired: 1 in]
        n1351 = Index Array(array=w1752, index (row)=4 ("index")) -> (element=→"ML signal":dbl[])  [unwired: 1 in]
        n1352 = Index Array(array=w1752, index (row)=5 ("index")) -> (element=→"Analog 3":dbl[])  [unwired: 1 in]
        n1353 = Index Array(array=w1752, index (row)=6 ("index")) -> (element=→"Analog 5":dbl[])  [unwired: 1 in]
        n1354 = call-poly <vilib>:"DAQmx Read.vi"("task/channels in"=w1853, "number of samples per channel"=w1845, "error in"=w1852) -> ("task out"=w1844:refnum<k21>, "data"=w1760:u8[][], "error out"=w1843:errorcluster)  [unwired: 10 in]
        n1355 = local read "index"() -> (w1833:i32)
        n1356 = Tick Count (ms)() -> (millisecond timer value=w1847:u32)
        n1357 = Index Array(array=w1779, index=0) -> (element=w1809:dbl)
        n1358 = Subtract(x=w1847, y=w1841) -> (x-y=w1804:u32)
        "Experiment time (ms)" <- w1804
        n1359 = Divide(x=w1779, y=w1783) -> (x/y=w1867:dbl[])
        n1360 = Greater Or Equal?(x=w1833, y=w1818) -> (x >= y?=w1821:bool)
        n1361 = Add(x=w1810, y=w1809) -> (x+y=w1808:dbl)
        "Encoder count" <- w1808
        n1362 = Multiply(x=w1867, y=w1865) -> (x*y=w1782:dbl[])
        "total distance cm" <- w1782
        n1363 = Index Array(array=w1752, index (row)=0 ("index")) -> (element=w1764:dbl[])  [unwired: 1 in]
        "Opt stim command" <- w1764
        n1364 = Index Array(array=w1752, index (row)=1 ("index")) -> (element=w1758:dbl[])  [unwired: 1 in]
        "Photodiode signal" <- w1758
        n1365 = Index Array(array=w1752, index (row)=3 ("index")) -> (element=w1769:dbl[])  [unwired: 1 in]
        n1366 = Index Array(array=w1760, index (row)=3) -> (element=w1759:u8[])  [unwired: 1 in]
        n1367 = Index Array(array=w1760, index (row)=1) -> (element=w1856:u8[])  [unwired: 1 in]
        n1368 = Index Array(array=w1760, index (row)=0) -> (element=w1794:u8[])  [unwired: 1 in]
        n1369 = Subtract(x=w1804, y=w1840) -> (x-y=w1827:u32)
        "Recording loop rate  (ms)" <- w1827
        n1370 = case shown="True" w1821 {
          tunnel: [w1878 0.0] -> w1830
          tunnel: [w1879 0.0] -> w1831
          tunnel: w1823 -> [w1879 w1883]
          tunnel: w1822 -> [w1878 w1882]
          frame False {
          }
          frame True {
            n1371 = Divide(x=w1883, y=w1882) -> (x/y=w1880:dbl)
            "Velocity chart" <- w1880
            n1372 = local write "index"(0 ("index")) -> ()
            n1373 = local write "velocity (cm/s)"(w1880) -> ()
          }
        }
        n1374 = local write "Photo stimulus signal"(w1764) -> ()
        n1375 = Index Array(array=w1782, index=0) -> (element=w1862:dbl)
        n1376 = Divide(x=w1856, y=32.0) -> (x/y=w1785:dbl[])
        "lick signal" <- w1785
        n1377 = Divide(x=w1759, y=8.0) -> (x/y=→"Frame signal 2":dbl[])
        n1378 = Divide(x=w1794, y=16.0) -> (x/y=→"Frame signal":dbl[])
        n1379 = Array Max & Min(array=w1758) -> (max value=w1757:dbl)  [unwired: 3 out]
        n1380 = Divide(x=w1769, y=3.3) -> (x/y=w1770:dbl[])
        n1381 = Quotient & Remainder(x=w1862, y=w1865) -> (x-y*floor(x/y)=→"Position on the wheel":dbl, floor(x/y)=→"Laps":dbl)
        n1382 = Round To Nearest(number=w1770) -> (nearest integer value=→"Eye cam frame signal":dbl[])
        n1383 = Divide(x=w1804, y=1000.0) -> (x/y=w1812:dbl)
        n1384 = Divide(x=w1827, y=1000.0) -> (x/y=→"delta time (s)":dbl)
        n1385 = local read "Valve open"() -> (w1838:bool)
        n1386 = disable-structure shown="Disabled" {
          disable-tunnel: w1812 -> [w1873 _]
          frame Disabled {
            "Experiment time (s)" <- w1873
          }
          frame Enabled {
          }
        }
        n1387 = Greater?(x=w1757, y=1.5) -> (0:w1792:bool)
        "Photodiode" <- w1792
        n1388 = Add Array Elements(numeric array=w1785) -> (sum=w1787:dbl)
        n1389 = Array Size(array=w1785) -> (size(s)=w1786:i32)
        n1390 = Index Array(array=w1785, index=0) -> (element=w1835:dbl)
        n1391 = Array Max & Min(array=w1782) -> (max value=w1781:dbl)  [unwired: 3 out]
        "Distance (cm)" <- w1781
        n1392 = Index Array(array=w1760, index (row)=2) -> (element=w1791:u8[])  [unwired: 1 in]
        n1393 = Subtract(x=w1782, y=w1793) -> (x-y=→"delta distance cm":dbl[])
        n1394 = Divide(x=w1787, y=w1786) -> (x/y=w1784:dbl)
        n1395 = Boolean To (0,1)(Boolean=w1838) -> (0, 1=w1836:i16)
        n1396 = Array Max & Min(array=w1764) -> (max value=w1775:dbl)  [unwired: 3 out]
        n1397 = case shown="True" w1792 {
          tunnel: w1781 -> [_ w1877]
          frame False {
          }
          frame True {
            n1398 = local write "prev. diode position"(w1877) -> ()
          }
        }
        n1399 = local read "Run experiment"() -> (w1872:bool)
        n1400 = Divide(x=w1781, y=100.0) -> (x/y=→"Distance (m)":dbl)
        n1401 = Divide(x=w1791, y=64.0) -> (x/y=→"Valve signal":dbl[])
        n1402 = Divide(x=w1812, y=60.0) -> (x/y=→"Time (min)":dbl)
        n1403 = Bundle(w1835, w1836) -> (→"Lick and reward chart":cluster{dbl, i16})  [unwired: 1 in]
        n1404 = local write "Lick indicator"(w1784) -> ()
        n1405 = Greater?(x=w1775, y=0.5) -> (0:w1773:bool)
        n1406 = local write "Laser ON"(w1773) -> ()
        n1407 = Select(t=Record_enum."Record VR" ("Record enum"), s=w1872, f=Record_enum."Stop data acquision" ("Record enum")) -> (s? t:f=w1870:T7)
        "Record loop state" <- w1869
      }
      frame "Record" {
        n1408 = local write "Record loop state"(w1995) -> ()
        n1409 = local read "Run experiment"() -> (w1998:bool)
        n1410 = Select(t=Record_enum."Record" ("Record enum"), s=w1998, f=Record_enum."Stop data acquision" ("Record enum")) -> (s? t:f=w1996:T7)
      }
    }
    n1411 = local write "Exit program"("Exit program") -> ()
  }
  n1412 = while {
    shift-right: [w2013] -> _
    shift-left: T6."Idle" ("Eyecam states") -> [w2015]
    shift-right: [w2012] -> _
    shift-left: _ -> [w2006]
    shift-right: [w2011] -> _
    shift-left: _ -> [w2005]
    shift-right: [w2010] -> _
    shift-left: _ -> [w2004]
    shift-right: [w2009] -> _
    shift-left: _ -> [w2003]
    shift-right: [w2008] -> _
    shift-left: _ -> [w2002]
    shift-right: [w2007] -> _
    shift-left: _ -> [w2001]
    shift-right: [w2000] -> _
    shift-left: _ -> [w1999]
    stop <- w2014 stop-if-true
    n1413 = case shown="\"Idle\", Default" w2015 {
      tunnel: [w2031 w2070 T6."Record pupille" ("Eyecam states") w2172 T6."Idle" ("Eyecam states")] -> w2013
      tunnel: [w2025 FALSE FALSE ("Exit") FALSE ("Exit") FALSE ("Exit")] -> w2014
      tunnel: [w2018 w2053 w2105 w2140 w2201] -> w2012
      tunnel: [w2019 w2048 w2104 w2142 w2200] -> w2011
      tunnel: [w2020 w2049 w2103 w2144 w2199] -> w2010
      tunnel: [w2021 w2052 w2102 w2146 w2198] -> w2009
      tunnel: [w2022 w2051 w2101 w2148 w2197] -> w2008
      tunnel: [w2023 w2050 w2100 w2151 w2196] -> w2007
      tunnel: w2006 -> [w2018 _ w2105 w2140 w2201]
      tunnel: w2005 -> [w2019 _ w2104 w2142 w2200]
      tunnel: w2004 -> [w2020 _ w2103 w2144 w2199]
      tunnel: w2003 -> [w2021 _ w2102 w2146 w2198]
      tunnel: w2002 -> [w2022 _ w2101 w2148 w2197]
      tunnel: w2001 -> [w2023 _ w2100 w2151 w2196]
      tunnel: [0 w2046 0 w2139 0] -> w2000
      tunnel: w1999 -> [_ w2045 _ w2138 _]
      frame "Idle", Default {
        n1414 = local write "Pupille image"(T3 refnum ("Security cam image")) -> ()
        n1415 = local read "Record Button 2"() -> (w2016:bool)
        n1416 = Wait (ms)(milliseconds to wait=u32 10) -> ()  [unwired: 1 out]
        n1417 = case shown="False" w2016 {
          frame False {
          }
          frame True {
            n1418 = Get Volume Info(11:path "C:/" ("path")) -> (1:w2038:i64)  [unwired: 1 in, 5 out]
            n1419 = Divide(x=w2038, y=i64 1024) -> (x/y=w2042:dbl)
            n1420 = Divide(x=w2042, y=i64 1024) -> (x/y=w2043:dbl)
            n1421 = Divide(x=w2043, y=i64 1024) -> (x/y=w2034:dbl)
            n1422 = Number To Fractional String(number=w2034, precision (6)=i16 1) -> (F-format string=w2035:string)  [unwired: 2 in]
            n1423 = Concatenate Strings("Pupil wideo will be recorded! \nAvailable disk space: " ("string"), w2035, " GB" ("string")) -> (w2032:string)
            n1424 = One Button Dialog(message=w2032) -> ()  [unwired: 1 in, 1 out]
          }
        }
        n1425 = local read "Eable eye cam"() -> (w2030:bool)
        n1426 = And(x=w2016, y=w2030) -> (x .and. y?=w2029:bool)
        n1427 = local read "Exit"() -> (w2025:bool)
        n1428 = Select(t=T6."Set params" ("Eyecam states"), s=w2029, f=T6."Idle" ("Eyecam states")) -> (s? t:f=w2031:T6)
      }
      frame "Set params" {
        n1429 = case shown="2.." w2045 {
          tunnel: [i64 100 ("Image Format Control::Offset Y") i64 102 ("Image Format Control::Offset Y") "Image Format Control::Offset Y"] -> w2050
          tunnel: [i64 100 ("Image Format Control::Offset X") i64 102 ("Image Format Control::Offset X") "Image Format Control::Offset X"] -> w2051
          tunnel: [29.0 ("Target frame rate") 28.0 ("Target frame rate") "Target frame rate"] -> w2052
          tunnel: [10.0 ("Gain") 9.0 ("Gain") "Gain"] -> w2049
          tunnel: [0.0 ("Black Level") 1.0 ("Black Level") "Black Level"] -> w2048
          tunnel: [5.0 5.5 "Exposure Time (ms)"] -> w2047
          selector: w2045 -> [_ _ w2096]
          tunnel: [1 2 w2096] -> w2046
          frame ..0 {
          }
          frame 1 {
          }
          frame 2.. {
          }
        }
        n1430 = Divide(x=1000, y=w2052) -> (x/y=w2060:dbl)
        n1431 = Multiply(x=0.9, y=w2060) -> (x*y=w2058:dbl)
        n1432 = call "Is Value Changed.vim"("value"=w2052) -> ("changed or first call?"=w2056:bool)
        n1433 = case shown="True" w2056 {
          tunnel: w2058 -> [_ w2098]
          frame False {
          }
          frame True {
            n1434 = To Quad Integer(1:w2098) -> (0:w2097:i64)
            n1435 = property on="Exposure Time (ms)" class="Slide (strict)"("Maximum"=w2097, "Scale.Maximum"=w2097, "Value"=w2097) -> ()  [unwired: 2 in, 2 out]
          }
        }
        n1436 = local read "Run experiment"() -> (w2065:bool)
        n1437 = local read "Record Button 2"() -> (w2072:bool)
        n1438 = Multiply(x=1000.0, y=w2047) -> (x*y=w2053:dbl)
        n1439 = local read "Exit"() -> (w2068:bool)
        n1440 = Not(x=w2072) -> (.not. x?=w2067:bool)
        n1441 = Compound Arithmetic op=OR(w2065, w2067, w2068) -> (w2069:bool)
        n1442 = call "Vision Acquisition"("Analog Control::Gain"=w2049, "Analog Control::Black Level"=w2048, "Acquisition Control::Exposure Time"=w2053, "Acquisition Control::Acquisition Frame Rate"=w2052, "Image Format Control::Offset X"=w2051, "Stop (F)"=w2069, "Image Format Control::Offset Y"=w2050) -> ("Image Out"=w2074:T3, "Lost Image Count"=→"Lost Image Count":u32, "Total Images Transferred"=→"Total Images Transferred":u32, "Frame Rate"=→"Frame rate":dbl, "Stopped"=w2073:bool)  [unwired: 13 in, 3 out]
        n1443 = local write "Pupille image"(w2074) -> ()
        n1444 = Select(t=T6."Start recording" ("Eyecam states"), s=w2065, f=T6."Idle" ("Eyecam states")) -> (s? t:f=w2064:T6)
        n1445 = Select(t=w2064, s=w2073, f=T6."Set params" ("Eyecam states")) -> (s? t:f=w2070:T6)
      }
      frame "Start recording" {
        # "Wait to make sure DAQ recording \nis started before saving images"
        n1446 = disable-structure shown="Disabled" {
          frame Disabled {
            n1447 = local read "Record"() -> (w2117:bool)
            n1448 = case shown="True" w2117 {
              frame False {
              }
              frame True {
                n1449 = Get Volume Info(11:path "C:/" ("path")) -> (1:w2124:i64)  [unwired: 1 in, 5 out]
                n1450 = Divide(x=w2124, y=i64 1024) -> (x/y=w2128:dbl)
                n1451 = Divide(x=w2128, y=i64 1024) -> (x/y=w2129:dbl)
                n1452 = Divide(x=w2129, y=i64 1024) -> (x/y=w2120:dbl)
                n1453 = Number To Fractional String(number=w2120, precision (6)=i16 1) -> (F-format string=w2121:string)  [unwired: 2 in]
                n1454 = Concatenate Strings("Pupil is beeing recorded! \nAvailable disk space: " ("string"), w2121, " GB" ("string")) -> (w2118:string)
                n1455 = One Button Dialog(message=w2118) -> ()  [unwired: 1 in, 1 out]
              }
            }
          }
          frame Enabled {
          }
        }
        n1456 = property on="Image Format Control::Offset X" class="Slide (strict)"("DisabledEnum"=T8."Disabled and Grayed Out" ("Disabled")) -> ()  [unwired: 2 in, 2 out]
        n1457 = property on="Image Format Control::Offset Y" class="Slide (strict)"("DisabledEnum"=T8."Disabled and Grayed Out" ("Disabled")) -> ()  [unwired: 2 in, 2 out]
        n1458 = property on="Gain" class="Slide (strict)"("DisabledEnum"=T8."Disabled and Grayed Out" ("Disabled")) -> ()  [unwired: 2 in, 2 out]
        n1459 = property on="Target frame rate" class="DigNum (strict)"("DisabledEnum"=T8."Disabled and Grayed Out" ("Disabled")) -> ()  [unwired: 2 in, 2 out]
        n1460 = while {
          stop <- w2135 stop-if-true
          n1461 = Wait (ms)(milliseconds to wait=u32 10) -> ()  [unwired: 1 out]
          n1462 = local read "Record loop state"() -> (w2137:T7)
          n1463 = Equal?(x=w2137, y=Record_enum."Record VR" ("Record loop state")) -> (x = y?=w2135:bool)
        }
        n1464 = local read "Pupil Exp day folder"() -> (w2106:path)
        n1465 = call <vilib>:"Check if File or Folder Exists.vi"("path"=w2106) -> ("file or folder exists?"=w2108:bool, "dup path"=w2107:path)  [unwired: 8 in, 1 out]
        n1466 = case shown="False" w2108 {
          tunnel: [w2131 w2133] -> _
          tunnel: w2107 -> [w2131 w2132]
          frame True {
          }
          frame False {
            n1467 = Create Folder(path (use dialog)=w2132) -> (created path=w2133:path)  [unwired: 2 in, 2 out]
          }
        }
        n1468 = property on="Exposure Time (ms)" class="Slide (strict)"("DisabledEnum"=T8."Disabled and Grayed Out" ("Disabled")) -> ()  [unwired: 2 in, 2 out]
        n1469 = property on="Black Level" class="Slide (strict)"("DisabledEnum"=T8."Disabled and Grayed Out" ("Disabled")) -> ()  [unwired: 2 in, 2 out]
      }
      frame "Record pupille" {
        n1470 = case shown="..0" w2138 {
          tunnel: [i64 100 ("Image Format Control::Offset Y") i64 102 ("Image Format Control::Offset Y") w2189] -> w2150
          tunnel: [i64 100 ("Image Format Control::Offset X") i64 102 ("Image Format Control::Offset X") w2190] -> w2149
          tunnel: [29.0 ("Target frame rate") 28.0 ("Target frame rate") w2191] -> w2147
          tunnel: [10.0 ("Gain") 9.0 ("Gain") w2192] -> w2145
          tunnel: [0.0 ("Black Level") 1.0 ("Black Level") w2193] -> w2143
          tunnel: [5000.0 5500.0 w2194] -> w2141
          tunnel: w2140 -> [_ _ w2194]
          tunnel: w2142 -> [_ _ w2193]
          tunnel: w2144 -> [_ _ w2192]
          tunnel: w2146 -> [_ _ w2191]
          tunnel: w2148 -> [_ _ w2190]
          tunnel: w2151 -> [_ _ w2189]
          selector: w2138 -> [_ _ w2188]
          tunnel: [1 2 w2188] -> w2139
          frame ..0 {
          }
          frame 1 {
          }
          frame 2.. {
          }
        }
        n1471 = local read "Run experiment"() -> (w2170:bool)
        n1472 = local read "Exit"() -> (w2169:bool)
        n1473 = Not(x=w2170) -> (.not. x?=w2168:bool)
        n1474 = Compound Arithmetic op=OR(w2168, w2169) -> (w2167:bool)
        n1475 = call "Vision Acquisition3"("Analog Control::Gain"=w2145, "Analog Control::Black Level"=w2143, "Acquisition Control::Exposure Time"=w2141, "Acquisition Control::Acquisition Frame Rate"=w2147, "Image Format Control::Offset X"=w2149, "Stop (F)"=w2167, "Image Format Control::Offset Y"=w2150) -> ("Image Out"=w2166:T3, "Lost Image Count"=w2152:u32, "Total Images Transferred"=w2153:u32, "Frame Rate"=w2173:dbl, "Stopped"=w2165:bool)  [unwired: 13 in, 3 out]
        n1476 = local write "Frame rate"(w2173) -> ()
        n1477 = local write "Pupille image"(w2166) -> ()
        n1478 = local write "Lost Image Count"(w2152) -> ()
        n1479 = local write "Total Images Transferred"(w2153) -> ()
        n1480 = local read "Pupil Exp day folder"() -> (w2161:path)
        n1481 = local read "Run experiment"() -> (w2156:bool)
        n1482 = local read "Exit"() -> (w2158:bool)
        n1483 = local read "Record"() -> (w2155:bool)
        n1484 = local read "Filename"() -> (w2159:string)
        n1485 = Not(x=w2158) -> (.not. x?=w2157:bool)
        n1486 = Compound Arithmetic op=AND(w2155, w2156, w2157) -> (w2154:bool)
        n1487 = call "SavePupilCameraImages.vi"("Save Format"=enum16{"Png", "Raw"}."Raw", "Save Image?"=w2154, "Block Folder"=w2161, "Subfolder"=w2159, "Refnum in"=w2166) -> ("ImageSaved"=w2160:bool)  [unwired: 5 in, 1 out]
        n1488 = local write "Pupille image saved"(w2160) -> ()
        n1489 = Select(t=T6."Stop recording" ("Eyecam states"), s=w2165, f=T6."Record pupille" ("Eyecam states")) -> (s? t:f=w2172:T6)
      }
      frame "Stop recording" {
        w2202 = FALSE ("Record Button 2")
        n1490 = property on="Image Format Control::Offset X" class="Slide (strict)"("DisabledEnum"=T8."Enabled" ("Disabled")) -> ()  [unwired: 2 in, 2 out]
        n1491 = property on="Image Format Control::Offset Y" class="Slide (strict)"("DisabledEnum"=T8."Enabled" ("Disabled")) -> ()  [unwired: 2 in, 2 out]
        n1492 = local write "Record Button 2"(w2202) -> ()
        n1493 = local write "Pupille image saved"(w2202) -> ()
        n1494 = property on="Gain" class="Slide (strict)"("DisabledEnum"=T8."Enabled" ("Disabled")) -> ()  [unwired: 2 in, 2 out]
        n1495 = property on="Target frame rate" class="DigNum (strict)"("DisabledEnum"=T8."Enabled" ("Disabled")) -> ()  [unwired: 2 in, 2 out]
        n1496 = property on="Exposure Time (ms)" class="Slide (strict)"("DisabledEnum"=T8."Enabled" ("Disabled")) -> ()  [unwired: 2 in, 2 out]
        n1497 = property on="Black Level" class="Slide (strict)"("DisabledEnum"=T8."Enabled" ("Disabled")) -> ()  [unwired: 2 in, 2 out]
      }
    }
    "Eyecam states" <- w2013
  }
  n1498 = while {
    stop <- w2214 stop-if-true
    n1499 = local read "Eable security cam"() -> (w2212:bool)
    n1500 = local read "Cam ON /OFF"() -> (w2213:bool)
    n1501 = Wait (ms)(milliseconds to wait=u32 20) -> ()  [unwired: 1 out]
    n1502 = And(x=w2213, y=w2212) -> (x .and. y?=w2211:bool)
    n1503 = case shown="False" w2211 {
      frame False {
        n1504 = local write "Security cam image"(T3 refnum ("Security cam image")) -> ()
      }
      frame True {
        n1505 = while {
          stop <- w2218 stop-if-true
          n1506 = local read "Cam ON /OFF"() -> (w2224:bool)
          n1507 = Not(x=w2224) -> (.not. x?=w2223:bool)
          n1508 = call "Vision Acquisition2"("Stop (F)"=w2223) -> ("Image Out"=→"Security cam image":T3, "Stopped"=w2220:bool, "error out"=w2222:errorcluster)  [unwired: 24 in]
          n1509 = local read "Exit"() -> (w2217:bool)
          n1510 = call <vilib>:"Find First Error.vi"("error in (no error)"=w2222) -> ("error?"=w2219:bool)  [unwired: 3 in, 1 out]
          n1511 = Compound Arithmetic op=OR(w2219, w2220, w2217) -> (w2218:bool)
        }
      }
    }
    n1512 = local read "Exit"() -> (w2214:bool)
  }
  n1513 = while {
    shift-right: [w2230] -> _
    shift-left: _ -> [w2229]
    shift-right: [w2231] -> _
    shift-left: _ -> [w2228]
    shift-right: [w2226] -> _
    shift-left: w76 -> [w2227]
    stop <- w2225 stop-if-true
    n1514 = case shown="\"Socket connected\"" w2227 {
      tunnel: [w2239 w2275 w2359 w2381] -> w2231
      tunnel: [w2240 w2277 w2360 w2382] -> w2230
      tunnel: w2229 -> [_ w2277 w2355 w2382]
      tunnel: w2228 -> [_ w2275 w2354 w2381]
      tunnel: [w2236 w2274 Socket_enum."Socket not connected" ("Enum") w2380] -> w2226
      tunnel: [w2235 FALSE FALSE ("Exit") w2376] -> w2225
      frame "Init socket", Default {
        n1515 = local read "Unity connected"() -> (w2234:bool)
        n1516 = local write "Read loop stopped"(FALSE ("Read loop stopped")) -> ()
        n1517 = local write "Write loop stopped"(FALSE ("Read loop stopped")) -> ()
        n1518 = local write "Unity connected"(FALSE ("Unity connected")) -> ()
        n1519 = case shown="False" w2234 {
          frame False {
            n1520 = flat-sequence {
              frame #0 {
                n1521 = Wait (ms)(milliseconds to wait=u32 200) -> ()  [unwired: 1 out]
              }
              frame #1 {
                n1522 = local read "command line"() -> (w2247:string)
                n1523 = property on="working directory 2" class="Path"("Visible"=TRUE) -> ()  [unwired: 2 in, 2 out]
                n1524 = call <vilib>:"System Exec.vi"("run minimized? (F)"=FALSE, "wait until completion? (T)"=FALSE, "working directory"="working directory 2", "command line"=w2247) -> ()  [unwired: 4 in, 4 out]
              }
              frame #2 {
                n1525 = Wait (ms)(milliseconds to wait=u32 800) -> ()  [unwired: 1 out]
              }
            }
          }
          frame True {
          }
        }
        n1526 = call <vilib>:"TCP Listen.vi"("timeout ms (wait forever: -1)"=10000, "port"=u16 11000) -> ("error out"=w2237:errorcluster, "connection ID"=w2238:refnum<k5>)  [unwired: 5 in, 3 out]
        n1527 = case shown="No Error" w2237 {
          tunnel: [w2260 w2266] -> w2240
          tunnel: [w2259 w2265] -> w2239
          tunnel: w2238 -> [w2258 w2266]
          tunnel: w2237 -> [w2257 w2265]
          tunnel: [Socket_enum."Socket connected" ("Enum") w2263] -> w2236
          frame No Error {
            n1528 = TCP Write(connection ID=w2258, data in="Start", error in (no error)=w2257, 9:-1 ("timeout ms (25000)")) -> (connection ID out=w2254:refnum<k5>, error out=w2252:errorcluster)  [unwired: 1 out]
            n1529 = TCP Write(connection ID=w2254, data in="Start", error in (no error)=w2252) -> (connection ID out=w2260:refnum<k5>, error out=w2259:errorcluster)  [unwired: 1 in, 1 out]
          }
          frame Error {
            n1530 = local read "VR Mode"() -> (w2264:bool)
            n1531 = Select(t=Socket_enum."Init socket" ("Enum"), s=w2264, f=Socket_enum."Socket not connected" ("Enum")) -> (s? t:f=w2263:T11)
          }
        }
        n1532 = local read "Exit"() -> (w2235:bool)
      }
      frame "Socket connected" {
        n1533 = Tick Count (ms)() -> (millisecond timer value=w2267:u32)
        n1534 = while {
          tunnel: w2277 -> [w2284]
          tunnel: w2275 -> [w2285]
          shift-right: [w2279] -> _
          shift-left: w2267 -> [w2280]
          stop <- w2283 stop-if-true
          n1535 = local read "read"() -> (w2282:bool)
          n1536 = case shown="True" w2282 {
            tunnel: w2284 -> [_ w2294]
            tunnel: w2285 -> [_ w2295]
            tunnel: [w2288 FALSE] -> w2283
            frame False {
              n1537 = local write "Read loop stopped"(TRUE ("Read loop stopped")) -> ()
              n1538 = local read "Exit"() -> (w2288:bool)
            }
            frame True {
              # "msg format: pos + CorridorIndicator + \",\" Position"
              n1539 = TCP Read(connection ID=w2294, bytes to read=20, error in (no error)=w2295, 7:T18."CRLF" ("mode (standard)"), 9:-1 ("timeout ms (25000)")) -> (data out=w2301:string)  [unwired: 2 out]
              n1540 = Match Pattern(string=w2301, regular expression=",", offset (0)=0) -> (after substring=w2305:string)  [unwired: 3 out]
              n1541 = Match Pattern(string=w2301, regular expression="pos") -> (after substring=w2298:string)  [unwired: 1 in, 3 out]
              n1542 = Match Pattern(string=w2298, regular expression="," ("after substring")) -> (before substring=w2297:string)  [unwired: 1 in, 3 out]
              n1543 = Match Pattern(string=w2305, regular expression="\\r\\n" ("after substring")) -> (before substring=w2303:string)  [unwired: 1 in, 3 out]
              n1544 = Decimal String To Number(string=w2297) -> ()  [unwired: 2 in, 2 out]
              n1545 = Fract/Exp String To Number(string=w2303) -> (number=w2289:dbl)  [unwired: 3 in, 1 out]
              n1546 = local write "Track position"(w2289) -> ()
              n1547 = local write "Read loop stopped"(FALSE ("Read loop stopped")) -> ()
            }
          }
          n1548 = local write "Unity connected"(TRUE ("Unity connected")) -> ()
          n1549 = Tick Count (ms)() -> (millisecond timer value=w2279:u32)
          n1550 = Subtract(x=w2279, y=w2280) -> (x-y=→"Socket read loop rate (ms)":u32)
          n1551 = Wait (ms)(milliseconds to wait=u32 1) -> ()  [unwired: 1 out]
        }
        n1552 = while {
          tunnel: w2277 -> [w2311]
          tunnel: w2275 -> [w2310]
          stop <- w2308 stop-if-true
          n1553 = local read "Write"() -> (w2309:bool)
          n1554 = case shown="True" w2309 {
            tunnel: w2311 -> [_ w2327]
            tunnel: w2310 -> [_ w2324]
            tunnel: [w2312 w2325] -> w2308
            frame False {
              n1555 = local read "Exit"() -> (w2312:bool)
            }
            frame True {
              n1556 = local read "VR Gain"() -> (w2314:dbl)
              n1557 = call "Is Value Changed.vim"("value"=w2314) -> ("changed or first call?"=w2315:bool)
              n1558 = case shown="False" w2315 {
                tunnel: [w2328 w2329] -> w2321
                tunnel: w2314 -> [_ w2332]
                frame False {
                  n1559 = local read "Encoder count"() -> (w2328:dbl)
                }
                frame True {
                  n1560 = local read "Encoder count"() -> (w2331:dbl)
                  n1561 = Multiply(x=w2331, y=w2332) -> (x*y=w2329:dbl)
                  n1562 = To Quad Integer(1:w2329) -> (0:w2330:i64)
                  n1563 = local write "Encoder count"(w2330) -> ()
                }
              }
              n1564 = local read "Read loop stopped"() -> (w2313:bool)
              n1565 = local read "encoder ticks per rev"() -> (w2320:dbl)
              n1566 = local read "Stop Unity"() -> (w2323:bool)
              n1567 = Divide(x=4000.0 ("y"), y=w2320) -> (x/y=w2318:dbl)
              n1568 = Multiply(x=w2318, y=w2321) -> (x*y=w2317:dbl)
              n1569 = And(x=w2323, y=w2313) -> (x .and. y?=w2322:bool)
              n1570 = Multiply(x=w2314, y=w2317) -> (x*y=w2316:dbl)
              n1571 = case shown="False" w2322 {
                tunnel: ["ext,\r\n" w2345] -> w2326
                tunnel: w2316 -> [_ w2344]
                tunnel: [TRUE FALSE] -> w2325
                frame True {
                  n1572 = disable-structure shown="Disabled" {
                    frame Disabled {
                      n1573 = local write "Write"(FALSE ("Write")) -> ()
                      n1574 = local write "Unity connected"(FALSE ("Unity connected")) -> ()
                    }
                    frame Enabled {
                    }
                  }
                  n1575 = local write "Write loop stopped"(TRUE ("Read loop stopped")) -> ()
                  n1576 = Wait (ms)(milliseconds to wait=u32 20) -> ()  [unwired: 1 out]
                }
                frame False {
                  n1577 = local read "offset tag"() -> (w2339:string)
                  n1578 = local read "msg tag"() -> (w2340:string)
                  n1579 = Number To Decimal String(number=w2344) -> (decimal integer string=w2342:string)  [unwired: 1 in]
                  n1580 = Concatenate Strings(w2340, w2339, w2342, "\r\n" ("string")) -> (w2345:string)
                }
              }
              n1581 = TCP Write(connection ID=w2327, data in=w2326, error in (no error)=w2324) -> ()  [unwired: 1 in, 3 out]
            }
          }
          n1582 = Wait (ms)(milliseconds to wait=u32 5) -> ()  [unwired: 1 out]
        }
        n1583 = local read "Stop Unity"() -> (w2271:bool)
        n1584 = local read "Exit"() -> (w2270:bool)
        n1585 = Compound Arithmetic op=OR(w2270, w2271) -> (w2269:bool)
        n1586 = Wait (ms)(milliseconds to wait=u32 10) -> ()  [unwired: 1 out]
        n1587 = Select(t=Socket_enum."Close socket" ("Enum"), s=w2269, f=Socket_enum."Socket connected" ("Enum")) -> (s? t:f=w2274:T11)
      }
      frame "Close socket" {
        n1588 = flat-sequence {
          tunnel: w2355 -> [w2362]
          tunnel: w2354 -> [w2361]
          tunnel: [w2364] -> w2353
          tunnel: [w2363] -> w2352
          tunnel: w2353 -> [w2368]
          tunnel: w2352 -> [w2367]
          tunnel: [w2368] -> w2351
          tunnel: [w2367] -> w2350
          tunnel: w2351 -> [w2371]
          tunnel: w2350 -> [w2372]
          tunnel: [w2370] -> w2349
          tunnel: [w2369] -> w2348
          frame #0 {
            n1589 = TCP Write(connection ID=w2362, data in="ext,\r\n", error in (no error)=w2361) -> (connection ID out=w2363:refnum<k5>, error out=w2364:errorcluster)  [unwired: 1 in, 1 out]
          }
          frame #1 {
            n1590 = Wait (ms)(milliseconds to wait=u32 50) -> ()  [unwired: 1 out]
          }
          frame #2 {
            n1591 = TCP Write(connection ID=w2372, data in="ext,\r\n", error in (no error)=w2371) -> (connection ID out=w2369:refnum<k5>, error out=w2370:errorcluster)  [unwired: 1 in, 1 out]
          }
        }
        n1592 = local write "Write"(FALSE ("Write")) -> ()
        n1593 = local write "Write loop stopped"(TRUE ("Read loop stopped")) -> ()
        n1594 = local write "Unity connected"(FALSE ("Unity connected")) -> ()
        n1595 = TCP Close Connection(connection ID=w2348, error in (no error)=w2349) -> (connection ID out=w2360:refnum<k5>, error out=w2359:errorcluster)  [unwired: 1 in]
      }
      frame "Socket not connected" {
        n1596 = local write "Unity connected"(FALSE ("Unity connected")) -> ()
        n1597 = Wait (ms)(milliseconds to wait=u32 1000) -> ()  [unwired: 1 out]
        n1598 = local read "VR Mode"() -> (w2379:bool)
        n1599 = local read "Exit"() -> (w2376:bool)
        n1600 = Select(t=Socket_enum."Init socket" ("Enum"), s=w2379, f=Socket_enum."Socket not connected" ("Enum")) -> (s? t:f=w2380:T11)
      }
    }
  }
  n1601 = disable-structure shown="Disabled" {
    frame Disabled {
      (unwired) string[][] [["User:", "username"], ["Loop rate:", "100"], ["Sampling rate:", "3000"], ["Encoder tisks:", ""], ["Recording folder:", ""], ["Enable VR mode (Y/N):", ""], ["Unity exe file:", ""]] ("Default variables 2")
      n1602 = local read "settings folder"() -> (w2385:path)
      n1603 = Build Path(base path=w2385, name or relative path="Default variables.txt") -> (appended path=w2386:path)
      n1604 = call-poly <vilib>:"Read Delimited Spreadsheet.vi"("file path (dialog if empty)"=w2386) -> ("all rows"=w2387:string[][])  [unwired: 9 in, 5 out]
      n1605 = Delete From Array(array=w2387, index (col)=0 ("disabled index (col)")) -> ()  [unwired: 2 in, 2 out]
    }
    frame Enabled {
    }
  }
  n1606 = local write "Save and exit"(FALSE ("Save and exit")) -> ()
  n1607 = property on="Record Button" class="Bool (strict)"("DisabledEnum"=w19) -> ()  [unwired: 2 in, 2 out]
  n1608 = property on="Stop recording" class="Bool (strict)"("DisabledEnum"=T8."Enabled" ("Disabled")) -> ()  [unwired: 2 in, 2 out]
  n1609 = property on="Start recording" class="Bool (strict)"("DisabledEnum"=w19) -> ()  [unwired: 2 in, 2 out]
  n1610 = property on="Path" class="Path" props=["Visible"]() -> ()  [unwired: 2 in, 3 out]
  n1611 = local write "Exit program"(FALSE ("Exit program")) -> ()
  n1612 = local write "Stop Unity"(FALSE ("Stop Unity")) -> ()
  n1613 = local write "Exit"(FALSE ("Exit")) -> ()
  n1614 = local write "Record"(FALSE ("Logg data")) -> ()
  n1615 = local write "Start recording"(FALSE ("Start recording")) -> ()
  n1616 = local write "Record Button"(FALSE ("Record Button")) -> ()
  n1617 = local write "VR Gain"(1.0 ("Gain")) -> ()
  n1618 = local read "Reward given"() -> (w23:u32)
  n1619 = disable-structure shown="Disabled" {
    frame Disabled {
      n1620 = stacked-sequence {
        frame #0 {
          n1621 = local write "Encoder count"(100.0 ("Encoder count")) -> ()
          n1622 = Wait (ms)(milliseconds to wait=u32 20) -> ()  [unwired: 1 out]
        }
        frame #1 {
          n1623 = local write "Encoder count"(11000.0 ("Encoder count")) -> ()
          n1624 = Wait (ms)(milliseconds to wait=u32 20) -> ()  [unwired: 1 out]
        }
        frame #2 {
          n1625 = local write "read"(FALSE ("read")) -> ()
          n1626 = local write "Stop Unity"(TRUE ("Exit")) -> ()
        }
      }
    }
    frame Enabled {
    }
  }
  n1627 = local read "Reward given"() -> (w24:u32)
  n1628 = local write "Store prev encoder count"(0.0 ("Store prev encoder count")) -> ()
  n1629 = local write "Open valve"(FALSE ("Open valve")) -> ()
  n1630 = Bundle(w10, w10) -> (w11:cluster{i32, i32})  [unwired: 1 in]
  n1631 = local write "Reward freq. (cm)"(100.0 ("Reward freq. (cm)")) -> ()
  n1632 = local write "Timed reward (s)"(u32 0 ("Timed reward (s)")) -> ()
  n1633 = for {
    N: 8 -> [_]
    i -> [w2394]
    n1634 = Bundle(w2394, 0) -> (w2396:cluster{i32, i32})  [unwired: 1 in]
    n1635 = property on="Behavior and VR signals saved" class="Tbl (strict)"("Active Cell"=w2396, "Cell BG Color"=u32 65295) -> ()  [unwired: 2 in, 2 out]
  }
  n1636 = for {
    N: 3 -> [_]
    i -> [w2398]
    n1637 = Bundle(w2398, 0) -> (w2399:cluster{i32, i32})  [unwired: 1 in]
    n1638 = property on="Saved 2P signals" class="Tbl (strict)"("Active Cell"=w2399, "Cell BG Color"=u32 65295) -> ()  [unwired: 2 in, 2 out]
  }
  n1639 = for {
    N: 4 -> [_]
    i -> [w2402]
    n1640 = Bundle(w2402, 0) -> (w2404:cluster{i32, i32})  [unwired: 1 in]
    n1641 = property on="Saved optogen. signals" class="Tbl (strict)"("Active Cell"=w2404, "Cell BG Color"=u32 65295) -> ()  [unwired: 2 in, 2 out]
  }
  n1642 = local write "random rew"(0.5 ("random rew")) -> ()
  n1643 = local write "Water cnt. reset"(0 ("Waret received")) -> ()
  n1644 = property on="Saved pupil imaging signals" class="Tbl (strict)"("Active Cell"=w11, "Cell BG Color"=u32 65295) -> ()  [unwired: 2 in, 2 out]
  n1645 = Equal?(x=w23, y=u32 0) -> ()  [unwired: 1 out]
  n1646 = call-poly <vilib>:"DAQmx Create Virtual Channel.vi"("lines"=tag "Dev1/port2/line6") -> ("task out"=w59:refnum<k21>)  [unwired: 13 in, 1 out]
  n1647 = call-poly <vilib>:"DAQmx Create Virtual Channel.vi"("lines"=tag "Dev1/port2/line5") -> ("task out"=w61:refnum<k21>)  [unwired: 13 in, 1 out]
  n1648 = local write "Valve open"(FALSE ("Valve open")) -> ()
  n1649 = local write "Repetition"(1 ("Repetition")) -> ()
  n1650 = local write "miss trial"(FALSE ("miss trial")) -> ()
  n1651 = Greater?(x=w24, y=u32 0) -> ()  [unwired: 1 out]
  n1652 = Build Path(base path=w1, name or relative path="Laser stimulus calibration.txt") -> (appended path=w3:path)
  n1653 = Tick Count (ms)() -> (millisecond timer value=w51:u32)
  n1654 = call <vilib>:"Check if File or Folder Exists.vi"("path"=w3) -> ("file or folder exists?"=w4:bool)  [unwired: 8 in, 2 out]
  n1655 = while {
    shift-right: [w2456] -> _
    shift-left: _ -> [w2455]
    stop <- w2457 stop-if-true
    w2437 = 100.0 ("y")
    # "Reward zone available?"
    n1656 = case shown="True" TRUE {
      tunnel: [w2522 w2600] -> w2456
      tunnel: w2455 -> [w2517 w2595]
      frame True {
        # "Clear graph history in every 1 min"
        n1657 = local read "Trials in session array"() -> (w2496:u16[][])
        n1658 = local read "Record loop state"() -> (w2491:T7)
        n1659 = local read "All trials"() -> (w2495:i32)
        n1660 = Tick Count (ms)() -> (millisecond timer value=w2521:u32)
        n1661 = local read "Stim trial"() -> (w2509:bool)
        n1662 = local read "Stim trial"() -> (w2506:bool)
        n1663 = Divide(x=w2521, y=u32 60000) -> (x/y=w2519:dbl)
        n1664 = local read "velocity (cm/s)"() -> (w2501:dbl)
        n1665 = local read "Track position"() -> (w2492:sgl)
        "?" <- w2492
        n1666 = Subtract(x=w2519, y=w2517) -> (x-y=w2518:dbl)
        n1667 = Index Array(array=w2496, index (row)=w2495, index (col)=1 ("disabled index (col)")) -> (element=w2493:u16)
        n1668 = Equal?(x=w2491, y=Record_enum."Record VR" ("Record loop state")) -> (x = y?=w2488:bool)
        n1669 = call "Is Value Changed.vim"("value"=w2488) -> ("changed or first call?"=w2489:bool)
        n1670 = Greater?(x=w2518, y=1.0) -> (0:w2485:bool)
        n1671 = Equal?(x="plot selector bool 1", y=w2509) -> (x = y?=w2511:bool)
        n1672 = Equal?(x="plot selector 1", y=w2493) -> (x = y?=w2510:bool)
        n1673 = Equal?(x=w2493, y="plot selector 2") -> (x = y?=w2512:bool)
        n1674 = Equal?(x=w2506, y="plot selector bool 2") -> (x = y?=w2513:bool)
        n1675 = And(x=w2489, y=w2488) -> (x .and. y?=w2486:bool)
        n1676 = And(x=w2511, y=w2510) -> (x .and. y?=w2503:bool)
        n1677 = And(x=w2512, y=w2513) -> (x .and. y?=w2502:bool)
        n1678 = Or(x=w2486, y=w2485) -> (x .or. y?=w2487:bool)
        n1679 = case shown="False" w2487 {
          tunnel: [w2572 w2581] -> w2522
          tunnel: w2517 -> [w2573 _]
          tunnel: ["Reset bottom plot" w2580] -> w2515
          tunnel: ["Reset top plot" w2580] -> w2514
          frame False {
            n1680 = Or(x="Reset bottom plot", y="Reset top plot") -> (x .or. y?=w2571:bool)
            n1681 = case shown="True" w2571 {
              tunnel: w2573 -> [w2576 _]
              tunnel: [w2576 w2577] -> w2572
              frame False {
              }
              frame True {
                n1682 = Tick Count (ms)() -> (millisecond timer value=w2579:u32)
                n1683 = Divide(x=w2579, y=u32 60000) -> (x/y=w2577:dbl)
              }
            }
          }
          frame True {
            w2580 = TRUE ("Reset NBC plot")
            n1684 = Tick Count (ms)() -> (millisecond timer value=w2582:u32)
            n1685 = Divide(x=w2582, y=u32 60000) -> (x/y=w2581:dbl)
          }
        }
        n1686 = call "Is New Trial - graph loop.vi"("Position data"=w2492) -> ("Boolean"=w2498:bool)  [unwired: 1 in]
        n1687 = local read "Valve open"() -> (w2531:bool)
        n1688 = local read "Valve open"() -> (w2536:bool)
        n1689 = local read "lick signal"() -> (w2546:i8[])
        n1690 = local read "lick signal"() -> (w2555:i8[])
        n1691 = call "Is Value Changed.vim"("value"=w2498) -> ("changed or first call?"=w2497:bool)
        n1692 = case shown="False" w2498 {
          tunnel: [w2567 w2569] -> w2499
          tunnel: w2501 -> [w2568 w2569]
          tunnel: w2492 -> [w2564 _]
          tunnel: [w2566 inf ("velocity (cm/s)")] -> w2500
          tunnel: w2497 -> [w2563 _]
          frame False {
            n1693 = Select(t=-inf ("velocity (cm/s)"), s=w2563, f=w2564) -> (s? t:f=w2566:dbl)
            n1694 = Select(t=-99.0, s=w2563, f=w2568) -> (s? t:f=w2567:dbl)
          }
          frame True {
          }
        }
        n1695 = Index Array(array=w2546, index=0) -> (element=w2548:i8)
        n1696 = Boolean To (0,1)(Boolean=w2531) -> (0, 1=w2529:i16)
        n1697 = Index Array(array=w2555, index=0) -> (element=w2552:i8)
        n1698 = Boolean To (0,1)(Boolean=w2536) -> (0, 1=w2534:i16)
        n1699 = Multiply(x=w2548, y=100) -> (x*y=w2523:i32)
        n1700 = Multiply(x=w2529, y=-20) -> (x*y=w2530:i32)
        n1701 = Multiply(x=w2552, y=100) -> (x*y=w2551:i32)
        n1702 = Multiply(x=w2534, y=-20) -> (x*y=w2535:i32)
        n1703 = call "Build XY Graph"("Enable"=w2503, "Reset"=w2514, "Y Input"=w2499, "X Input"=w2500) -> ("XY Graph"=w2557:cluster{"X":dbl[], "Y":dbl[]}[])  [unwired: 6 in, 1 out]
        n1704 = call "Build XY Graph4"("Enable"=w2503, "Reset"=w2514, "Y Input"=w2551, "X Input"=w2500) -> ("XY Graph"=w2560:cluster{"X":dbl[], "Y":dbl[]}[])  [unwired: 6 in, 1 out]
        n1705 = call "Build XY Graph3"("Enable"=w2503, "Reset"=w2514, "Y Input"=w2535, "X Input"=w2500) -> ("XY Graph"=w2545:cluster{"X":dbl[], "Y":dbl[]}[])  [unwired: 6 in, 1 out]
        n1706 = call "Build XY Graph2"("Enable"=w2502, "Reset"=w2515, "Y Input"=w2523, "X Input"=w2500) -> ("XY Graph"=w2537:cluster{"X":dbl[], "Y":dbl[]}[])  [unwired: 6 in, 1 out]
        n1707 = call "Build XY Graph5"("Enable"=w2502, "Reset"=w2515, "Y Input"=w2499, "X Input"=w2500) -> ("XY Graph"=w2542:cluster{"X":dbl[], "Y":dbl[]}[])  [unwired: 6 in, 1 out]
        n1708 = call "Build XY Graph6"("Enable"=w2502, "Reset"=w2515, "Y Input"=w2530, "X Input"=w2500) -> ("XY Graph"=w2540:cluster{"X":dbl[], "Y":dbl[]}[])  [unwired: 6 in, 1 out]
        n1709 = Index Array(array=w2557, index=0) -> (element=w2524:cluster{"X":dbl[], "Y":dbl[]})
        n1710 = Index Array(array=w2560, index=0) -> (element=w2556:cluster{"X":dbl[], "Y":dbl[]})
        n1711 = Index Array(array=w2545, index=0) -> (element=w2541:cluster{"X":dbl[], "Y":dbl[]})
        n1712 = Index Array(array=w2542, index=0) -> (element=w2528:cluster{"X":dbl[], "Y":dbl[]})
        n1713 = Index Array(array=w2537, index=0) -> (element=w2527:cluster{"X":dbl[], "Y":dbl[]})
        n1714 = Index Array(array=w2540, index=0) -> (element=w2526:cluster{"X":dbl[], "Y":dbl[]})
        n1715 = Build Array(w2528, w2527, w2526) -> (→"Bottom Graph":cluster{"X":dbl[], "Y":dbl[]}[])
        n1716 = Build Array(w2524, w2556, w2541) -> (→"Top Graph":cluster{"X":dbl[], "Y":dbl[]}[])
        n1717 = Wait (ms)(milliseconds to wait=u32 20) -> ()  [unwired: 1 out]
      }
      frame False {
        # "Clear graph history in every 5 min"
        n1718 = local read "Reward zone"() -> (w2590:bool)
        n1719 = Tick Count (ms)() -> (millisecond timer value=w2599:u32)
        n1720 = case shown="False" w2590 {
          tunnel: [w2635 w2637] -> w2591
          frame False {
            n1721 = local read "Distance (cm)"() -> (w2634:dbl)
            n1722 = local read "Prev. rew. pos."() -> (w2636:dbl)
            n1723 = Subtract(x=w2634, y=w2636) -> (x-y=w2635:dbl)
          }
          frame True {
            n1724 = local read "Track position"() -> (w2637:sgl)
          }
        }
        n1725 = Divide(x=w2599, y=u32 60000) -> (x/y=w2597:dbl)
        n1726 = Subtract(x=w2597, y=w2595) -> (x-y=w2596:dbl)
        n1727 = Greater?(x=w2596, y=2.0) -> (0:w2592:bool)
        n1728 = case shown="False" w2592 {
          tunnel: [w2639 w2646] -> w2600
          tunnel: w2595 -> [w2640 _]
          tunnel: ["Reset wheel pos. graph" TRUE ("Reset NBC plot")] -> w2593
          frame False {
            n1729 = case shown="False" "Reset wheel pos. graph" {
              tunnel: w2640 -> [w2641 _]
              tunnel: [w2641 w2642] -> w2639
              frame False {
              }
              frame True {
                n1730 = Tick Count (ms)() -> (millisecond timer value=w2644:u32)
                n1731 = Divide(x=w2644, y=u32 60000) -> (x/y=w2642:dbl)
              }
            }
          }
          frame True {
            n1732 = Tick Count (ms)() -> (millisecond timer value=w2647:u32)
            n1733 = Divide(x=w2647, y=u32 60000) -> (x/y=w2646:dbl)
          }
        }
        n1734 = local read "Random reward"() -> (w2587:bool)
        n1735 = local read "Reward zone"() -> (w2588:bool)
        n1736 = local read "lick signal"() -> (w2614:i8[])
        n1737 = call "Is Value Changed.vim"("value"=w2588) -> ("changed or first call?"=w2585:bool)
        n1738 = call "Is Value Changed.vim"("value"=w2587) -> ("changed or first call?"=w2586:bool)
        n1739 = local read "Valve open"() -> (w2605:bool)
        n1740 = local read "velocity (cm/s)"() -> (w2589:dbl)
        n1741 = Or(x=w2585, y=w2586) -> (x .or. y?=w2584:bool)
        n1742 = case shown="True" w2584 {
          tunnel: w2588 -> [_ w2633]
          tunnel: w2587 -> [_ w2622]
          frame False {
          }
          frame True {
            n1743 = local read "Reward freq. (cm)"() -> (w2627:u32)
            n1744 = local read "Reward freq. (cm)"() -> (w2630:u32)
            n1745 = local read "Wheel circumference"() -> (w2632:dbl)
            n1746 = Multiply(x=w2627, y=2.0) -> (x*y=w2624:dbl)
            n1747 = Add(x=w2630, y=20.0) -> (x+y=w2623:dbl)
            n1748 = Add(x=w2624, y=20.0) -> (x+y=w2626:dbl)
            n1749 = Select(t=w2626, s=w2622, f=w2623) -> (s? t:f=w2621:dbl)
            n1750 = Select(t=w2632, s=w2633, f=w2621) -> (s? t:f=w2625:dbl)
            n1751 = property on="Wheel position graph" class="XYGraph (strict)"("XScale.Maximum"=w2625) -> ()  [unwired: 2 in, 2 out]
          }
        }
        n1752 = Index Array(array=w2614, index=0) -> (element=w2611:i8)
        n1753 = Boolean To (0,1)(Boolean=w2605) -> (0, 1=w2603:i16)
        n1754 = Multiply(x=w2611, y=100) -> (x*y=w2610:i32)
        n1755 = Multiply(x=w2603, y=-20) -> (x*y=w2604:i32)
        n1756 = call "Build XY Graph7"("Reset"=w2593, "Y Input"=w2589, "X Input"=w2591) -> ("XY Graph"=w2616:cluster{"X":dbl[], "Y":dbl[]}[])  [unwired: 7 in, 1 out]
        n1757 = call "Build XY Graph8"("Reset"=w2593, "Y Input"=w2610, "X Input"=w2591) -> ("XY Graph"=w2619:cluster{"X":dbl[], "Y":dbl[]}[])  [unwired: 7 in, 1 out]
        n1758 = call "Build XY Graph9"("Reset"=w2593, "Y Input"=w2604, "X Input"=w2591) -> ("XY Graph"=w2608:cluster{"X":dbl[], "Y":dbl[]}[])  [unwired: 7 in, 1 out]
        n1759 = Index Array(array=w2616, index=0) -> (element=w2601:cluster{"X":dbl[], "Y":dbl[]})
        n1760 = Index Array(array=w2619, index=0) -> (element=w2615:cluster{"X":dbl[], "Y":dbl[]})
        n1761 = Index Array(array=w2608, index=0) -> (element=w2606:cluster{"X":dbl[], "Y":dbl[]})
        n1762 = Build Array(w2601, w2615, w2606) -> (→"Wheel position graph":cluster{"X":dbl[], "Y":dbl[]}[])
        n1763 = Wait (ms)(milliseconds to wait=u32 20) -> ()  [unwired: 1 out]
      }
    }
    n1764 = disable-structure shown="Disabled" {
      frame Disabled {
        n1765 = local read "VR Mode"() -> ()  [unwired: 1 out]
      }
      frame Enabled {
      }
    }
    n1766 = local write "Lab book notes"("Lab book notes") -> ()
    n1767 = local write "Record 2P"("Record 2P") -> ()
    n1768 = local write "Reward zone"("Reward zone") -> ()
    n1769 = Not(x="Reward zone") -> (.not. x?=w2448:bool)
    n1770 = property on="Reward freq. (cm)" class="DigNum (strict)"("Visible"=w2448) -> ()  [unwired: 2 in, 2 out]
    n1771 = property on="Timed reward (s)" class="DigNum (strict)"("Visible"=w2448) -> ()  [unwired: 2 in, 2 out]
    n1772 = local read "current VR context"() -> (w2434:u16)
    n1773 = local read "zeward zones"() -> (w2435:i16[][])
    n1774 = local read "Eye cam frame signal"() -> (w2410:i8[])
    n1775 = local read "Hit trials stim."() -> (w2442:i32)
    n1776 = local read "Hit trials ctrl."() -> (w2444:i32)
    n1777 = Delete From Array(array=w2435, index (row)=w2434) -> (deleted portion=w2436:i16[])  [unwired: 2 in, 1 out]
    n1778 = local read "Stim. count"() -> (w2443:i32)
    n1779 = local read "Ctrl. count"() -> (w2445:i32)
    n1780 = local read "Reward zone"() -> (w2426:bool)
    n1781 = local read "Frame signal"() -> (w2414:i8[])
    n1782 = Decimate 1D Array(w2436) -> (w2433:i16[], w2432:i16[])
    n1783 = local read "Context command"() -> (w2446:u16)
    n1784 = local read "Active licking"() -> (w2450:bool)
    n1785 = Add Array Elements(numeric array=w2433) -> (sum=w2431:i16)
    n1786 = Add Array Elements(numeric array=w2432) -> (sum=w2430:i16)
    n1787 = call "Is Value Changed.vim"("value"=w2426) -> ("changed or first call?"=w2425:bool)
    n1788 = Less?(x=w2431, y=w2430) -> (x < y?=w2429:bool)
    n1789 = call "Is Value Changed.vim"("value"=w2429) -> ("changed or first call?"=w2427:bool)
    n1790 = Or(x=w2425, y=w2427) -> (x .or. y?=w2428:bool)
    n1791 = Divide(x=w2442, y=w2443) -> (x/y=w2439:dbl)
    "P stim. Hit" <- w2439
    n1792 = Divide(x=w2444, y=w2445) -> (x/y=w2440:dbl)
    "P ctrl. Hit" <- w2440
    n1793 = Add Array Elements(numeric array=w2410) -> (sum=w2411:i8)
    n1794 = Add Array Elements(numeric array=w2414) -> (sum=w2413:i8)
    n1795 = case shown="True" w2428 {
      tunnel: w2426 -> [_ w2469]
      tunnel: w2429 -> [_ w2468]
      frame False {
      }
      frame True {
        n1796 = case shown="True" w2469 {
          tunnel: w2468 -> [_ w2474]
          frame False {
            n1797 = local write "Active licking"(FALSE ("Enable")) -> ()
            n1798 = property on="Active licking" class="Bool (strict)"("DisabledEnum"=T8."Disabled and Grayed Out" ("Disabled")) -> ()  [unwired: 2 in, 2 out]
            n1799 = property on="Random reward" class="Bool (strict)"("DisabledEnum"=T8."Enabled" ("Disabled"), "Visible"=TRUE) -> ()  [unwired: 2 in, 2 out]
          }
          frame True {
            n1800 = local write "Random reward"(FALSE ("Random reward")) -> ()
            n1801 = Select(t=TRUE ("Enable"), s=w2474, f=FALSE ("Enable")) -> (s? t:f=w2480:bool)
            n1802 = Select(t=T8."Enabled" ("Disabled"), s=w2474, f=T8."Disabled and Grayed Out" ("Disabled")) -> (s? t:f=w2479:T8)
            n1803 = local write "Active licking"(w2480) -> ()
            n1804 = property on="Random reward" class="Bool (strict)"("DisabledEnum"=T8."Disabled" ("Disabled"), "Visible"=FALSE) -> ()  [unwired: 2 in, 2 out]
            n1805 = property on="Active licking" class="Bool (strict)"("DisabledEnum"=w2479) -> ()  [unwired: 2 in, 2 out]
          }
        }
      }
    }
    n1806 = Array Size(array=w2410) -> (size(s)=w2407:i32)
    n1807 = Array Size(array=w2414) -> (size(s)=w2424:i32)
    n1808 = call "Is Value Changed.vim"("value"=w2450) -> ("changed or first call?"=w2449:bool)
    n1809 = Divide(x=w2411, y=w2407) -> (x/y=w2408:dbl)
    n1810 = Divide(x=w2413, y=w2424) -> (x/y=w2423:dbl)
    n1811 = call "Is Value Changed.vim"("value"=w2446) -> ("changed or first call?"=w2447:bool)
    n1812 = case shown="True" w2449 {
      frame False {
      }
      frame True {
        n1813 = local read "Active licking"() -> (w2464:bool)
        n1814 = Select(t=T8."Enabled" ("Disabled"), s=w2464, f=T8."Disabled and Grayed Out") -> (s? t:f=w2466:T8)
        n1815 = property on="Hybrid licking" class="Bool (strict)"("DisabledEnum"=w2466) -> ()  [unwired: 2 in, 2 out]
      }
    }
    n1816 = case shown="True" w2447 {
      tunnel: w2446 -> [_ w2458]
      frame False {
      }
      frame True {
        n1817 = local read "corridor lengths"() -> (w2462:i32[])
        n1818 = local read "teleports"() -> (w2463:i16[])
        n1819 = Index Array(array=w2463, index=w2458) -> (element=w2461:i16)
        n1820 = Index Array(array=w2462, index=w2458) -> (element=w2460:i32)
        n1821 = Subtract(x=w2461, y=w2460) -> (x-y=w2459:i32)
        n1822 = property on="Top Graph" class="XYGraph (strict)"("XScale.Maximum"=w2461, "XScale.Minimum"=w2459) -> ()  [unwired: 2 in, 2 out]
        n1823 = property on="Bottom Graph" class="XYGraph (strict)"("XScale.Maximum"=w2461, "XScale.Minimum"=w2459) -> ()  [unwired: 2 in, 2 out]
        n1824 = property on="Position bar" class="Slide (strict)"("Scale.Maximum"=w2461, "Scale.Minimum"=w2459) -> ()  [unwired: 2 in, 2 out]
      }
    }
    n1825 = Greater?(x=w2408, y=0.1) -> (0:→"EyeCam frame signal rec.":bool)
    n1826 = Greater?(x=w2423, y=0.1) -> (0:→"Frame signal 1 rec.":bool)
    n1827 = Multiply(x=w2440, y=w2437) -> (x*y=→"Control hit trials %":dbl)
    n1828 = Multiply(x=w2437, y=w2439) -> (x*y=→"Stim. hit trials %":dbl)
    n1829 = local read "Frame signal 2"() -> (w2415:i8[])
    n1830 = Add Array Elements(numeric array=w2415) -> (sum=w2417:i8)
    n1831 = Array Size(array=w2415) -> (size(s)=w2418:i32)
    n1832 = case shown="False" "Random reward" {
      frame False {
      }
      frame True {
        n1833 = local write "Active licking"(FALSE ("Enable")) -> ()
      }
    }
    n1834 = Divide(x=w2417, y=w2418) -> (x/y=w2419:dbl)
    n1835 = local read "Exit"() -> (w2457:bool)
    n1836 = Greater?(x=w2419, y=0.1) -> (0:→"Frame signal 2 rec.":bool)
  }
  n1837 = while {
    tunnel: w61 -> [w2677]
    tunnel: w59 -> [w2667]
    shift-right: [w2669] -> _
    shift-left: w51 -> [w2668]
    shift-right: [w2659] -> _
    shift-left: _ -> [w2658]
    stop <- w2683 stop-if-true
    n1838 = local read "Repetition"() -> (w2679:i32)
    n1839 = local read "Reward zone"() -> (w2671:bool)
    n1840 = case shown="True" w2671 {
      tunnel: [w2725 w2785] -> w2651
      tunnel: [w2729 w2784] -> w2672
      tunnel: w2658 -> [w2727 _]
      tunnel: [w2726 w2783] -> w2656
      tunnel: [w2724 w2782] -> w2654
      frame False {
        n1841 = local read "Random reward"() -> (w2728:bool)
        n1842 = case shown="False" w2728 {
          tunnel: [w2730 FALSE] -> w2729
          tunnel: w2727 -> [w2734 w2776]
          tunnel: [w2730 w2762] -> w2726
          tunnel: [FALSE ("Active rew within RZ") w2761] -> w2725
          tunnel: [FALSE ("Passive rew after RZ") w2759] -> w2724
          frame True {
            n1843 = local read "Reward freq. (cm)"() -> (w2748:u32)
            n1844 = local read "Timed reward (s)"() -> (w2743:u32)
            n1845 = local read "random rew"() -> (w2746:dbl)
            n1846 = local read "Prev. rew. pos."() -> (w2750:dbl)
            n1847 = local read "Distance (cm)"() -> (w2751:dbl)
            n1848 = Tick Count (ms)() -> (millisecond timer value=w2742:u32)
            n1849 = Multiply(x=w2743, y=u32 1000) -> (x*y=w2739:u32)
            n1850 = Multiply(x=w2748, y=2.0) -> (x*y=w2745:dbl)
            n1851 = Add(x=w2734, y=w2739) -> (x+y=w2741:u32)
            n1852 = Multiply(x=w2745, y=w2746) -> (x*y=w2744:dbl)
            n1853 = Greater?(x=w2739, y=u32 999) -> (0:w2738:bool)
            n1854 = Greater?(x=w2742, y=w2741) -> (0:w2740:bool)
            n1855 = Add(x=w2750, y=w2744) -> (x+y=w2749:dbl)
            n1856 = And(x=w2740, y=w2738) -> (x .and. y?=w2737:bool)
            n1857 = Greater?(x=w2751, y=w2749) -> (0:w2733:bool)
            n1858 = Or(x=w2733, y=w2737) -> (x .or. y?=w2730:bool)
          }
          frame False {
            n1859 = local read "Reward freq. (cm)"() -> (w2767:u32)
            n1860 = local read "Timed reward (s)"() -> (w2779:u32)
            n1861 = local read "Prev. rew. pos."() -> (w2769:dbl)
            n1862 = local read "Distance (cm)"() -> (w2770:dbl)
            n1863 = local read "Lick indicator"() -> (w2764:dbl)
            n1864 = Multiply(x=w2779, y=u32 1000) -> (x*y=w2773:u32)
            n1865 = Subtract(x=w2770, y=w2769) -> (x-y=w2752:dbl)
            n1866 = Greater?(x=w2764, y=0.1) -> (0:w2754:bool)
            n1867 = Add(x=w2767, y=u32 20) -> (x+y=w2768:u32)
            n1868 = Add(x=w2776, y=w2773) -> (x+y=w2775:u32)
            n1869 = Tick Count (ms)() -> (millisecond timer value=w2777:u32)
            n1870 = Build Array(w2767, w2768) -> (w2758:u32[])
            n1871 = Greater?(x=w2773, y=u32 999) -> (0:w2771:bool)
            n1872 = Greater?(x=w2777, y=w2775) -> (0:w2774:bool)
            n1873 = call "Analyze reward conditions - No RZ.vi"("Lick event"=w2754, "Array"=w2758, "reward given"=u32 0, "mouse position"=w2752) -> ("Active rew within RZ"=w2756:bool, "Passive rew within RZ"=w2757:bool, "Passive rew after RZ"=w2755:bool)  [unwired: 4 in, 1 out]
            n1874 = And(x=w2774, y=w2771) -> (x .and. y?=w2760:bool)
            n1875 = Or(x=w2757, y=w2760) -> (x .or. y?=w2762:bool)
            n1876 = Or(x=w2756, y=w2760) -> (x .or. y?=w2761:bool)
            n1877 = Or(x=w2755, y=w2760) -> (x .or. y?=w2759:bool)
          }
        }
      }
      frame True {
        n1878 = local read "VR Mode"() -> (w2780:bool)
        n1879 = case shown="True" TRUE {
          tunnel: [FALSE ("Active rew within RZ") w2804] -> w2785
          tunnel: [w2789 w2802] -> w2784
          tunnel: [w2786 w2805] -> w2783
          tunnel: [FALSE ("Passive rew after RZ") w2803] -> w2782
          frame False {
            n1880 = disable-structure shown="Disabled" {
              disable-tunnel: [w2796 _] -> w2786
              frame Disabled {
                w2797 = 0 ("element")
                n1881 = local read "Track position"() -> (w2792:sgl)
                n1882 = local read "Reward given"() -> (w2793:u32)
                n1883 = local read "Lick indicator"() -> (w2799:dbl)
                n1884 = Greater?(x=w2799, y=0.1) -> (0:w2794:bool)
                n1885 = Build Array(w2797, w2797) -> (w2795:i32[])
                n1886 = call "Analyze reward conditions - No VR.vi"("Lick event"=w2794, "Array"=w2795, "reward given"=w2793, "mouse position"=w2792) -> ("Passive rew within RZ"=w2796:bool)  [unwired: 4 in, 3 out]
              }
              frame Enabled {
              }
            }
            n1887 = local read "Track position"() -> (w2788:sgl)
            n1888 = Greater?(x=w2788, y=sgl 100.0) -> (0:w2789:bool)
          }
          frame True {
            n1889 = local read "current VR context"() -> (w2811:u16)
            n1890 = local read "zeward zones"() -> (w2812:i16[][])
            n1891 = local read "Lick indicator"() -> (w2807:dbl)
            n1892 = local read "Track position"() -> (w2813:sgl)
            n1893 = local read "Reward given"() -> (w2809:u32)
            n1894 = Delete From Array(array=w2812, index (row)=w2811) -> (deleted portion=w2810:i16[])  [unwired: 2 in, 1 out]
            n1895 = Greater?(x=w2807, y=0.1) -> (0:w2806:bool)
            n1896 = local read "Track position"() -> (w2801:sgl)
            n1897 = call "Analyze reward conditions.vi"("Lick event"=w2806, "Array"=w2810, "reward given"=w2809, "mouse position"=w2813) -> ("Active rew within RZ"=w2804:bool, "Passive rew within RZ"=w2805:bool, "Passive rew after RZ"=w2803:bool)  [unwired: 4 in, 1 out]
            n1898 = call "Is New Trial - reward loop.vi"("Position data"=w2801, "Minimum value drop"=-20.0) -> ("Boolean"=w2802:bool)
          }
        }
        n1899 = local write "VR Mode"(w2780) -> ()
      }
    }
    n1900 = case shown="True" "Give reward" {
      tunnel: w2667 -> [_ w2817]
      tunnel: w2679 -> [_ w2816]
      frame False {
      }
      frame True {
        n1901 = flat-sequence {
          tunnel: w2817 -> [w2823]
          tunnel: w2816 -> [w2818]
          frame #0 {
            n1902 = local read "Water cnt. reset"() -> (w2821:i32)
            n1903 = for {
              N: w2818 -> [_]
              tunnel: w2823 -> [w2825]
              n1904 = local read "Valve open dur. (ms)"() -> (w2824:u32)
              n1905 = local write "Valve open"(TRUE ("Valve open")) -> ()
              n1906 = call "SendTriggerPulse.vi"("Trigger Duration (ms)"=w2824, "Refnum in"=w2825) -> ()  [unwired: 9 in, 1 out]
            }
            n1907 = local read "Water count"() -> (w2819:i32)
            n1908 = Add(x=w2818, y=w2821) -> (x+y=w2822:i32)
            n1909 = Add(x=w2818, y=w2819) -> (x+y=w2820:i32)
            n1910 = local write "Water cnt. reset"(w2822) -> ()
            n1911 = local write "Water count"(w2820) -> ()
          }
          frame #1 {
            n1912 = local write "Valve open"(FALSE ("Valve open")) -> ()
          }
        }
      }
    }
    n1913 = case shown="True" w2672 {
      frame False {
      }
      frame True {
        n1914 = local write "Reward given"(u32 0 ("Reward given")) -> ()
      }
    }
    n1915 = local read "Hybrid licking"() -> (w2655:bool)
    n1916 = local read "Active licking"() -> (w2657:bool)
    n1917 = Select(t=w2654, s=w2655, f=FALSE) -> (s? t:f=w2652:bool)
    n1918 = Or(x=w2652, y=w2651) -> (x .or. y?=w2650:bool)
    n1919 = Select(t=w2650, s=w2657, f=w2656) -> (s? t:f=w2649:bool)
    n1920 = case shown="True" w2649 {
      tunnel: w2677 -> [_ w2690]
      tunnel: w2667 -> [_ w2689]
      tunnel: [w2684 w2686] -> w2659
      tunnel: w2658 -> [w2684 _]
      tunnel: w2654 -> [_ w2685]
      frame False {
      }
      frame True {
        n1921 = flat-sequence {
          tunnel: w2690 -> [w2694]
          tunnel: w2689 -> [w2693]
          tunnel: [w2693] -> w2688
          tunnel: [w2692] -> w2687
          tunnel: w2685 -> [w2691]
          tunnel: w2688 -> [w2709]
          tunnel: w2687 -> [w2703]
          tunnel: [w2702] -> w2686
          frame #0 {
            n1922 = case shown="True" w2691 {
              tunnel: w2694 -> [_ w2698]
              tunnel: [1 ("Repetition") w2696] -> w2692
              frame True {
              }
              frame False {
                n1923 = local read "Sound duration (ms)"() -> (w2697:u32)
                n1924 = local read "Repetition"() -> (w2696:i32)
                n1925 = call "SendTriggerPulse.vi"("Trigger Duration (ms)"=w2697, "Refnum in"=w2698) -> ()  [unwired: 9 in, 1 out]
              }
            }
          }
          frame #1 {
            n1926 = Random Number (0-1)() -> (number: 0 to 1=w2704:dbl)
            n1927 = local read "Water cnt. reset"() -> (w2708:i32)
            n1928 = local read "Water count"() -> (w2705:i32)
            n1929 = local write "random rew"(w2704) -> ()
            n1930 = Add(x=w2703, y=w2708) -> (x+y=w2707:i32)
            n1931 = Add(x=w2703, y=w2705) -> (x+y=w2706:i32)
            n1932 = local read "Reward given"() -> (w2701:u32)
            n1933 = for {
              N: w2703 -> [_]
              tunnel: w2709 -> [w2710]
              n1934 = stacked-sequence {
                tunnel: w2710 -> [w2713 _]
                frame #0 {
                  n1935 = local read "Valve open dur. (ms)"() -> (w2711:u32)
                  n1936 = local write "Valve open"(TRUE ("Valve open")) -> ()
                  n1937 = call "SendTriggerPulse.vi"("Trigger Duration (ms)"=w2711, "Refnum in"=w2713) -> ()  [unwired: 9 in, 1 out]
                  n1938 = Wait (ms)(milliseconds to wait=w2711) -> ()  [unwired: 1 out]
                }
                frame #1 {
                  n1939 = local read "Distance (cm)"() -> (w2714:dbl)
                  n1940 = local write "Valve open"(FALSE ("Valve open")) -> ()
                  n1941 = local write "Prev. rew. pos."(w2714) -> ()
                  n1942 = Wait (ms)(milliseconds to wait=u32 50) -> ()  [unwired: 1 out]
                }
              }
            }
            n1943 = local write "Water count"(w2706) -> ()
            n1944 = local write "Water cnt. reset"(w2707) -> ()
            n1945 = Add(x=w2701, y=u32 1) -> (x+y=w2699:u32)
            n1946 = local write "Reward given"(w2699) -> ()
            n1947 = Tick Count (ms)() -> (millisecond timer value=w2702:u32)
          }
        }
      }
    }
    n1948 = Tick Count (ms)() -> (millisecond timer value=w2669:u32)
    n1949 = local write "Active licking"("Active licking") -> ()
    n1950 = Subtract(x=w2669, y=w2668) -> (x-y=→"Reward read loop rate (ms)":u32)
    n1951 = local read "Lick indicator"() -> (w2675:dbl)
    n1952 = call "Is Value Changed.vim"("value"="Open valve") -> ("changed or first call?"=w2661:bool)
    n1953 = case shown="False" w2661 {
      tunnel: w2667 -> [_ w2721]
      tunnel: "Open valve" -> [_ w2720]
      frame False {
      }
      frame True {
        n1954 = call <vilib>:"DAQmx Start Task.vi"("task/channels in"=w2721) -> ("task out"=w2723:refnum<k21>)  [unwired: 13 in, 1 out]
        n1955 = call-poly <vilib>:"DAQmx Write.vi"("task/channels in"=w2723, "data"=w2720) -> ("task out"=w2722:refnum<k21>)  [unwired: 11 in, 2 out]
        n1956 = call <vilib>:"DAQmx Stop Task.vi"("task/channels in"=w2722) -> ()  [unwired: 13 in, 2 out]
      }
    }
    n1957 = Greater?(x=w2675, y=i8 0) -> (0:→"Lick":bool)
    n1958 = case shown="False" "Hybrid licking" {
      frame False {
      }
      frame True {
        n1959 = local write "Active licking"(TRUE ("Active licking")) -> ()
      }
    }
    n1960 = local read "Valve open"() -> (→"Valve open":bool)
    n1961 = case shown="False" "Boolean" {
      tunnel: [w2718 w2719] -> w2664
      frame False {
        n1962 = local read "Water cnt. reset"() -> (w2718:i32)
      }
      frame True {
        n1963 = local read "Water count"() -> (w2719:i32)
      }
    }
    n1964 = local read "Reward size (ul)"() -> (w2666:dbl)
    n1965 = case shown="False" "Reset water count" {
      frame False {
      }
      frame True {
        n1966 = local write "Water cnt. reset"(0 ("Waret received")) -> ()
        n1967 = local write "Reset water count"(FALSE ("Reset water count")) -> ()
      }
    }
    n1968 = local read "Exit"() -> (w2683:bool)
    n1969 = Multiply(x=w2664, y=w2666) -> (x*y=→"Water received (ul)":dbl)
    n1970 = Wait (ms)(milliseconds to wait=u32 5) -> ()  [unwired: 1 out]
  }
  n1971 = case shown="True" w4 {
    tunnel: w3 -> [_ w2829]
    frame False {
    }
    frame True {
      n1972 = Open/Create/Replace File(file path (use dialog)=w2829, operation (0:open)=T9."open", access (0:read/write)=enum16{"read/write", "read-only", "write-only"}."read-only") -> (refnum out=w2842:refnum<file>)  [unwired: 3 in, 2 out]
      n1973 = Read from Text File(file (use dialog)=w2842) -> (refnum out=w2841:refnum<file>, text=w2843:string)  [unwired: 3 in, 2 out]
      "Laser stimulus calibration" <- w2843
      n1974 = Match Pattern(string=w2843, regular expression="Max output: ") -> (after substring=w2844:string)  [unwired: 1 in, 3 out]
      n1975 = Match Pattern(string=w2843, regular expression="Min output: ") -> (after substring=w2840:string)  [unwired: 1 in, 3 out]
      n1976 = Close File(refnum=w2841) -> ()  [unwired: 1 in, 2 out]
      n1977 = Match Pattern(string=w2844, regular expression=" V") -> (before substring=w2846:string)  [unwired: 1 in, 3 out]
      n1978 = Match Pattern(string=w2840, regular expression=" V") -> (before substring=w2845:string)  [unwired: 1 in, 3 out]
      n1979 = Fract/Exp String To Number(string=w2845) -> (number=w2833:dbl)  [unwired: 3 in, 1 out]
      n1980 = Fract/Exp String To Number(string=w2846) -> (number=w2832:dbl)  [unwired: 3 in, 1 out]
      n1981 = while {
        tunnel: w2832 -> [w3318]
        tunnel: w2833 -> [w3327]
        shift-right: [w3322] -> _
        shift-left: _ -> [w3321]
        shift-right: [w3314] -> _
        shift-left: _ -> [w3315]
        stop <- w3374 stop-if-true
        w3353 = "none" ("regular expression")
        w3332 = " %" ("regular expression")
        # "safety cut off switch"
        # "Stop DAQ asistant first"
        n1982 = local read "Stim prot command"() -> (w3339:u16)
        n1983 = local read "protocol array"() -> (w3335:string[][])
        n1984 = Tick Count (ms)() -> (millisecond timer value=w3314:u32)
        n1985 = Subtract(x=w3314, y=w3315) -> (x-y=w3313:u32)
        n1986 = Divide(x=u32 1000, y=w3313) -> (x/y=→"stim loop rate":dbl)
        n1987 = Index Array(array=w3335, index (row)=w3339, index (col)=4) -> (element=w3337:string)
        n1988 = Index Array(array=w3335, index (row)=w3339, index (col)=3 ("disabled index (col)")) -> (element=w3348:string)
        n1989 = Index Array(array=w3335, index (row)=w3339, index (col)=0 ("index (row)")) -> (element=w3345:string)
        n1990 = Index Array(array=w3335, index (row)=w3339, index (col)=1 ("disabled index (col)")) -> (element=w3368:string)
        n1991 = Index Array(array=w3335, index (row)=w3339, index (col)=2 ("disabled index (col)")) -> (element=w3371:string)
        n1992 = Multiply(x="Stimulus cut off (s)", y=u32 1000) -> (x*y=w3309:u32)
        n1993 = Match Pattern(string=w3348, regular expression="int. ") -> (after substring=w3346:string)  [unwired: 1 in, 3 out]
        n1994 = local read "Track position"() -> (w3355:sgl)
        n1995 = Match Pattern(string=w3337, regular expression="duty cycle ") -> (after substring=w3333:string)  [unwired: 1 in, 3 out]
        n1996 = Match Pattern(string=w3345, regular expression="continuous") -> (match substring=w3342:string)  [unwired: 1 in, 3 out]
        n1997 = Match Pattern(string=w3345, regular expression="sinus") -> (match substring=w3341:string)  [unwired: 1 in, 3 out]
        n1998 = Match Pattern(string=w3345, regular expression="square") -> (match substring=w3340:string)  [unwired: 1 in, 3 out]
        n1999 = local read "Enable stim."() -> (w3351:bool)
        n2000 = Subtract(x=w3314, y=w3321) -> (x-y=w3320:u32)
        n2001 = Match Pattern(string=w3346, regular expression=w3332) -> (before substring=w3372:string)  [unwired: 1 in, 3 out]
        n2002 = Match Pattern(string=w3345, regular expression=" Hz") -> (before substring=w3334:string)  [unwired: 1 in, 3 out]
        n2003 = Match Pattern(string=w3345, regular expression=w3353) -> (match substring=w3352:string)  [unwired: 1 in, 3 out]
        n2004 = Match Pattern(string=w3368, regular expression="from ") -> (after substring=w3367:string)  [unwired: 1 in, 3 out]
        n2005 = Match Pattern(string=w3371, regular expression="to ") -> (after substring=w3369:string)  [unwired: 1 in, 3 out]
        n2006 = Match Pattern(string=w3333, regular expression=w3332) -> (before substring=w3331:string)  [unwired: 1 in, 3 out]
        n2007 = Concatenate Strings(w3342, w3341, w3340) -> (w3325:string)
        n2008 = Greater?(x=w3320, y=w3309) -> (0:w3319:bool)
        n2009 = Not(x=w3351) -> (.not. x?=w3350:bool)
        n2010 = Equal?(x=w3352, y=w3353) -> (x = y?=w3349:bool)
        n2011 = Decimal String To Number(string=w3372) -> (number=w3323:i32)  [unwired: 2 in, 1 out]
        n2012 = Decimal String To Number(string=w3331) -> (number=w3330:i32)  [unwired: 2 in, 1 out]
        n2013 = Decimal String To Number(string=w3334) -> (number=w3359:i32)  [unwired: 2 in, 1 out]
        n2014 = Decimal String To Number(string=w3367) -> (number=w3357:i32)  [unwired: 2 in, 1 out]
        n2015 = Decimal String To Number(string=w3369) -> (number=w3356:i32)  [unwired: 2 in, 1 out]
        n2016 = Or(x=w3350, y=w3349) -> (x .or. y?=w3354:bool)
        n2017 = case shown="False" w3354 {
          tunnel: w3357 -> [w3397 _]
          tunnel: w3355 -> [w3376 _]
          tunnel: w3356 -> [w3396 _]
          tunnel: w3355 -> [w3395 _]
          tunnel: w3325 -> [w3392 _]
          tunnel: [w3391 w3406] -> w3324
          tunnel: w3323 -> [w3389 _]
          tunnel: [w3387 w3407] -> w3317
          tunnel: w3319 -> [w3386 _]
          frame False {
            n2018 = Greater?(x=w3395, y=w3396) -> (0:w3385:bool)
            n2019 = Divide(x=w3389, y=100) -> (x/y=w3388:dbl)
            n2020 = Greater Or Equal?(x=w3376, y=w3397) -> (x >= y?=w3377:bool)
            n2021 = call "Is New Trial - stim. gen. loop.vi"("Position data"=w3376) -> ("Boolean"=w3375:bool)  [unwired: 1 in]
            n2022 = call "Is Value Changed.vim"("value"=w3377) -> ("changed or first call?"=w3380:bool)
            n2023 = call "Is Value Changed.vim"("value"=w3385) -> ("changed or first call?"=w3384:bool)
            n2024 = Compound Arithmetic op=OR(w3380, w3375) -> (w3379:bool)
            n2025 = And(x=w3385, y=w3384) -> (x .and. y?=w3383:bool)
            n2026 = Not(x=w3377) -> (.not. x?=w3378:bool)
            n2027 = Equal?(x=w3392, y="") -> (x = y?=w3394:bool)
            n2028 = Or(x=w3383, y=w3386) -> (x .or. y?=w3382:bool)
            n2029 = And(x=w3377, y=w3379) -> (x .and. y?=w3381:bool)
            n2030 = case shown="True" w3382 {
              frame False {
              }
              frame True {
                n2031 = local write "Stop light stim"(TRUE ("Stop light stim")) -> ()
              }
            }
            n2032 = case shown="True" w3378 {
              frame False {
              }
              frame True {
                n2033 = local write "Stop light stim"(TRUE ("Stop light stim")) -> ()
              }
            }
            n2034 = case shown="True" w3381 {
              frame False {
              }
              frame True {
                n2035 = local write "Start light stim"(TRUE ("Start light stim")) -> ()
                n2036 = local write "Stop light stim"(FALSE ("Stop light stim")) -> ()
              }
            }
            n2037 = case shown="False" w3394 {
              tunnel: w3392 -> [w3403 _]
              tunnel: [w3403 w3405] -> w3391
              tunnel: w3388 -> [w3402 _]
              tunnel: [w3402 w3404] -> w3387
              frame False {
                n2038 = local write "prev. max stim. V"(w3402) -> ()
                n2039 = local write "prev. stim. type"(w3403) -> ()
              }
              frame True {
                n2040 = local read "prev. stim. type"() -> (w3405:string)
                n2041 = local read "prev. max stim. V"() -> (w3404:dbl)
              }
            }
          }
          frame True {
            n2042 = local write "Stop light stim"(TRUE ("Stop light stim")) -> ()
            n2043 = local read "prev. max stim. V"() -> (w3407:dbl)
            n2044 = local read "prev. stim. type"() -> (w3406:string)
          }
        }
        n2045 = Subtract(x=w3318, y=w3327) -> (x-y=w3326:dbl)
        n2046 = local read "Start light stim"() -> (w3373:bool)
        n2047 = local read "Exit"() -> (w3329:bool)
        n2048 = Multiply(x=w3318, y=w3317) -> (x*y=w3316:dbl)
        n2049 = Multiply(x=w3326, y=w3317) -> (x*y=w3360:dbl)
        n2050 = case shown="True" w3329 {
          tunnel: [FALSE w3462] -> w3374
          frame False {
          }
          frame True {
            n2051 = local write "Enable stim."(FALSE ("Enable stim.")) -> ()
            n2052 = flat-sequence {
              tunnel: [TRUE] -> w3462
              frame #0 {
                n2053 = Wait (ms)(milliseconds to wait=u32 100) -> ()  [unwired: 1 out]
              }
              frame #1 {
              }
            }
            n2054 = property on="Enable stim." class="Bool (strict)"("DisabledEnum"=T8."Disabled and Grayed Out" ("Disabled")) -> ()  [unwired: 2 in, 2 out]
          }
        }
        n2055 = case shown="True" w3373 {
          selector: w3373 -> [w3409 w3417]
          tunnel: [w3412 w3427] -> w3328
          tunnel: w3360 -> [_ w3422]
          tunnel: w3327 -> [_ w3419]
          tunnel: w3359 -> [_ w3426]
          tunnel: w3324 -> [_ w3425]
          tunnel: w3330 -> [_ w3424]
          tunnel: [w3410 w3421] -> w3322
          tunnel: w3321 -> [_ w3421]
          tunnel: w3316 -> [_ w3420]
          frame False {
            n2056 = local read "Start mask stim"() -> (w3411:bool)
            n2057 = local write "stim started"(w3409) -> ()
            n2058 = case shown="False" w3411 {
              tunnel: [w3413 w3415] -> w3412
              frame True {
                n2059 = call "Simulate Signal77"("Offset"=0.0) -> ("DC"=w3413:dynamicdata)  [unwired: 13 in, 1 out]
              }
              frame False {
                n2060 = call "Simulate Signal8"("Offset"=0.0) -> ("DC"=w3415:dynamicdata)  [unwired: 13 in, 1 out]
              }
            }
            n2061 = Tick Count (ms)() -> (millisecond timer value=w3410:u32)
          }
          frame True {
            # "min V value"
            # "max V value"
            n2062 = local write "stim started"(w3417) -> ()
            n2063 = local read "Stop light stim"() -> (w3430:bool)
            n2064 = case shown="\"continuous\", Default" w3425 {
              tunnel: [w3433 w3440 w3447] -> w3423
              tunnel: w3422 -> [w3434 w3438 _]
              tunnel: w3426 -> [_ w3436 w3444]
              tunnel: w3424 -> [_ _ w3443]
              tunnel: w3420 -> [_ _ w3442]
              tunnel: w3419 -> [w3432 w3435 _]
              tunnel: [w3432 w3435 0.0] -> w3418
              frame "continuous", Default {
                n2065 = call "Simulate Signal78"("Offset"=w3434) -> ("Sine"=w3433:dynamicdata)  [unwired: 13 in, 1 out]
              }
              frame "sinus" {
                n2066 = Divide(x=w3438, y=2.0) -> (x/y=w3437:dbl)
                n2067 = call "Simulate Signal"("Offset"=w3437, "Frequency"=w3436, "Amplitude"=w3437) -> ("Sine"=w3440:dynamicdata)  [unwired: 11 in, 1 out]
              }
              frame "square" {
                n2068 = Divide(x=w3442, y=2.0) -> (x/y=w3445:dbl)
                n2069 = call "Simulate Signal10"("Offset"=w3445, "Duty Cycle (%)"=w3443, "Frequency"=w3444, "Amplitude"=w3445) -> ("Square"=w3447:dynamicdata)  [unwired: 10 in, 1 out]
              }
            }
            n2070 = call "Simulate Signal81"("Offset"=w3418) -> ("DC"=w3428:dynamicdata)  [unwired: 13 in, 1 out]
            n2071 = case shown="True" w3430 {
              tunnel: [w3451 w3458] -> w3431
              frame False {
                n2072 = local read "start with ramp"() -> (w3449:bool)
                n2073 = local read "start of stim"() -> (w3450:bool)
                n2074 = And(x=w3450, y=w3449) -> (x .and. y?=w3448:bool)
                n2075 = case shown="False" w3448 {
                  tunnel: [w3453 w3454] -> w3451
                  frame True {
                    n2076 = call "Simulate Signal12"() -> ("Triangle"=w3453:dynamicdata)  [unwired: 14 in, 1 out]
                    n2077 = local write "start of stim"(FALSE ("start of stim")) -> ()
                  }
                  frame False {
                    n2078 = call "Simulate Signal79"() -> ("DC"=w3454:dynamicdata)  [unwired: 14 in, 1 out]
                  }
                }
              }
              frame True {
                n2079 = call "Simulate Signal80"() -> ("Triangle"=w3458:dynamicdata)  [unwired: 14 in, 1 out]
                n2080 = local write "Stop light stim"(FALSE ("Stop light stim")) -> ()
                n2081 = local write "Start light stim"(FALSE ("Start light stim")) -> ()
                n2082 = local write "start of stim"(TRUE ("start of stim")) -> ()
              }
            }
            n2083 = Multiply(1:w3431, 2:w3423) -> (0:w3429:dynamicdata)  [unwired: 1 in, 1 out]
            n2084 = Add(1:w3428, 2:w3429) -> (0:w3427:dynamicdata)  [unwired: 1 in, 1 out]
          }
        }
        n2085 = call "DAQ Assistant"("data"=w3328, "stop (T)"=w3329) -> ()  [unwired: 16 in, 2 out]
      }
      n2086 = while {
        shift-right: [w2851] -> w2831
        shift-left: _ -> [w2853]
        shift-right: [w2850] -> w2830
        shift-left: _ -> [w2852]
        shift-right: [w2848] -> _
        shift-left: _ -> [w2847]
        stop <- w2849 stop-if-true
        n2087 = case shown="\"20 Hz until reward \"" w2847 {
          selector: w2847 -> [_ w2930 w2965 w3024 w3085 w3113 w3185 w3250]
          tunnel: w2853 -> [w2856 w2934 w2969 w3034 w3095 w3111 w3183 w3261]
          tunnel: w2852 -> [w2854 w2933 w2968 w3033 w3094 w3110 w3182 w3260]
          tunnel: [w2857 w2932 w2967 w3030 w3091 w3109 w3181 w3257] -> w2851
          tunnel: [w2855 w2931 w2966 w3029 w3090 w3108 w3180 w3256] -> w2850
          tunnel: [w2858 w2927 w2962 w3023 w3084 w3112 w3184 w3251] -> w2848
          frame "None", Default {
            n2088 = local read "Masking light"() -> (w2858:T5)
            n2089 = case shown="\"Continuous specified light off trials\"" w2858 {
              tunnel: [w2861 w2863 w2876 w2889 w2902 w2915 w2918 w2921] -> w2857
              tunnel: w2856 -> [w2861 w2865 w2878 w2891 w2904 _ _ _]
              tunnel: [w2860 w2862 w2875 w2888 w2901 w2914 w2917 w2920] -> w2855
              tunnel: w2854 -> [w2860 w2864 w2877 w2890 w2903 _ _ _]
              frame "None", Default {
              }
              frame "20 Hz until reward " {
                w2869 = 10123 items=["Finite Samples"=10178, "Continuous Samples"=10123, "Hardware Timed Single Point"=12522]  # Sample Mode
                n2090 = call <vilib>:"DAQmx Clear Task.vi"("task in"=w2865, "error in"=w2864) -> ()  [unwired: 13 in, 1 out]
                n2091 = call-poly <vilib>:"DAQmx Create Virtual Channel.vi"("frequency"=20.0, "duty cycle"=0.5 ("Duty Cycle"), "counter"=tag "Dev1/ctr3" ("Counter")) -> ("task out"=w2874:refnum<k21>, "error out"=w2873:errorcluster)  [unwired: 11 in]
                n2092 = property class="DAQmx Channel"(reference=w2874, error in=w2873, "CO.Pulse.Term"=tag "/Dev1/PFI15" ("Output Terminal")) -> (reference out=w2871:refnum<k21>, error out=w2872:errorcluster)
                n2093 = call-poly <vilib>:"DAQmx Timing.vi"("task/channels in"=w2871, "sample mode"=w2869, "error in"=w2872) -> ("task out"=w2863:refnum<k21>, "error out"=w2862:errorcluster)  [unwired: 11 in]
              }
              frame "20 Hz specified light off trials" {
                w2882 = 10123 items=["Finite Samples"=10178, "Continuous Samples"=10123, "Hardware Timed Single Point"=12522]  # Sample Mode
                n2094 = call <vilib>:"DAQmx Clear Task.vi"("task in"=w2878, "error in"=w2877) -> ()  [unwired: 13 in, 1 out]
                n2095 = call-poly <vilib>:"DAQmx Create Virtual Channel.vi"("frequency"=20.0, "duty cycle"=0.5 ("Duty Cycle"), "counter"=tag "Dev1/ctr3" ("Counter")) -> ("task out"=w2887:refnum<k21>, "error out"=w2886:errorcluster)  [unwired: 11 in]
                n2096 = property class="DAQmx Channel"(reference=w2887, error in=w2886, "CO.Pulse.Term"=tag "/Dev1/PFI15" ("Output Terminal")) -> (reference out=w2884:refnum<k21>, error out=w2885:errorcluster)
                n2097 = call-poly <vilib>:"DAQmx Timing.vi"("task/channels in"=w2884, "sample mode"=w2882, "error in"=w2885) -> ("task out"=w2876:refnum<k21>, "error out"=w2875:errorcluster)  [unwired: 11 in]
              }
              frame "20 Hz specified all trials" {
                w2895 = 10123 items=["Finite Samples"=10178, "Continuous Samples"=10123, "Hardware Timed Single Point"=12522]  # Sample Mode
                n2098 = call <vilib>:"DAQmx Clear Task.vi"("task in"=w2891, "error in"=w2890) -> ()  [unwired: 13 in, 1 out]
                n2099 = call-poly <vilib>:"DAQmx Create Virtual Channel.vi"("frequency"=20.0, "duty cycle"=0.5 ("Duty Cycle"), "counter"=tag "Dev1/ctr3" ("Counter")) -> ("task out"=w2900:refnum<k21>, "error out"=w2899:errorcluster)  [unwired: 11 in]
                n2100 = property class="DAQmx Channel"(reference=w2900, error in=w2899, "CO.Pulse.Term"=tag "/Dev1/PFI15" ("Output Terminal")) -> (reference out=w2897:refnum<k21>, error out=w2898:errorcluster)
                n2101 = call-poly <vilib>:"DAQmx Timing.vi"("task/channels in"=w2897, "sample mode"=w2895, "error in"=w2898) -> ("task out"=w2889:refnum<k21>, "error out"=w2888:errorcluster)  [unwired: 11 in]
              }
              frame "20 Hz full trial" {
                w2908 = 10123 items=["Finite Samples"=10178, "Continuous Samples"=10123, "Hardware Timed Single Point"=12522]  # Sample Mode
                n2102 = call <vilib>:"DAQmx Clear Task.vi"("task in"=w2904, "error in"=w2903) -> ()  [unwired: 13 in, 1 out]
                n2103 = call-poly <vilib>:"DAQmx Create Virtual Channel.vi"("frequency"=20.0, "duty cycle"=0.5 ("Duty Cycle"), "counter"=tag "Dev1/ctr3" ("Counter")) -> ("task out"=w2913:refnum<k21>, "error out"=w2912:errorcluster)  [unwired: 11 in]
                n2104 = property class="DAQmx Channel"(reference=w2913, error in=w2912, "CO.Pulse.Term"=tag "/Dev1/PFI15" ("Output Terminal")) -> (reference out=w2910:refnum<k21>, error out=w2911:errorcluster)
                n2105 = call-poly <vilib>:"DAQmx Timing.vi"("task/channels in"=w2910, "sample mode"=w2908, "error in"=w2911) -> ("task out"=w2902:refnum<k21>, "error out"=w2901:errorcluster)  [unwired: 11 in]
              }
              frame "Continuous specified light off trials" {
                n2106 = call-poly <vilib>:"DAQmx Create Virtual Channel.vi"("lines"=tag "Dev1/port2/line7") -> ("task out"=w2915:refnum<k21>, "error out"=w2914:errorcluster)  [unwired: 13 in]
              }
              frame "Continuous specified all trials" {
                n2107 = call-poly <vilib>:"DAQmx Create Virtual Channel.vi"("lines"=tag "Dev1/port2/line7") -> ("task out"=w2918:refnum<k21>, "error out"=w2917:errorcluster)  [unwired: 13 in]
              }
              frame "Continuous full trial" {
                n2108 = call-poly <vilib>:"DAQmx Create Virtual Channel.vi"("lines"=tag "Dev1/port2/line7") -> ("task out"=w2921:refnum<k21>, "error out"=w2920:errorcluster)  [unwired: 13 in]
              }
            }
            n2109 = Wait (ms)(milliseconds to wait=u32 20) -> ()  [unwired: 1 out]
          }
          frame "20 Hz until reward " {
            n2110 = local read "Reward given"() -> (w2925:u32)
            n2111 = Equal?(x=w2925, y=u32 0) -> (x = y?=w2923:bool)
            n2112 = case shown="True" w2923 {
              tunnel: w2934 -> [w2937 w2943]
              tunnel: w2933 -> [w2936 w2945]
              tunnel: [w2937 w2938] -> w2932
              tunnel: [w2936 w2939] -> w2931
              frame False {
                n2113 = Wait (ms)(milliseconds to wait=u32 20) -> ()  [unwired: 1 out]
              }
              frame True {
                n2114 = call <vilib>:"DAQmx Start Task.vi"("task/channels in"=w2943, "error in"=w2945) -> ("task out"=w2942:refnum<k21>, "error out"=w2944:errorcluster)  [unwired: 12 in]
                n2115 = while {
                  tunnel: w2942 -> [w2959]
                  tunnel: w2944 -> [w2958]
                  tunnel: [w2956] -> w2940
                  tunnel: [w2957] -> w2941
                  stop <- w2954 stop-if-true
                  n2116 = local read "Reward given"() -> (w2948:u32)
                  n2117 = call <vilib>:"DAQmx Is Task Done.vi"("task/channels in"=w2959, "error in"=w2958) -> ("task out"=w2957:refnum<k21>, "error out"=w2956:errorcluster)  [unwired: 11 in, 1 out]
                  n2118 = local read "Masking light"() -> (w2951:T5)
                  n2119 = local read "Exit"() -> (w2953:bool)
                  n2120 = Unbundle By Name(w2956) -> ("status"=w2952:bool)
                  n2121 = Greater?(x=w2948, y=u32 0) -> (0:w2946:bool)
                  n2122 = Not Equal?(x=w2951, y=T14."20 Hz until reward ") -> (x != y?=w2947:bool)
                  n2123 = Wait (ms)(milliseconds to wait=u32 20) -> ()  [unwired: 1 out]
                  n2124 = Compound Arithmetic op=OR(w2952, w2953, w2946, w2947) -> (w2954:bool)
                }
                n2125 = call <vilib>:"DAQmx Stop Task.vi"("task/channels in"=w2941, "error in"=w2940) -> ("task out"=w2938:refnum<k21>, "error out"=w2939:errorcluster)  [unwired: 12 in]
              }
            }
            n2126 = local read "Masking light"() -> (w2928:T5)
            n2127 = Equal?(x=w2928, y=w2930) -> (x = y?=w2929:bool)
            n2128 = Select(t=w2928, s=w2929, f=T14."None") -> (s? t:f=w2927:T5)
          }
          frame "20 Hz full trial" {
            n2129 = local read "Run experiment"() -> (w2960:bool)
            n2130 = case shown="True" w2960 {
              tunnel: w2969 -> [w2972 w2978]
              tunnel: w2968 -> [w2971 w2980]
              tunnel: [w2972 w2973] -> w2967
              tunnel: [w2971 w2974] -> w2966
              frame False {
                n2131 = Wait (ms)(milliseconds to wait=u32 20) -> ()  [unwired: 1 out]
              }
              frame True {
                n2132 = call <vilib>:"DAQmx Start Task.vi"("task/channels in"=w2978, "error in"=w2980) -> ("task out"=w2977:refnum<k21>, "error out"=w2979:errorcluster)  [unwired: 12 in]
                n2133 = while {
                  tunnel: w2977 -> [w2989]
                  tunnel: w2979 -> [w2988]
                  tunnel: [w2999] -> w2975
                  tunnel: [w3000] -> w2976
                  stop <- w2997 stop-if-true
                  n2134 = local read "stim started"() -> (w2984:bool)
                  n2135 = Equal?(x=w2984, y=TRUE) -> (x = y?=w2982:bool)
                  n2136 = call "Is Value Changed.vim"("value"=w2984) -> ("changed or first call?"=w2983:bool)
                  n2137 = And(x=w2983, y=w2982) -> (x .and. y?=w2981:bool)
                  n2138 = case shown="True" w2981 {
                    tunnel: w2989 -> [w3002 w3009]
                    tunnel: w2988 -> [w3001 w3010]
                    tunnel: [w3002 w3004] -> w2987
                    tunnel: [w3001 w3003] -> w2986
                    frame False {
                    }
                    frame True {
                      n2139 = flat-sequence {
                        tunnel: w3010 -> [w3012]
                        tunnel: w3009 -> [w3011]
                        tunnel: [w3014] -> w3008
                        tunnel: [w3013] -> w3007
                        tunnel: w3008 -> [w3017]
                        tunnel: w3007 -> [w3016]
                        tunnel: [w3017] -> w3006
                        tunnel: [w3016] -> w3005
                        tunnel: w3006 -> [w3019]
                        tunnel: w3005 -> [w3018]
                        tunnel: [w3021] -> w3004
                        tunnel: [w3020] -> w3003
                        frame #0 {
                          n2140 = call <vilib>:"DAQmx Stop Task.vi"("task/channels in"=w3011, "error in"=w3012) -> ("task out"=w3014:refnum<k21>, "error out"=w3013:errorcluster)  [unwired: 12 in]
                        }
                        frame #1 {
                          n2141 = Wait (ms)(milliseconds to wait=u32 5) -> ()  [unwired: 1 out]
                        }
                        frame #2 {
                          n2142 = call <vilib>:"DAQmx Start Task.vi"("task/channels in"=w3019, "error in"=w3018) -> ("task out"=w3021:refnum<k21>, "error out"=w3020:errorcluster)  [unwired: 12 in]
                        }
                      }
                    }
                  }
                  n2143 = local read "Run experiment"() -> (w2992:bool)
                  n2144 = local read "Masking light"() -> (w2993:T5)
                  n2145 = call <vilib>:"DAQmx Is Task Done.vi"("task/channels in"=w2987, "error in"=w2986) -> ("task out"=w3000:refnum<k21>, "error out"=w2999:errorcluster)  [unwired: 11 in, 1 out]
                  n2146 = local read "Exit"() -> (w2996:bool)
                  n2147 = Unbundle By Name(w2999) -> ("status"=w2995:bool)
                  n2148 = Not(x=w2992) -> (.not. x?=w2991:bool)
                  n2149 = Not Equal?(x=w2993, y=T5."20 Hz full trial") -> (x != y?=w2994:bool)
                  n2150 = Wait (ms)(milliseconds to wait=u32 2) -> ()  [unwired: 1 out]
                  n2151 = Compound Arithmetic op=OR(w2995, w2996, w2991, w2994) -> (w2997:bool)
                }
                n2152 = call <vilib>:"DAQmx Stop Task.vi"("task/channels in"=w2976, "error in"=w2975) -> ("task out"=w2973:refnum<k21>, "error out"=w2974:errorcluster)  [unwired: 12 in]
              }
            }
            n2153 = local read "Masking light"() -> (w2963:T5)
            n2154 = Equal?(x=w2963, y=w2965) -> (x = y?=w2964:bool)
            n2155 = Select(t=w2963, s=w2964, f=T14."None") -> (s? t:f=w2962:T5)
          }
          frame "Continuous specified light off trials" {
            n2156 = call <vilib>:"DAQmx Start Task.vi"("task/channels in"=w3034, "error in"=w3033) -> ("task out"=w3032:refnum<k21>, "error out"=w3031:errorcluster)  [unwired: 12 in]
            n2157 = disable-structure shown="Disabled" {
              disable-tunnel: w3032 -> [w3038 _]
              disable-tunnel: w3031 -> [w3037 _]
              disable-tunnel: [w3036 _] -> w3028
              disable-tunnel: [w3035 _] -> w3027
              frame Disabled {
                n2158 = while {
                  tunnel: w3038 -> [w3051]
                  tunnel: w3037 -> [w3050]
                  tunnel: [w3049] -> w3035
                  tunnel: [w3048] -> w3036
                  stop <- w3043 stop-if-true
                  n2159 = local read "VR Mode"() -> (w3045:bool)
                  n2160 = case shown="True" w3045 {
                    tunnel: [w3054 w3072] -> w3046
                    frame False {
                      n2161 = local read "prev. diode position"() -> (w3052:dbl)
                      n2162 = local read "total distance cm"() -> (w3063:sgl[])
                      n2163 = local read "total distance cm"() -> (w3064:sgl[])
                      n2164 = local read "prev. diode position"() -> (w3053:dbl)
                      n2165 = local read item#-1() -> ()  [unwired: 1 out]
                      n2166 = local read item#-1() -> ()  [unwired: 1 out]
                      n2167 = Subtract() -> (x-y=w3059:dbl)  [unwired: 2 in]
                      n2168 = Divide(x=w3059, y=2.0) -> (x/y=w3057:dbl)
                      n2169 = Absolute Value(x=w3057) -> (abs(x)=w3056:dbl)
                      n2170 = Add(y=w3056) -> (x+y=w3055:dbl)  [unwired: 1 in]
                      n2171 = Array Max & Min(array=w3063) -> (max value=w3062:sgl)  [unwired: 3 out]
                      n2172 = Array Max & Min(array=w3064) -> (max value=w3065:sgl)  [unwired: 3 out]
                      n2173 = Subtract(x=w3062, y=w3052) -> (x-y=w3061:dbl)
                      n2174 = Subtract(x=w3065, y=w3053) -> (x-y=w3066:dbl)
                      n2175 = Greater?(x=w3061) -> (0:w3060:bool)  [unwired: 1 in]
                      n2176 = case shown="True" w3060 {
                        frame False {
                        }
                        frame True {
                          n2177 = local write "Masking light"(FALSE ("Masking light")) -> ()
                        }
                      }
                      n2178 = Greater?(x=w3066) -> (0:w3068:bool)  [unwired: 1 in]
                      n2179 = Less?(x=w3066, y=w3055) -> (x < y?=w3067:bool)
                      n2180 = And(x=w3067, y=w3068) -> (x .and. y?=w3054:bool)
                    }
                    frame True {
                      n2181 = local read "Track position"() -> (w3077:sgl)
                      n2182 = local read "Track position"() -> (w3078:sgl)
                      n2183 = local read "Track position"() -> (w3074:sgl)
                      n2184 = local read item#-1() -> ()  [unwired: 1 out]
                      n2185 = local read item#-1() -> ()  [unwired: 1 out]
                      n2186 = local read item#-1() -> ()  [unwired: 1 out]
                      n2187 = Add(y=15.0) -> (x+y=w3070:dbl)  [unwired: 1 in]
                      n2188 = Less?(x=w3078, y=w3070) -> (x < y?=w3075:bool)
                      n2189 = Greater?(x=w3074) -> (0:w3073:bool)  [unwired: 1 in]
                      n2190 = Greater?(x=w3077) -> (0:w3076:bool)  [unwired: 1 in]
                      n2191 = case shown="True" w3076 {
                        frame False {
                        }
                        frame True {
                          n2192 = local write "Masking light"(FALSE ("Masking light")) -> ()
                        }
                      }
                      n2193 = And(x=w3075, y=w3073) -> (x .and. y?=w3072:bool)
                    }
                  }
                  n2194 = Wait (ms)(milliseconds to wait=u32 10) -> ()  [unwired: 1 out]
                  n2195 = local read "Masking light"() -> (w3041:T5)
                  n2196 = case shown="True" w3046 {
                    frame False {
                    }
                    frame True {
                      n2197 = local read "Light ON"() -> (w3081:bool)
                      n2198 = Not(x=w3081) -> (.not. x?=w3080:bool)
                      n2199 = case shown="True" w3080 {
                        frame False {
                        }
                        frame True {
                          n2200 = local write "Masking light"(TRUE ("Masking light")) -> ()
                        }
                      }
                    }
                  }
                  n2201 = local read "Masking light"() -> (w3044:bool)
                  n2202 = Not Equal?(x=w3041, y=T14."Continuous specified light off trials") -> (x != y?=w3040:bool)
                  n2203 = local read "Exit"() -> (w3042:bool)
                  n2204 = call-poly <vilib>:"DAQmx Write.vi"("task/channels in"=w3051, "data"=w3044, "error in"=w3050) -> ("task out"=w3049:refnum<k21>, "error out"=w3048:errorcluster)  [unwired: 10 in, 1 out]
                  n2205 = Compound Arithmetic op=OR(w3040, w3042) -> (w3043:bool)
                }
              }
              frame Enabled {
              }
            }
            n2206 = local read "Masking light"() -> (w3025:T5)
            n2207 = Equal?(x=w3025, y=w3024) -> (x = y?=w3026:bool)
            n2208 = Select(t=w3025, s=w3026, f=T14."None") -> (s? t:f=w3023:T5)
            n2209 = call <vilib>:"DAQmx Stop Task.vi"("task/channels in"=w3027, "error in"=w3028) -> ("task out"=w3030:refnum<k21>, "error out"=w3029:errorcluster)  [unwired: 12 in]
          }
          frame "Continuous full trial" {
            n2210 = call <vilib>:"DAQmx Start Task.vi"("task/channels in"=w3095, "error in"=w3094) -> ("task out"=w3093:refnum<k21>, "error out"=w3092:errorcluster)  [unwired: 12 in]
            n2211 = while {
              tunnel: w3093 -> [w3106]
              tunnel: w3092 -> [w3105]
              tunnel: [w3104] -> w3088
              tunnel: [w3103] -> w3089
              stop <- w3101 stop-if-true
              n2212 = Wait (ms)(milliseconds to wait=u32 10) -> ()  [unwired: 1 out]
              n2213 = local read "Masking light"() -> (w3099:T5)
              n2214 = local read "Run experiment"() -> (w3097:bool)
              n2215 = Not Equal?(x=w3099, y=T5."Continuous full trial") -> (x != y?=w3098:bool)
              n2216 = local read "Exit"() -> (w3100:bool)
              n2217 = call-poly <vilib>:"DAQmx Write.vi"("task/channels in"=w3106, "data"=w3097, "error in"=w3105) -> ("task out"=w3104:refnum<k21>, "error out"=w3103:errorcluster)  [unwired: 10 in, 1 out]
              n2218 = Compound Arithmetic op=OR(w3098, w3100) -> (w3101:bool)
            }
            n2219 = local read "Masking light"() -> (w3086:T5)
            n2220 = Equal?(x=w3086, y=w3085) -> (x = y?=w3087:bool)
            n2221 = Select(t=w3086, s=w3087, f=T14."None") -> (s? t:f=w3084:T5)
            n2222 = call <vilib>:"DAQmx Stop Task.vi"("task/channels in"=w3088, "error in"=w3089) -> ("task out"=w3091:refnum<k21>, "error out"=w3090:errorcluster)  [unwired: 12 in]
          }
          frame "20 Hz specified light off trials" {
            n2223 = disable-structure shown="Disabled" {
              disable-tunnel: w3111 -> [w3120 _]
              disable-tunnel: w3110 -> [w3119 _]
              disable-tunnel: [w3118 _] -> w3109
              disable-tunnel: [w3117 _] -> w3108
              frame Disabled {
                n2224 = local read "VR Mode"() -> (w3121:bool)
                n2225 = case shown="True" w3121 {
                  tunnel: [w3123 w3137] -> w3122
                  frame False {
                    n2226 = local read "total distance cm"() -> (w3129:sgl[])
                    n2227 = local read "prev. diode position"() -> (w3130:dbl)
                    n2228 = local read item#-1() -> ()  [unwired: 1 out]
                    n2229 = Subtract() -> (x-y=w3128:dbl)  [unwired: 2 in]
                    n2230 = Divide(x=w3128, y=2.0) -> (x/y=w3126:dbl)
                    n2231 = Absolute Value(x=w3126) -> (abs(x)=w3125:dbl)
                    n2232 = local read item#-1() -> ()  [unwired: 1 out]
                    n2233 = Add(y=w3125) -> (x+y=w3124:dbl)  [unwired: 1 in]
                    n2234 = Array Max & Min(array=w3129) -> (max value=w3131:sgl)  [unwired: 3 out]
                    n2235 = Subtract(x=w3131, y=w3130) -> (x-y=w3132:dbl)
                    n2236 = Greater?(x=w3132) -> (0:w3134:bool)  [unwired: 1 in]
                    n2237 = Less?(x=w3132, y=w3124) -> (x < y?=w3133:bool)
                    n2238 = And(x=w3133, y=w3134) -> (x .and. y?=w3123:bool)
                  }
                  frame True {
                    n2239 = local read "Track position"() -> (w3141:sgl)
                    n2240 = local read "Track position"() -> (w3139:sgl)
                    n2241 = local read item#-1() -> ()  [unwired: 1 out]
                    n2242 = local read item#-1() -> ()  [unwired: 1 out]
                    n2243 = Add(y=15.0) -> (x+y=w3135:dbl)  [unwired: 1 in]
                    n2244 = Less?(x=w3141, y=w3135) -> (x < y?=w3140:bool)
                    n2245 = Greater?(x=w3139) -> (0:w3138:bool)  [unwired: 1 in]
                    n2246 = And(x=w3140, y=w3138) -> (x .and. y?=w3137:bool)
                  }
                }
                n2247 = case shown="True" w3122 {
                  frame False {
                  }
                  frame True {
                    n2248 = local read "Light ON"() -> (w3143:bool)
                    n2249 = Not(x=w3143) -> (.not. x?=w3142:bool)
                    n2250 = case shown="True" w3142 {
                      frame False {
                      }
                      frame True {
                        n2251 = local write "Masking light"(TRUE ("Masking light")) -> ()
                      }
                    }
                  }
                }
                n2252 = local read "Masking light"() -> (w3116:bool)
                n2253 = case shown="True" w3116 {
                  tunnel: w3120 -> [w3147 w3153]
                  tunnel: w3119 -> [w3146 w3155]
                  tunnel: [w3147 w3148] -> w3118
                  tunnel: [w3146 w3149] -> w3117
                  frame False {
                    n2254 = Wait (ms)(milliseconds to wait=u32 20) -> ()  [unwired: 1 out]
                  }
                  frame True {
                    n2255 = call <vilib>:"DAQmx Start Task.vi"("task/channels in"=w3153, "error in"=w3155) -> ("task out"=w3152:refnum<k21>, "error out"=w3154:errorcluster)  [unwired: 12 in]
                    n2256 = while {
                      tunnel: w3152 -> [w3169]
                      tunnel: w3154 -> [w3168]
                      tunnel: [w3166] -> w3150
                      tunnel: [w3167] -> w3151
                      stop <- w3164 stop-if-true
                      n2257 = local read "VR Mode"() -> (w3156:bool)
                      n2258 = case shown="True" w3156 {
                        frame False {
                          n2259 = local read "prev. diode position"() -> (w3170:dbl)
                          n2260 = local read "total distance cm"() -> (w3174:sgl[])
                          n2261 = local read item#-1() -> ()  [unwired: 1 out]
                          n2262 = Array Max & Min(array=w3174) -> (max value=w3173:sgl)  [unwired: 3 out]
                          n2263 = Subtract(x=w3173, y=w3170) -> (x-y=w3172:dbl)
                          n2264 = Greater?(x=w3172) -> (0:w3171:bool)  [unwired: 1 in]
                          n2265 = case shown="True" w3171 {
                            frame False {
                            }
                            frame True {
                              n2266 = local write "Masking light"(FALSE ("Masking light")) -> ()
                            }
                          }
                        }
                        frame True {
                          n2267 = local read "Track position"() -> (w3177:sgl)
                          n2268 = local read item#-1() -> ()  [unwired: 1 out]
                          n2269 = Greater?(x=w3177) -> (0:w3176:bool)  [unwired: 1 in]
                          n2270 = case shown="True" w3176 {
                            frame False {
                            }
                            frame True {
                              n2271 = local write "Masking light"(FALSE ("Masking light")) -> ()
                            }
                          }
                        }
                      }
                      n2272 = call <vilib>:"DAQmx Is Task Done.vi"("task/channels in"=w3169, "error in"=w3168) -> ("task out"=w3167:refnum<k21>, "error out"=w3166:errorcluster)  [unwired: 11 in, 1 out]
                      n2273 = local read "Masking light"() -> (w3158:bool)
                      n2274 = local read "Masking light"() -> (w3160:T5)
                      n2275 = Unbundle By Name(w3166) -> ("status"=w3162:bool)
                      n2276 = local read "Exit"() -> (w3163:bool)
                      n2277 = Not(x=w3158) -> (.not. x?=w3157:bool)
                      n2278 = Not Equal?(x=w3160, y=T14."20 Hz specified light off trials") -> (x != y?=w3161:bool)
                      n2279 = Compound Arithmetic op=OR(w3162, w3163, w3157, w3161) -> (w3164:bool)
                      n2280 = Wait (ms)(milliseconds to wait=u32 20) -> ()  [unwired: 1 out]
                    }
                    n2281 = call <vilib>:"DAQmx Stop Task.vi"("task/channels in"=w3151, "error in"=w3150) -> ("task out"=w3148:refnum<k21>, "error out"=w3149:errorcluster)  [unwired: 12 in]
                  }
                }
              }
              frame Enabled {
              }
            }
            n2282 = local read "Masking light"() -> (w3114:T5)
            n2283 = Equal?(x=w3114, y=w3113) -> (x = y?=w3115:bool)
            n2284 = Select(t=w3114, s=w3115, f=T14."None") -> (s? t:f=w3112:T5)
          }
          frame "20 Hz specified all trials" {
            n2285 = disable-structure shown="Disabled" {
              disable-tunnel: w3183 -> [w3192 _]
              disable-tunnel: w3182 -> [w3191 _]
              disable-tunnel: [w3190 _] -> w3181
              disable-tunnel: [w3189 _] -> w3180
              frame Disabled {
                n2286 = local read "VR Mode"() -> (w3193:bool)
                n2287 = case shown="True" w3193 {
                  tunnel: [w3196 w3209] -> w3194
                  frame False {
                    n2288 = local read "total distance cm"() -> (w3202:sgl[])
                    n2289 = local read "prev. diode position"() -> (w3195:dbl)
                    n2290 = local read item#-1() -> ()  [unwired: 1 out]
                    n2291 = Subtract() -> (x-y=w3201:dbl)  [unwired: 2 in]
                    n2292 = Divide(x=w3201, y=2.0) -> (x/y=w3199:dbl)
                    n2293 = Absolute Value(x=w3199) -> (abs(x)=w3198:dbl)
                    n2294 = local read item#-1() -> ()  [unwired: 1 out]
                    n2295 = Add(y=w3198) -> (x+y=w3197:dbl)  [unwired: 1 in]
                    n2296 = Array Max & Min(array=w3202) -> (max value=w3203:sgl)  [unwired: 3 out]
                    n2297 = Subtract(x=w3203, y=w3195) -> (x-y=w3204:dbl)
                    n2298 = Greater?(x=w3204) -> (0:w3206:bool)  [unwired: 1 in]
                    n2299 = Less?(x=w3204, y=w3197) -> (x < y?=w3205:bool)
                    n2300 = And(x=w3205, y=w3206) -> (x .and. y?=w3196:bool)
                  }
                  frame True {
                    n2301 = local read "Track position"() -> (w3213:sgl)
                    n2302 = local read "Track position"() -> (w3211:sgl)
                    n2303 = local read item#-1() -> ()  [unwired: 1 out]
                    n2304 = local read item#-1() -> ()  [unwired: 1 out]
                    n2305 = Add(y=15.0) -> (x+y=w3207:dbl)  [unwired: 1 in]
                    n2306 = Less?(x=w3213, y=w3207) -> (x < y?=w3212:bool)
                    n2307 = Greater?(x=w3211) -> (0:w3210:bool)  [unwired: 1 in]
                    n2308 = And(x=w3212, y=w3210) -> (x .and. y?=w3209:bool)
                  }
                }
                n2309 = case shown="True" w3194 {
                  frame False {
                  }
                  frame True {
                    n2310 = local write "Masking light"(TRUE ("Masking light")) -> ()
                  }
                }
                n2311 = local read "Masking light"() -> (w3188:bool)
                n2312 = case shown="True" w3188 {
                  tunnel: w3192 -> [w3217 w3223]
                  tunnel: w3191 -> [w3216 w3225]
                  tunnel: [w3217 w3218] -> w3190
                  tunnel: [w3216 w3219] -> w3189
                  frame False {
                    n2313 = Wait (ms)(milliseconds to wait=u32 20) -> ()  [unwired: 1 out]
                  }
                  frame True {
                    n2314 = call <vilib>:"DAQmx Start Task.vi"("task/channels in"=w3223, "error in"=w3225) -> ("task out"=w3222:refnum<k21>, "error out"=w3224:errorcluster)  [unwired: 12 in]
                    n2315 = while {
                      tunnel: w3222 -> [w3239]
                      tunnel: w3224 -> [w3238]
                      tunnel: [w3236] -> w3220
                      tunnel: [w3237] -> w3221
                      stop <- w3234 stop-if-true
                      n2316 = local read "VR Mode"() -> (w3226:bool)
                      n2317 = case shown="True" w3226 {
                        frame False {
                          n2318 = local read "prev. diode position"() -> (w3240:dbl)
                          n2319 = local read "total distance cm"() -> (w3244:sgl[])
                          n2320 = local read item#-1() -> ()  [unwired: 1 out]
                          n2321 = Array Max & Min(array=w3244) -> (max value=w3243:sgl)  [unwired: 3 out]
                          n2322 = Subtract(x=w3243, y=w3240) -> (x-y=w3242:dbl)
                          n2323 = Greater?(x=w3242) -> (0:w3241:bool)  [unwired: 1 in]
                          n2324 = case shown="True" w3241 {
                            frame False {
                            }
                            frame True {
                              n2325 = local write "Masking light"(FALSE ("Masking light")) -> ()
                            }
                          }
                        }
                        frame True {
                          n2326 = local read "Track position"() -> (w3247:sgl)
                          n2327 = local read item#-1() -> ()  [unwired: 1 out]
                          n2328 = Greater?(x=w3247) -> (0:w3246:bool)  [unwired: 1 in]
                          n2329 = case shown="True" w3246 {
                            frame False {
                            }
                            frame True {
                              n2330 = local write "Masking light"(FALSE ("Masking light")) -> ()
                            }
                          }
                        }
                      }
                      n2331 = call <vilib>:"DAQmx Is Task Done.vi"("task/channels in"=w3239, "error in"=w3238) -> ("task out"=w3237:refnum<k21>, "error out"=w3236:errorcluster)  [unwired: 11 in, 1 out]
                      n2332 = local read "Masking light"() -> (w3228:bool)
                      n2333 = local read "Masking light"() -> (w3230:T5)
                      n2334 = Unbundle By Name(w3236) -> ("status"=w3232:bool)
                      n2335 = local read "Exit"() -> (w3233:bool)
                      n2336 = Not(x=w3228) -> (.not. x?=w3227:bool)
                      n2337 = Not Equal?(x=w3230, y=T14."20 Hz specified all trials") -> (x != y?=w3231:bool)
                      n2338 = Compound Arithmetic op=OR(w3232, w3233, w3227, w3231) -> (w3234:bool)
                      n2339 = Wait (ms)(milliseconds to wait=u32 20) -> ()  [unwired: 1 out]
                    }
                    n2340 = call <vilib>:"DAQmx Stop Task.vi"("task/channels in"=w3221, "error in"=w3220) -> ("task out"=w3218:refnum<k21>, "error out"=w3219:errorcluster)  [unwired: 12 in]
                  }
                }
              }
              frame Enabled {
              }
            }
            n2341 = local read "Masking light"() -> (w3186:T5)
            n2342 = Equal?(x=w3186, y=w3185) -> (x = y?=w3187:bool)
            n2343 = Select(t=w3186, s=w3187, f=T14."None") -> (s? t:f=w3184:T5)
          }
          frame "Continuous specified all trials" {
            n2344 = call <vilib>:"DAQmx Start Task.vi"("task/channels in"=w3261, "error in"=w3260) -> ("task out"=w3259:refnum<k21>, "error out"=w3258:errorcluster)  [unwired: 12 in]
            n2345 = disable-structure shown="Disabled" {
              disable-tunnel: w3259 -> [w3265 _]
              disable-tunnel: w3258 -> [w3264 _]
              disable-tunnel: [w3263 _] -> w3255
              disable-tunnel: [w3262 _] -> w3254
              frame Disabled {
                n2346 = while {
                  tunnel: w3265 -> [w3278]
                  tunnel: w3264 -> [w3277]
                  tunnel: [w3276] -> w3262
                  tunnel: [w3275] -> w3263
                  stop <- w3267 stop-if-true
                  n2347 = local read "VR Mode"() -> (w3272:bool)
                  n2348 = case shown="True" w3272 {
                    tunnel: [w3281 w3299] -> w3273
                    frame False {
                      n2349 = local read "prev. diode position"() -> (w3279:dbl)
                      n2350 = local read "total distance cm"() -> (w3290:sgl[])
                      n2351 = local read "total distance cm"() -> (w3291:sgl[])
                      n2352 = local read item#-1() -> ()  [unwired: 1 out]
                      n2353 = local read "prev. diode position"() -> (w3280:dbl)
                      n2354 = local read item#-1() -> ()  [unwired: 1 out]
                      n2355 = Subtract() -> (x-y=w3286:dbl)  [unwired: 2 in]
                      n2356 = Divide(x=w3286, y=2.0) -> (x/y=w3284:dbl)
                      n2357 = Absolute Value(x=w3284) -> (abs(x)=w3283:dbl)
                      n2358 = Add(y=w3283) -> (x+y=w3282:dbl)  [unwired: 1 in]
                      n2359 = Array Max & Min(array=w3290) -> (max value=w3289:sgl)  [unwired: 3 out]
                      n2360 = Array Max & Min(array=w3291) -> (max value=w3292:sgl)  [unwired: 3 out]
                      n2361 = Subtract(x=w3289, y=w3279) -> (x-y=w3288:dbl)
                      n2362 = Subtract(x=w3292, y=w3280) -> (x-y=w3293:dbl)
                      n2363 = Greater?(x=w3288) -> (0:w3287:bool)  [unwired: 1 in]
                      n2364 = case shown="True" w3287 {
                        frame False {
                        }
                        frame True {
                          n2365 = local write "Masking light"(FALSE ("Masking light")) -> ()
                        }
                      }
                      n2366 = Greater?(x=w3293) -> (0:w3295:bool)  [unwired: 1 in]
                      n2367 = Less?(x=w3293, y=w3282) -> (x < y?=w3294:bool)
                      n2368 = And(x=w3294, y=w3295) -> (x .and. y?=w3281:bool)
                    }
                    frame True {
                      n2369 = local read "Track position"() -> (w3304:sgl)
                      n2370 = local read "Track position"() -> (w3305:sgl)
                      n2371 = local read "Track position"() -> (w3301:sgl)
                      n2372 = local read item#-1() -> ()  [unwired: 1 out]
                      n2373 = local read item#-1() -> ()  [unwired: 1 out]
                      n2374 = local read item#-1() -> ()  [unwired: 1 out]
                      n2375 = Add(y=15.0) -> (x+y=w3297:dbl)  [unwired: 1 in]
                      n2376 = Less?(x=w3305, y=w3297) -> (x < y?=w3302:bool)
                      n2377 = Greater?(x=w3301) -> (0:w3300:bool)  [unwired: 1 in]
                      n2378 = Greater?(x=w3304) -> (0:w3303:bool)  [unwired: 1 in]
                      n2379 = case shown="True" w3303 {
                        frame False {
                        }
                        frame True {
                          n2380 = local write "Masking light"(FALSE ("Masking light")) -> ()
                        }
                      }
                      n2381 = And(x=w3302, y=w3300) -> (x .and. y?=w3299:bool)
                    }
                  }
                  n2382 = Wait (ms)(milliseconds to wait=u32 10) -> ()  [unwired: 1 out]
                  n2383 = local read "Masking light"() -> (w3269:T5)
                  n2384 = case shown="True" w3273 {
                    frame False {
                    }
                    frame True {
                      n2385 = local write "Masking light"(TRUE ("Masking light")) -> ()
                    }
                  }
                  n2386 = local read "Masking light"() -> (w3271:bool)
                  n2387 = Not Equal?(x=w3269, y=T14."Continuous specified all trials") -> (x != y?=w3268:bool)
                  n2388 = local read "Exit"() -> (w3270:bool)
                  n2389 = call-poly <vilib>:"DAQmx Write.vi"("task/channels in"=w3278, "data"=w3271, "error in"=w3277) -> ("task out"=w3276:refnum<k21>, "error out"=w3275:errorcluster)  [unwired: 10 in, 1 out]
                  n2390 = Compound Arithmetic op=OR(w3268, w3270) -> (w3267:bool)
                }
              }
              frame Enabled {
              }
            }
            n2391 = local read "Masking light"() -> (w3252:T5)
            n2392 = Equal?(x=w3252, y=w3250) -> (x = y?=w3253:bool)
            n2393 = Select(t=w3252, s=w3253, f=T14."None") -> (s? t:f=w3251:T5)
            n2394 = call <vilib>:"DAQmx Stop Task.vi"("task/channels in"=w3254, "error in"=w3255) -> ("task out"=w3257:refnum<k21>, "error out"=w3256:errorcluster)  [unwired: 12 in]
          }
        }
        n2395 = local read "Exit"() -> (w2849:bool)
      }
      n2396 = call <vilib>:"DAQmx Clear Task.vi"("task in"=w2831, "error in"=w2830) -> ()  [unwired: 13 in, 1 out]
    }
  }
  n2397 = Bundle(w7, w7) -> (w6:cluster{i32, i32})  [unwired: 1 in]
  n2398 = property on="Saved pupil imaging signals" class="Tbl (strict)"("Index Values"=w6) -> ()  [unwired: 2 in, 2 out]
  n2399 = property on="Behavior and VR signals saved" class="Tbl (strict)"("Index Values"=w6) -> ()  [unwired: 2 in, 2 out]
  n2400 = property on="Saved 2P signals" class="Tbl (strict)"("Index Values"=w6) -> ()  [unwired: 2 in, 2 out]
  n2401 = property on="Saved optogen. signals" class="Tbl (strict)"("Index Values"=w6) -> ()  [unwired: 2 in, 2 out]
  n2402 = local write "Reset bottom plot"(w44) -> ()
  n2403 = local write "Reset wheel pos. graph"(w44) -> ()
  n2404 = local write "Reset top plot"(w44) -> ()
  n2405 = local write "Random reward"(FALSE ("Random reward")) -> ()
  n2406 = disable-structure shown="Disabled" {
    disable-tunnel: _ -> [w3465 _]
    frame Disabled {
      n2407 = case shown="True" w3465 {
        frame False {
        }
        frame True {
          # "Light ON/OFF  indicators"
          # "Trial type indicators"
          n2408 = local read "shuffled array"() -> (w3472:i16[])
          n2409 = local read "All trials"() -> (w3473:i32)
          n2410 = local read "shuffled array"() -> (w3525:i16[])
          n2411 = local read "shuffled array"() -> (w3480:i16[])
          n2412 = local read "Stim types"() -> (w3526:u16[])
          n2413 = local read "Stim types"() -> (w3479:u16[])
          n2414 = local read "Stim types"() -> (w3470:u16[])
          n2415 = Quotient & Remainder(x=w3473, y=5.0) -> (x-y*floor(x/y)=w3471:dbl)  [unwired: 1 out]
          n2416 = Index Array(array=w3472, index=w3471) -> (element=w3469:i16)
          n2417 = Index Array(array=w3526, index=0 ("index (row)")) -> (element=w3519:u16)
          n2418 = Index Array(array=w3479, index=1 ("index (row)")) -> (element=w3486:u16)
          n2419 = Index Array(array=w3525, index=0) -> (element=w3524:i16)
          n2420 = Index Array(array=w3525, index=1) -> (element=w3520:i16)
          n2421 = Index Array(array=w3525, index=2) -> (element=w3521:i16)
          n2422 = Index Array(array=w3525, index=3) -> (element=w3522:i16)
          n2423 = Index Array(array=w3525, index=4) -> (element=w3523:i16)
          n2424 = Index Array(array=w3480, index=0) -> (element=w3481:i16)
          n2425 = Index Array(array=w3480, index=1) -> (element=w3485:i16)
          n2426 = Index Array(array=w3480, index=2) -> (element=w3484:i16)
          n2427 = Index Array(array=w3480, index=3) -> (element=w3483:i16)
          n2428 = Index Array(array=w3480, index=4) -> (element=w3482:i16)
          n2429 = Index Array(array=w3470, index (row)=0, index (col)=w3469) -> (element=w3466:u16)
          n2430 = Index Array(array=w3519, index=w3524) -> (element=w3518)
          n2431 = Index Array(array=w3519, index=w3520) -> (element=w3517)
          n2432 = Index Array(array=w3519, index=w3521) -> (element=w3516)
          n2433 = Index Array(array=w3519, index=w3522) -> (element=w3514)
          n2434 = Index Array(array=w3519, index=w3523) -> (element=w3515)
          n2435 = Index Array(array=w3486, index=w3481) -> (element=w3487)
          n2436 = Index Array(array=w3486, index=w3485) -> (element=w3488)
          n2437 = Index Array(array=w3486, index=w3484) -> (element=w3489)
          n2438 = Index Array(array=w3486, index=w3483) -> (element=w3491)
          n2439 = Index Array(array=w3486, index=w3482) -> (element=w3490)
          n2440 = Number To Boolean Array(number=w3466) -> (Boolean array=w3534:bool[])
          n2441 = Number To Boolean Array(number=w3518) -> (Boolean array=w3527:bool[])
          n2442 = Number To Boolean Array(number=w3516) -> (Boolean array=w3530:bool[])
          n2443 = Number To Boolean Array(number=w3514) -> (Boolean array=w3529:bool[])
          n2444 = Number To Boolean Array(number=w3515) -> (Boolean array=w3531:bool[])
          n2445 = Number To Boolean Array(number=w3487) -> (Boolean array=w3478:bool[])
          n2446 = Number To Boolean Array(number=w3489) -> (Boolean array=w3475:bool[])
          n2447 = Number To Boolean Array(number=w3491) -> (Boolean array=w3476:bool[])
          n2448 = Number To Boolean Array(number=w3490) -> (Boolean array=w3474:bool[])
          n2449 = Number To Boolean Array(number=w3517) -> (Boolean array=w3528:bool[])
          n2450 = Number To Boolean Array(number=w3488) -> (Boolean array=w3477:bool[])
          n2451 = Index Array(array=w3534, index=0) -> (element=w3533:bool)
          n2452 = Index Array(array=w3527, index=0) -> ()  [unwired: 1 out]
          n2453 = Index Array(array=w3528, index=0) -> ()  [unwired: 1 out]
          n2454 = Index Array(array=w3530, index=0) -> ()  [unwired: 1 out]
          n2455 = Index Array(array=w3529, index=0) -> ()  [unwired: 1 out]
          n2456 = Index Array(array=w3531, index=0) -> ()  [unwired: 1 out]
          n2457 = Index Array(array=w3478, index=0) -> ()  [unwired: 1 out]
          n2458 = Index Array(array=w3477, index=0) -> ()  [unwired: 1 out]
          n2459 = Index Array(array=w3475, index=0) -> ()  [unwired: 1 out]
          n2460 = Index Array(array=w3476, index=0) -> ()  [unwired: 1 out]
          n2461 = Index Array(array=w3474, index=0) -> ()  [unwired: 1 out]
          n2462 = local read item#-1() -> ()  [unwired: 1 in]
          n2463 = local read item#-1() -> ()  [unwired: 1 in]
          n2464 = local read item#-1() -> ()  [unwired: 1 in]
          n2465 = local read item#-1() -> ()  [unwired: 1 in]
          n2466 = local read item#-1() -> ()  [unwired: 1 in]
          n2467 = local read item#-1() -> ()  [unwired: 1 in]
          n2468 = local read item#-1() -> ()  [unwired: 1 in]
          n2469 = local read item#-1() -> ()  [unwired: 1 in]
          n2470 = local read item#-1() -> ()  [unwired: 1 in]
          n2471 = local read item#-1() -> ()  [unwired: 1 in]
        }
      }
    }
    frame Enabled {
    }
  }
  n2472 = disable-structure shown="Disabled" {
    frame Disabled {
      n2473 = local read "No. of smpl. per ch."() -> (w3540:i32)
      n2474 = local read "Photodiode signal"() -> (w3552:sgl[])
      n2475 = local read "Track position"() -> (w3541:sgl)
      n2476 = local read "Valve signal"() -> (w3551:i8[])
      n2477 = local read "lick signal"() -> (w3550:i8[])
      n2478 = local read "analog lick"() -> (w3549:sgl[])
      n2479 = local read "VR Gain"() -> (w3539:dbl)
      n2480 = local read "Frame signal"() -> (w3548:i8[])
      n2481 = local read "Frame signal 2"() -> (w3547:i8[])
      n2482 = local read "Eye cam frame signal"() -> (w3546:i8[])
      n2483 = local read "Analog 3"() -> (w3545:sgl[])
      n2484 = local read "Photo stimulus signal"() -> (w3544:sgl[])
      n2485 = local read "ML signal"() -> (w3543:sgl[])
      n2486 = local read "Analog 5"() -> (w3542:sgl[])
      n2487 = local read "delta time (s)"() -> (w3536:dbl)
      n2488 = Multiply(x=w3536, y=1000.0) -> ()  [unwired: 1 out]
      n2489 = Initialize Array(w3541, w3540) -> (w3537:sgl[])
      n2490 = Initialize Array(w3539, w3540) -> (w3538:dbl[])
      n2491 = Build Array(w3552, w3537, w3551, w3550, w3549, w3538, w3548, w3547, w3546, w3545, w3544, w3543, w3542) -> ()  [unwired: 1 out]
    }
    frame Enabled {
    }
  }
  "Tab Control hidden Variables" <- enum32{"Test charts", "Variables"}."Test charts" ("Tab Control 5")
